vi "IMAQController.panel.vi"(0 "object ref":refnum<vi>, 5 "error in":errorcluster) -> ()   [LabVIEW 2014, in "IMAQController.lvlib"]
doc: "This is the front panel VI for the IMAQController class.\n\nThis program is free software; you can redistribute it and/or modify it under the terms of the GNU General Public License as published by the Free Software Foundation; either version 2 of the license, or (at your option) any later version.\n\nThis program is distributed in the hope that it will be useful, but WITHOUT ANY WARRANTY; without even the implied warranty of MERCHANTABILITY or FITNESS FOR A PARTICULAR PURPOSE. See the GNU General License for more details (http://www.gnu.org).\n\nLast update: 2-DEC-2010"
uses:
  IMAQController.lvlib
  CSlibraries-extern/DimLVEvent/LVDimInterface/LVDimInterface.lvlib
  CSlibraries-extern/DimLVEvent/LVDimInterface/LVDimInterface.dim service type.ctl
  CSCore/CSSystem/CSSystemLib/CSSystemLib.lvlib
  CSCore/BaseProcess/BaseProcess.lvlib
  CSlibraries-extern/DimLVEvent/DimIndicators/DimIndicators.lvlib
  CSPentatrap/_common/PTUtils/PTUtils.lvlib
  CSlibraries-extern/HGF/HGF_VisionTools/HGF_VisionTools.lvlib
  CSCore/CSObj/CSObj.lvlib
  CSlibraries-extern/DimLVEvent/LVDimInterface/LVDimInterface.dic_info_service_queue.vi
  CSCore/CSSystem/CoreLib/CoreLib.lvlib
  CSCore/CSSystem/CoreLib/CoreLib.short 2 byte array.vi
  <vilib>/Utility/error.llb/DialogType.ctl
  CSCore/CSSystem/CoreLib/CoreLib.int 2 byte array.vi
  CSCore/CSSystem/CoreLib/CoreLib.string 2 byte array.vi
  <vilib>/Utility/file.llb/Write To Spreadsheet File (DBL).vi
  <vilib>/Math Plots/3D Math Plots/3D Surface/3D Surface Datatype/3D Surface Datatype.lvclass
  <vilib>/Utility/file.llb/Write To Spreadsheet File (I64).vi
  <vilib>/Math Plots/3D Math Plots/3D Surface/3D Surface XCtrl/3D Surface.xctl
  <vilib>/Utility/config.llb/NI_LVConfig.lvlib
  <vilib>/Utility/config.llb/Read Key (Boolean).vi
  <vilib>/Utility/config.llb/Read Key (String).vi
  <vilib>/Utility/config.llb/Write Key (String).vi
  <vilib>/Math Plots/3D Math Plots/3D Surface/3D Surface Datatype/Public/Plot Helper (Vector).vi
  <vilib>/Math Plots/3D Math Plots/3D Plot/3D Plot Datatype/3D Plot Datatype.lvclass
  <vilib>/Utility/config.llb/Write Key (Boolean).vi
  <vilib>/event_ctls.llb/eventvkey.ctl
  CSlibraries-extern/DimLVEvent/DimIndicators/DimIndicators.anyType.ctl
panel:
  in  "ScanNamesArray":string[](array[string])
  in  "MeasurementNo":i32
  out "AnaWidth":i32
  out "AnaHeight":i32
  out "ScanRunning?":bool
  out "Progress bar":u8(slide) scale=0.0..100.0
  out "Last scan started":string
  out "ScanMin":dbl
  out "ActVerticalProj":dbl[][](array[numeric])
  out "ActHorizontalProj":dbl[][](array[numeric])
  in  "Delay (ms) Buffered":i32=2000
  out "SActStep":i32
  in  "Control Tab":T1(tab)
  in  "ROI Choice":enum32{"Radio Selection 1", "Radio Selection 2"}(radio)=enum."Radio Selection 2"
  in  "lower limit":dbl
  in  "auto repeat scan step":bool
  in  "Stop Scan button":bool
  in  "Pause Scan button":bool
  in  "Start Scan button":bool
  in  "Configure Scan button":bool
  in  "ROI2notROI1Boolen":bool
  in  "TL1x":i32 caption="x"
  in  "TL1y":i32 caption="y"
  in  "BR1x":i32 caption="x"
  in  "BR1y":i32 caption="y"
  in  "TL2x":i32 caption="x"
  in  "TL2y":i32 caption="y"
  in  "BR2x":i32 caption="x"
  in  "BR2y":i32 caption="y"
  in  "Clear ROIs button":bool
  out "ROI 2":dbl format="%.0e"
  out "ROI 1":dbl format="%.0e"
  out "ROI 1 / ROI 2":dbl format="%#.4g"
  in  "Offset":dbl
  in  "auto save":bool
  in  "Delay (ms)":i32=2000
  in  "Acquisition mode":T2(radio)
  in  "Network Transport":enum32{"Radio Selection 1", "Radio Selection 2"}(radio)
  in  "Image Settings":cluster{u8, u8}(slide)={0, 255} scale=0.0..255.0
  in  "Show Grid ?":bool=TRUE
  in  "Grid Color Box":u32(colorbox)=16448250
  in  "Save Path":path=path "D:/HitrapControlSystem/Camera-Pictures"
  in  "Overlay configured?":bool
  in  "Save this button":bool
  in  "Averaging":u8=1
  in  "Show all data":bool=TRUE
  in  "# shown Plots:":u8=3
  out "Intensity Scan":cluster{dbl[], dbl[]}[](graph)
  out "3D Surface":refnum<class "3D Plot Datatype.lvclass">[](xcontrol)
  out "ScanImage":T3(plugin-control)
  out "HilfsplotProj":cluster{i32[], dbl[]}[](graph)
  in  "Save Analysis button":bool
  in  "Analysis Mode":T4(ring)
  in  "Clear Analysis button":bool
  in  "Bug Report/ Feature Request - List":i32(listbox)
  in  "Send Button":bool
  out "Error OR":bool
  out "Error OL":bool
  out "Error UR":bool
  out "Error UL":bool
  out "Camera Choice error out":errorcluster
  out "NewVal":i32[](array[numeric])
  out "Overlay Lines":T5(array[cluster])
  out "SNofSteps":i32
  out "Image Arrived":i32
  out "Scan Image":i32
  out "Proj Up":i32
  out "AnaStep2":string
  out "AnaStep1":string
  out "AnaStep3":string
  out "BugFilePath":path
  out "ActDimensions":i16
  out "ScanValuesArray":dbl[](array[numeric])
  in  "CameraTimeStamps":dbl[](array[numeric])
  out "DIM Array":refnum<queue>[](array[refnum])
  out "Connection status":bool
  in  "Camera Choice":i32[](listbox)
  in  "Select Camera":u16(ring)
  in  "Camera\nConnected?":bool
  in  "Acquisition mode (Buffer)":T2(radio)
  in  "string":string
  in  "TestButton":bool
  out "ActImage RSelectionOn?":bool
  out "ActImage RMouse Down?":bool
  out "ActImage LSelectionOn?":bool
  out "ActImage LMouse Down?":bool
  out "Vertical chart XY":cluster{i32[], dbl[]}[](graph)
  out "Horizontal chart XY":cluster{i32[], dbl[]}[](graph)
  out "Error complete":bool
  out "Horizontal chart":dbl(graph)
  out "Time Stamp":timestamp format="%<%X\n%x>T"
  in  "Clear Log button":bool
  in  "Save Log button":bool
  in  "ActualImageLink(Compression Mode)":T6
  in  "Chart Auswertung-Strings":string
  out "Horiz/Vert Chart error out":errorcluster
  out "Horiz/Vert Chart Loop":i32
  out "Vertical chart":dbl[][](graph)
  out "Waveform Chart":dbl(graph)
  out "Act Image\nInformation":string
  out "Scan Image Pixel Value Loop error out":errorcluster
  out "Scan Pixel Value Loop":i32
  out "Scan Image\nInformation":string
  in  "stop button":bool
  out "Logger String":string
  out "Time Loop":i32
  in  "Analysis Image Settings":cluster{u8, u8}(slide)={0, 255} scale=0.0..255.0
  out "User Event error out":errorcluster
  out "User Event Loop":i32
  out "Send command error out":errorcluster
  out "DIM client error out":errorcluster
  out "Send Command Loop":i32
  out "DIM Client Loop":i32
  out "Analysis Event Loop":i32
  out "Asynch\nAna Data":i32
  out "TimeStamp Analyzer":i16[](array[numeric])
  out "Data Ana Synch?":bool
  out "TimeStamp Data":i16[](array[numeric])
  out "aktueller\nService":i32
  out "Image length":i32
  out "Image height":i32
  out "ActImage":T3(plugin-control)
  out "Analysis Event error out":errorcluster
  out "DIM service length / byte":i32
  out "no link":bool
  out "callBackID":i32
  # "Acquisition control"
  # "Scan control"
  # "Projections control"
  # "Image control"
  # "ROI 1"
  # "ROI 2"
  # "TL"
  # "BR"
  # "Integrated Pixel Values"
  # "Save Path"
  # "(no Analysis!)"
  # "Intensity Plot"
  # "Intensity Plot"
  # "Vertical Projection"
  # "position / mm"
  # "Horizontal Projection"
  # "position / mm"
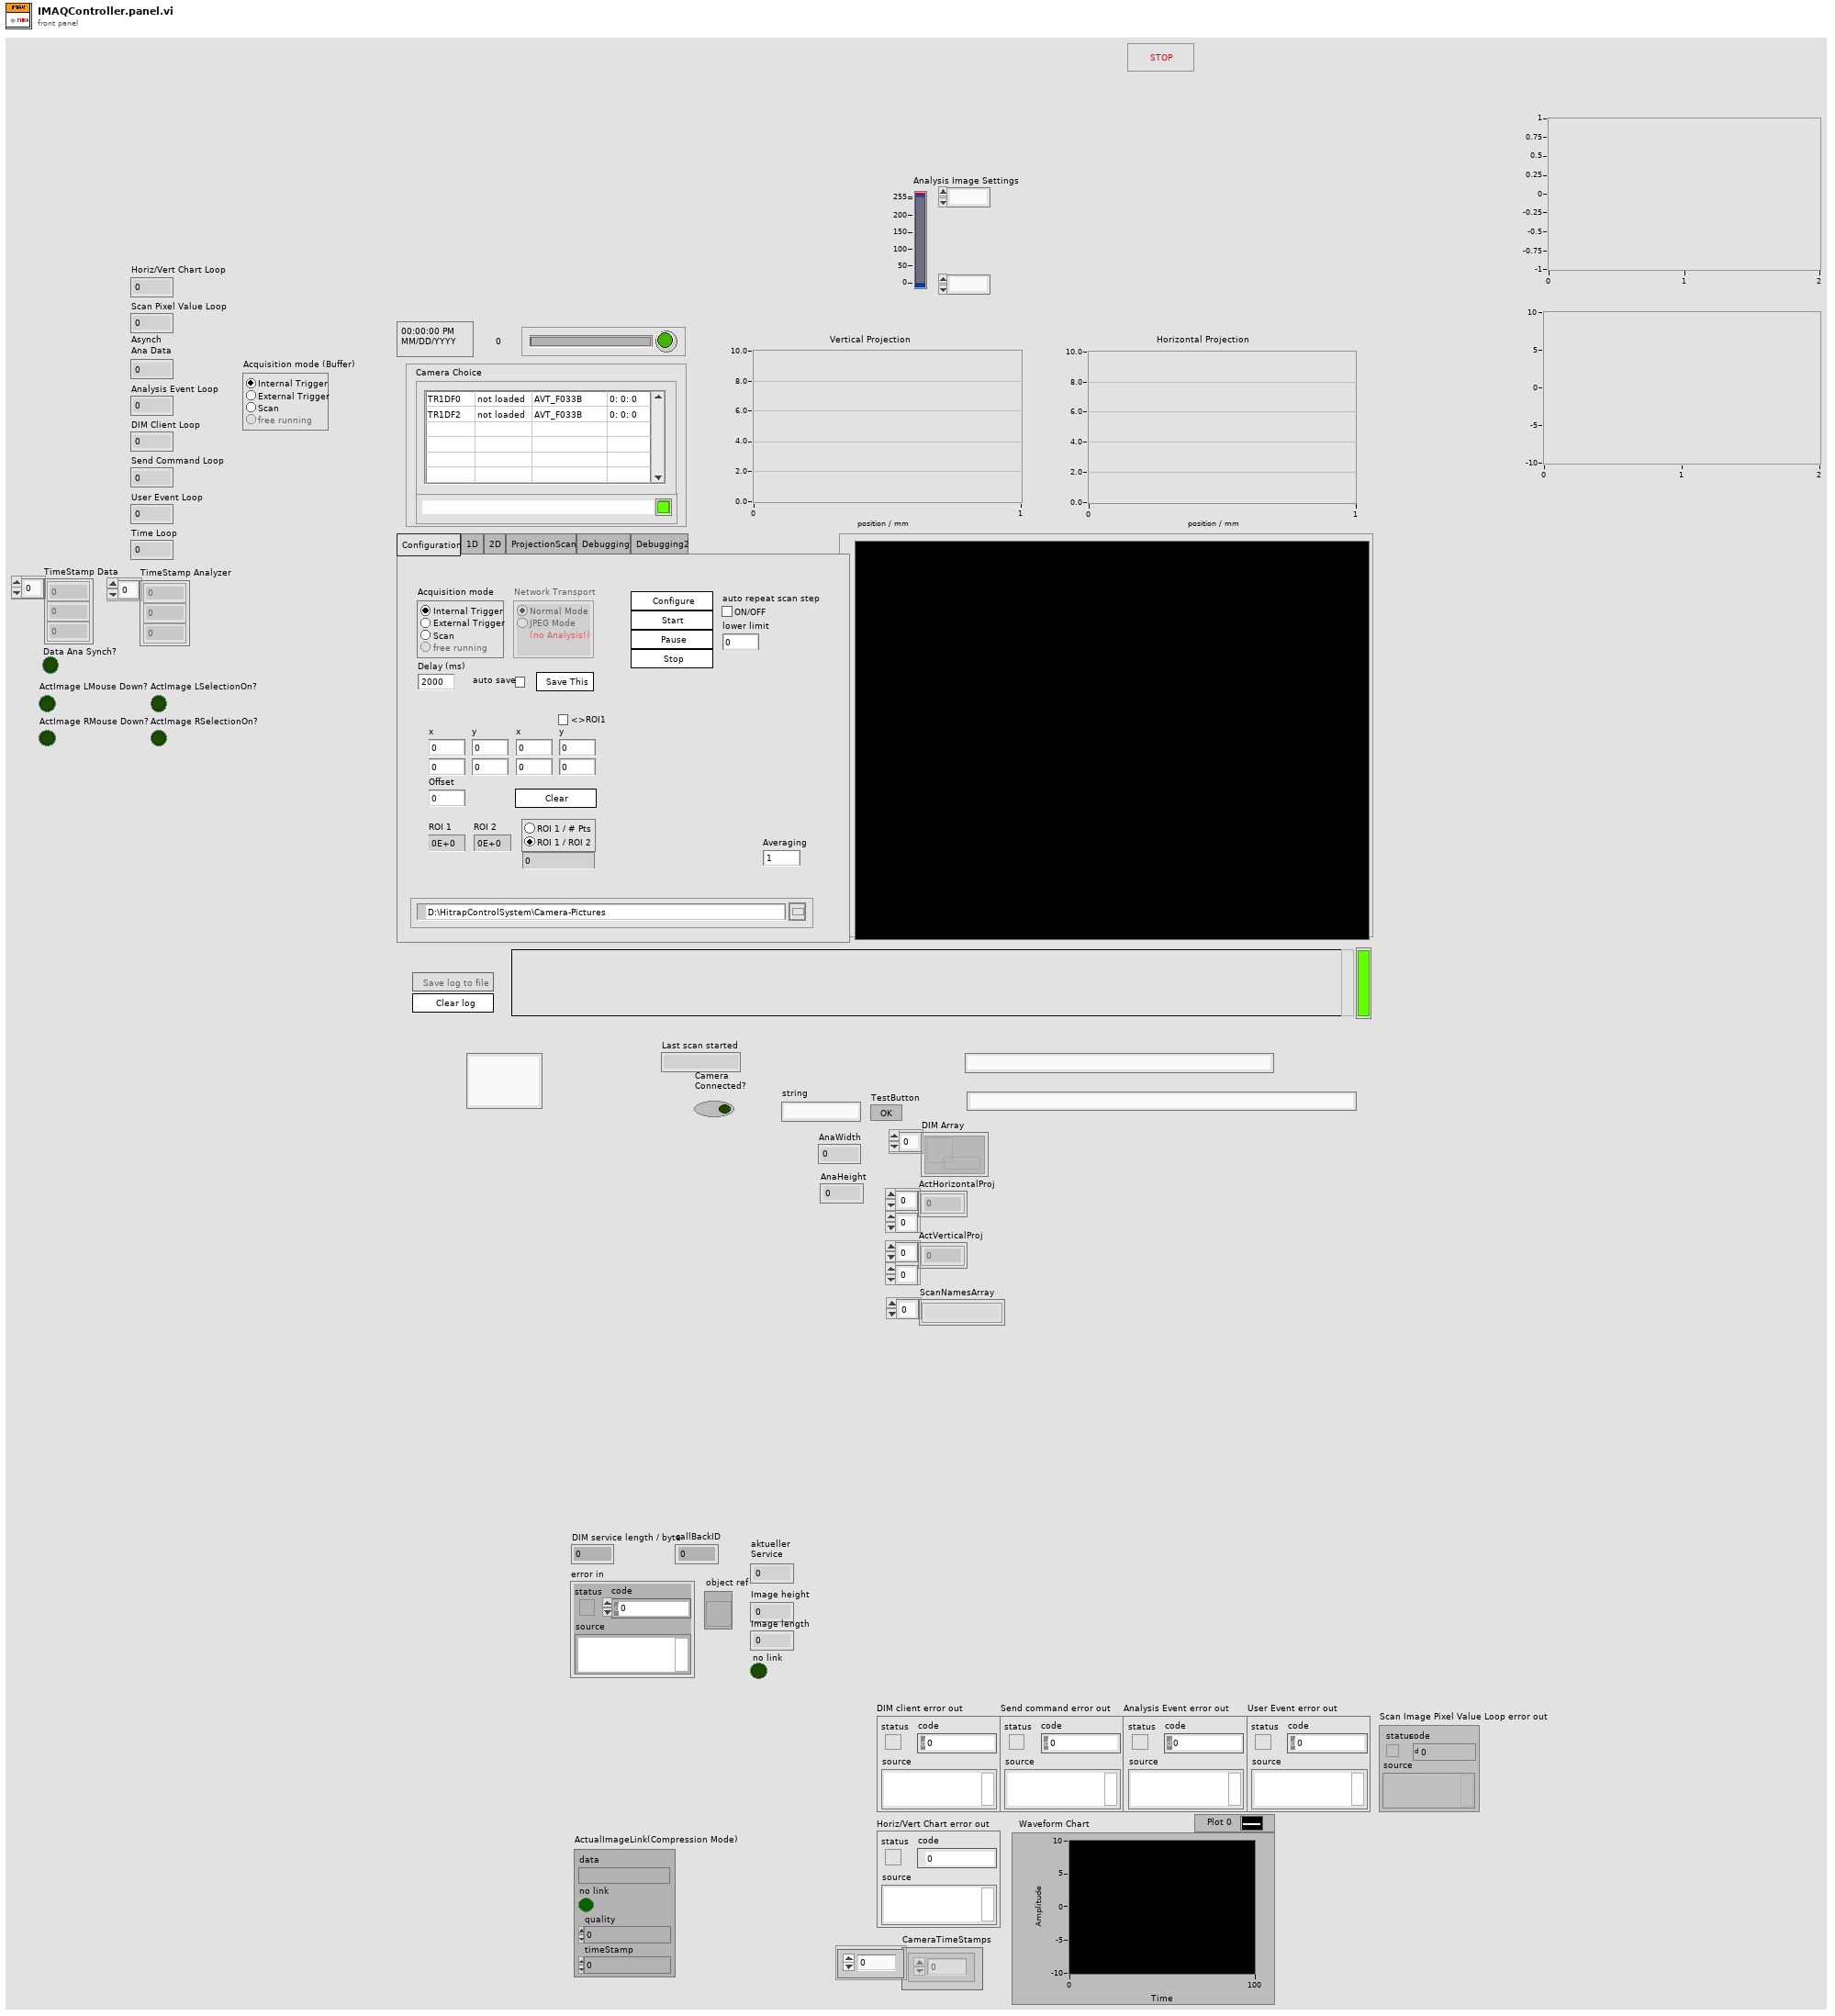
[diagram p1: front panel]
types:
  T1 = enum32{"Configuration", "1D", "2D", "ProjectionScan", "Debugging", "Debugging2"}
  T2 = enum32{"Internal Trigger", "Scan", "free Running", "External Trigger"}
  T3 = typedef "IMAQ Image.ctl" = refnum<image>
  T4 = enum16{"Horizontal Projection", "Vertical Projection"}
  T5 = cluster{cluster{"Horizontal":i32, "Vertical":i32}, cluster{"Horizontal":i32, "Vertical":i32}}[]
  T6 = typedef "DimIndicators.lvlib/DimIndicators.anyType.ctl" = cluster{"data":string, "no link":bool, "quality":i32, "timeStamp":dbl}
  T7 = cluster{"Message":string, "Error?":bool, "current time":timestamp, "MsgNo":i32}
  T8 = cluster{"Data":u8[][], "Height":i32, "Width":i32, "Save path out Horizontal":path, "Save path out Vertical":path}
  T9 = cluster{"Data":u8[][], "Height":i32, "Width":i32, "Save path out Scan":path, "Save path out Horizontal":path, "Save path out Vertical":path, "Scan?":bool, "Scan running?":bool, "ScanValuesArray":dbl[], "ActDimensions":i16, "ScanNamesArray":string[], "Av repeat?":bool}
  T10 = cluster{"Data":u8[][], "Height":i32, "Width":i32, "Save path out Scan":path, "Save path out Horizontal":path, "Save path out Vertical":path, "Scan?":bool, "Scan running?":bool, "ROI Calculation?":bool, "Starting Mouse Position 1":cluster{"X":i32, "Y":i32}, "End Mouse Position 1":cluster{"X":i32, "Y":i32}, "Starting Mouse Position 2":cluster{"X":i32, "Y":i32}, "End Mouse Position 2":cluster{"X":i32, "Y":i32}, "do analysis?":bool, "ScanValuesArray":dbl[], "ActDimensions":i16, "ScanNamesArray":string[], "Av repeat?":bool}
  T11 = typedef "DialogType.ctl" = u16
  T12 = cluster{"Message":string, "Error?":bool, "current time":timestamp}
  T13 = typedef "Image Type" = u32
  T14 = typedef "BaseProcess.lvlib/BaseProcess.i attribute.ctl" = cluster{"EventStatus":string, "EventError":i32, "PresetEvtWatchD":i32, "PresetPdcWatchD":i32, "EventTimeout":i32, "PeriodicInterval":i32, "Interface":string[], "Address":string[], "Special":string[], "PeriodicError":i32, "PeriodicStatus":string, "SuperProc":string, "Descriptors":T15[], "CaseRef":refnum<vi>, "PdcRef":refnum<vi>, "Thread Ref":refnum<vi>, "eventErrorID":i32, "eventStatusID":i32, "periodicErrorID":i32, "periodicStatusID":i32, "pdcCtrID":i32}
  T15 = typedef "BaseProcess.lvlib/BaseProcess.descriptor definition.ctl" = cluster{"selector":string, "descriptor":T16}
  T16 = typedef "BaseProcess.lvlib/BaseProcess.descriptor string definition.ctl" = string
  T17 = typedef "IMAQController.lvlib/IMAQController.i attribute.ctl" = cluster{"ImageTakenID":i32, "actSequencer":string, "actScanner":string, "CameraTriggerID":i32, "activatedCameras":cluster{"Name":string, "Camera Type":string, "Acquisition Mode":u32, "JPEG Mode?":bool, "Acquisition Delay":dbl, "Save Images?":bool, "Center Coordinates":T18, "PixelPermm":cluster{"Horizontal":dbl, "Vertical":dbl}, "Rotation":dbl, "Mirror Mode":u32, "PixelCoordinates":cluster{"1":cluster{"Horizontal":i32, "Vertical":i32}, "2":cluster{"Horizontal":i32, "Vertical":i32}, "3":cluster{"Horizontal":i32, "Vertical":i32}, "4":cluster{"Horizontal":i32, "Vertical":i32}}, "RWCoordinates":cluster{"1":cluster{"Horizontal":dbl, "Vertical":dbl}, "2":cluster{"Horizontal":dbl, "Vertical":dbl}, "3":cluster{"Horizontal":dbl, "Vertical":dbl}, "4":cluster{"Horizontal":dbl, "Vertical":dbl}}, "HorizScaling":dbl, "VertScaling":dbl}[], "Ini C-Array":string[], "actCamera":string, "activeCamera":cluster{"Name":string, "Camera Type":string, "Aqcuisation Mode":enum32{"Internal Trigger", "Scan", "free Running", "External Trigger"}, "JPEG Mode?":bool, "Acquisition Delay":dbl, "Save Images?":bool, "Center Coordinates":T18, "PixelPermm":cluster{"Horizontal":dbl, "Vertical":dbl}, "Rotation":dbl, "Mirror Mode":u32, "PixelCoordinates":cluster{"1":cluster{"Horizontal":i32, "Vertical":i32}, "2":cluster{"Horizontal":i32, "Vertical":i32}, "3":cluster{"Horizontal":i32, "Vertical":i32}, "4":cluster{"Horizontal":i32, "Vertical":i32}}, "RWCoordinates":cluster{"1":cluster{"Horizontal":dbl, "Vertical":dbl}, "2":cluster{"Horizontal":dbl, "Vertical":dbl}, "3":cluster{"Horizontal":dbl, "Vertical":dbl}, "4":cluster{"Horizontal":dbl, "Vertical":dbl}}, "HorizScaling":dbl, "VertScaling":dbl}, "BilderMittelungen":u8, "OldPicture":dbl[][]}
  T18 = typedef "LVPoint32TypeDef.ctl" = cluster{"Horizontal":i32, "Vertical":i32}
  T19 = cluster{"Name":string, "Camera Type":string, "Acquisition Mode":u32, "JPEG Mode?":bool, "Acquisition Delay":dbl, "Save Images?":bool, "Center Coordinates":T18, "PixelPermm":cluster{"Horizontal":dbl, "Vertical":dbl}, "Rotation":dbl, "Mirror Mode":u32, "PixelCoordinates":cluster{"1":cluster{"Horizontal":i32, "Vertical":i32}, "2":cluster{"Horizontal":i32, "Vertical":i32}, "3":cluster{"Horizontal":i32, "Vertical":i32}, "4":cluster{"Horizontal":i32, "Vertical":i32}}, "RWCoordinates":cluster{"1":cluster{"Horizontal":dbl, "Vertical":dbl}, "2":cluster{"Horizontal":dbl, "Vertical":dbl}, "3":cluster{"Horizontal":dbl, "Vertical":dbl}, "4":cluster{"Horizontal":dbl, "Vertical":dbl}}, "HorizScaling":dbl, "VertScaling":dbl}[]
  T20 = typedef "NI_LVConfig.lvlib/Config Data RefNum.ctl" = refnum<k1>
  T21 = enum8{"Enabled", "Disabled", "Disabled and Grayed Out"}
  T22 = typedef "LVDimInterface.lvlib/LVDimInterface.dim service type.ctl" = u16
  T23 = cluster{"Last scan started":string, "ScanValuesArray":dbl[], "ActDimensions":i16, "ScanNamesArray":string[]}
  T24 = cluster{"Name":string, "Color":u32, "Style":u8, "Point Style":u8, "Name Visible":bool, "Allow Drag":bool, "Annotation Mode":u32, "Plot":i32, "Index":i32, "Position":cluster{"X":dbl, "Y":dbl}, "X Scale":u32, "Y Scale":u32, "Show Arrow":bool, "Lock Name":bool, "Plot Area":i32, "Label Offset":cluster{"X":dbl, "Y":dbl}}
  T25 = cluster{"Name":string, "Color":u32, "Style":u8, "Point Style":u8, "Name Visible":bool, "Allow Drag":bool, "Annotation Mode":u32, "Plot":i32, "Index":i32, "Position":cluster{"X":dbl, "Y":dbl}, "X Scale":u32, "Y Scale":u32, "Show Arrow":bool, "Lock Name":bool, "Plot Area":i32, "Label Offset":cluster{"X":dbl, "Y":dbl}}[]
  T26 = typedef "CoreDefs.rawDataType.ctl" = i8[]
  T27 = typedef "LVAnnotationListTypeDef.ctl" = cluster{"Name":string, "Color":u32, "Style":u8, "Point Style":u8, "Name Visible":bool, "Allow Drag":bool, "Annotation Mode":u32, "Plot":i32, "Index":i32, "Position":cluster{"X":dbl, "Y":dbl}, "X Scale":u32, "Y Scale":u32, "Show Arrow":bool, "Lock Name":bool, "Plot Area":i32, "Label Offset":cluster{"X":dbl, "Y":dbl}}[]
  T28 = cluster{"Message":string, "Error?":bool, "current time":timestamp, "Msg#":i32}
  T29 = cluster{"Message":string, "Error?":bool, "current time":timestamp, "MsgNo":i32}[]
  T30 = typedef "eventvkey.ctl" = enum16{"ASCII", "Enter", "Return", "Shift", "Ctrl", "Alt", "Cmd", "Opt", "Caps", "NumLock", "Clear", "Break", "Up", "Down", "Left", "Right", "Insert", "Delete", "Home", "End", "PageUp", "PageDown", "Escape", "Help", "Pause", "ScrollLock", "F1", "F2", "F3", "F4", "F5", "F6", "F7", "F8", "F9", "F10", "F11", "F12", "F13", "F14", "F15", "F16", "F17", "F18", "F19", "F20", "F21", "F22", "F23", "F24", "Play", "VolumeUp", "VolumeDown", "Mute", "Two Byte Char"}
  T31 = enum32{"Gray", "Binary", "Gradient", "Rainbow", "Temperature"}
  T32 = cluster{"Name":string, "Camera Type":string, "Acquisition Mode":u32, "JPEG Mode?":bool, "Acquisition Delay":dbl, "Save Images?":bool, "Center Coordinates":T18, "PixelPermm":cluster{"Horizontal":dbl, "Vertical":dbl}, "Rotation":dbl, "Mirror Mode":u32, "PixelCoordinates":cluster{"1":cluster{"Horizontal":i32, "Vertical":i32}, "2":cluster{"Horizontal":i32, "Vertical":i32}, "3":cluster{"Horizontal":i32, "Vertical":i32}, "4":cluster{"Horizontal":i32, "Vertical":i32}}, "RWCoordinates":cluster{"1":cluster{"Horizontal":dbl, "Vertical":dbl}, "2":cluster{"Horizontal":dbl, "Vertical":dbl}, "3":cluster{"Horizontal":dbl, "Vertical":dbl}, "4":cluster{"Horizontal":dbl, "Vertical":dbl}}, "HorizScaling":dbl, "VertScaling":dbl}
  T33 = cluster{"SystemName":string, "Camera-Name":string[]}[]
  T34 = typedef "LVDateTimeRec.ctl" = cluster{"fractional second":dbl, "second":i32, "minute":i32, "hour":i32, "day of month":i32, "month":i32, "year":i32, "day of week":i32, "day of year":i32, "DST":i32}
  T35 = cluster{"Name":string, "CSObject Name":string, "Camera Type":string, "Hardware Address":string, "Acquisition Mode":u32, "JPEG Mode?":bool, "Acquisition Delay":dbl, "Save Images?":bool, "Center Coordinates":T18, "PixelPermm":cluster{"Horizontal":dbl, "Vertical":dbl}, "Rotation":dbl, "Mirror Mode":u32, "PixelCoordinates":cluster{"1":cluster{"Horizontal":i32, "Vertical":i32}, "2":cluster{"Horizontal":i32, "Vertical":i32}, "3":cluster{"Horizontal":i32, "Vertical":i32}, "4":cluster{"Horizontal":i32, "Vertical":i32}}, "RWCoordinates":cluster{"1":cluster{"Horizontal":dbl, "Vertical":dbl}, "2":cluster{"Horizontal":dbl, "Vertical":dbl}, "3":cluster{"Horizontal":dbl, "Vertical":dbl}, "4":cluster{"Horizontal":dbl, "Vertical":dbl}}, "HorizScaling":dbl, "VertScaling":dbl}[]
  T36 = cluster{"Name":string, "CSObject Name":string, "Camera Type":string, "Hardware Address":string, "Acquisition Mode":u32, "JPEG Mode?":bool, "Acquisition Delay":dbl, "Save Images?":bool, "Center Coordinates":T18, "PixelPermm":cluster{"Horizontal":dbl, "Vertical":dbl}, "Rotation":dbl, "Mirror Mode":u32, "PixelCoordinates":cluster{"1":cluster{"Horizontal":i32, "Vertical":i32}, "2":cluster{"Horizontal":i32, "Vertical":i32}, "3":cluster{"Horizontal":i32, "Vertical":i32}, "4":cluster{"Horizontal":i32, "Vertical":i32}}, "RWCoordinates":cluster{"1":cluster{"Horizontal":dbl, "Vertical":dbl}, "2":cluster{"Horizontal":dbl, "Vertical":dbl}, "3":cluster{"Horizontal":dbl, "Vertical":dbl}, "4":cluster{"Horizontal":dbl, "Vertical":dbl}}, "HorizScaling":dbl, "VertScaling":dbl}
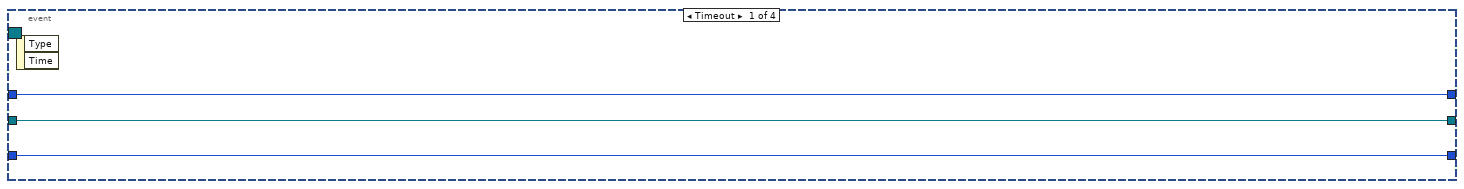
[diagram p2: hidden frame]
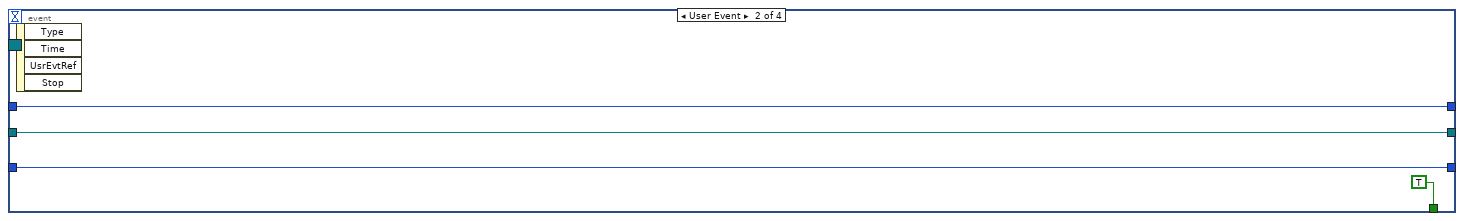
[diagram p3: hidden frame]
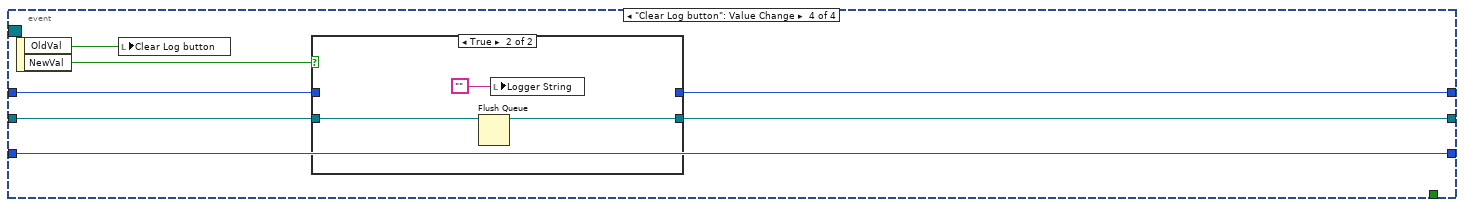
[diagram p4: hidden frame]
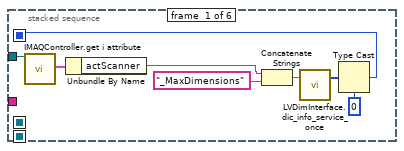
[diagram p6: hidden frame]
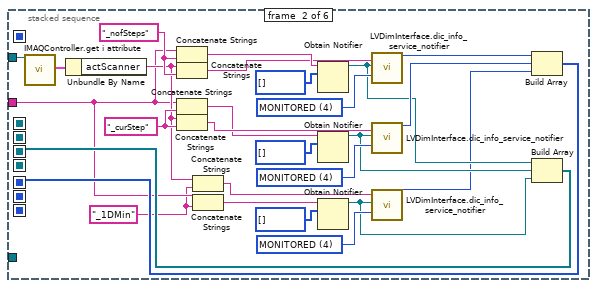
[diagram p7: hidden frame]
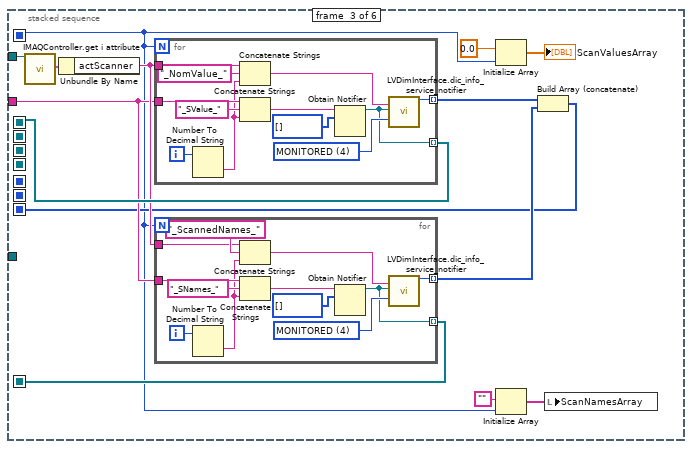
[diagram p8: hidden frame]
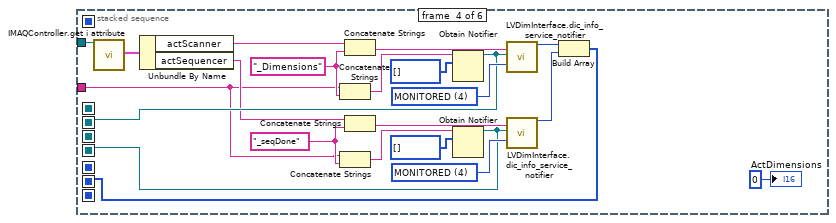
[diagram p9: hidden frame]
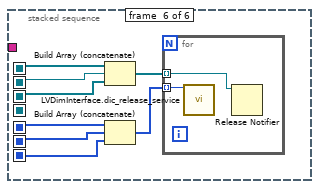
[diagram p18: hidden frame]
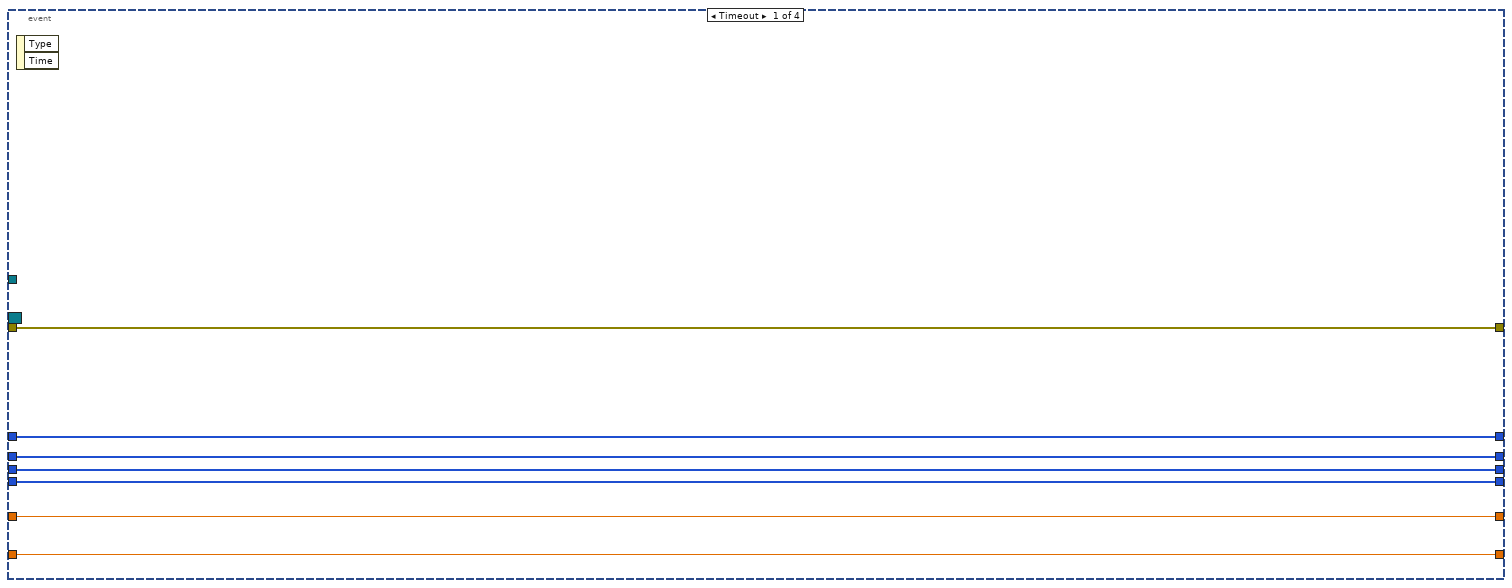
[diagram p19: hidden frame]
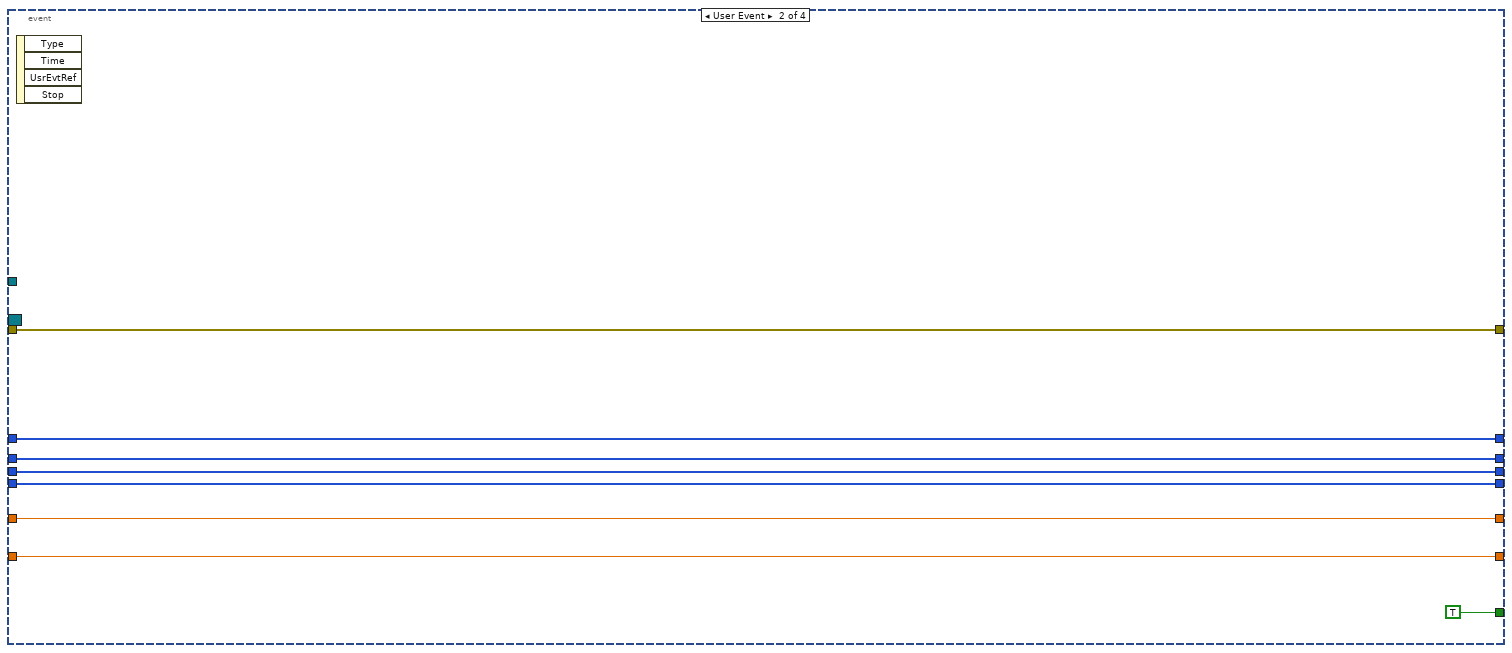
[diagram p20: hidden frame]
diagram:
  w2 = refnum<class "3D Plot Datatype.lvclass">[] []  # 2D Plot Class
  w24 = 0.0  # Previous x-Value
  w25 = dbl[][] []  # ScanGraphZ
  w27 = 0  # Msg#
  w28 = T7 {"Message"="", "Error?"=TRUE, "current time"=timestamp(0 s since 1904-01-01), "MsgNo"=0}  # Logger String
  w31 = 100  # Max Logger Size
  w40 = T8 {"Data"=[], "Height"=0, "Width"=0, "Save path out Horizontal"=path "", "Save path out Vertical"=path ""}  # Analysis Step 3
  w45 = TRUE  # AnaOn?
  w44 = T9 {"Data"=[], "Height"=0, "Width"=0, "Save path out Scan"=path "", "Save path out Horizontal"=path "", "Save path out Vertical"=path "", "Scan?"=TRUE, "Scan running?"=TRUE, "ScanValuesArray"=[], "ActDimensions"=0, "ScanNamesArray"=[], "Av repeat?"=FALSE}  # Analysis Step 1
  w43 = T10 {"Data"=[], "Height"=0, "Width"=0, "Save path out Scan"=path "", "Save path out Horizontal"=path "", "Save path out Vertical"=path "", "Scan?"=TRUE, "Scan running?"=TRUE, "ROI Calculation?"=TRUE, "Starting Mouse Position 1"={"X"=0, "Y"=0}, "End Mouse Position 1"={"X"=0, "Y"=0}, "Starting Mouse Position 2"={"X"=0, "Y"=0}, "End Mouse Position 2"={"X"=0, "Y"=0}, "do analysis?"=TRUE, "ScanValuesArray"=[], "ActDimensions"=0, "ScanNamesArray"=[], "Av repeat?"=FALSE}  # Analysis Step 2
  w47 = TRUE  # DeleteAnaOfLastStep
  w59 = 0  # AnaCounter
  w61 = 0  # MaxProjectionH
  w62 = i32[][] []  # Analysis Data Hor
  w70 = FALSE  # Paused scan?
  w72 = TRUE  # SequenceDone?
  w75 = TRUE  # CameraChange?
  w95 = FALSE  # Is maybe a bit better
  w113 = TRUE  # NewScan?
  w115 = dbl[] []  # ScanGraphY
  w116 = dbl[] []  # ScanGraphX
  w117 = u32 5 items=["Grayscale", "Binary", "Gradient", "Rainbow", "Temperature", "User Defined"] ("Palette:Palette Type")
  w119 = cluster{"X":i32, "Y":i32} {"X"=0, "Y"=0}  # End Mouse Position 2
  w118 = cluster{"X":i32, "Y":i32} {"X"=0, "Y"=0}  # Starting Mouse Position 2
  w120 = cluster{"X":i32, "Y":i32} {"X"=0, "Y"=0}  # End Mouse Position 1
  (unwired) TRUE  # NewImage?
  w127 = cluster{"X":i32, "Y":i32} {"X"=0, "Y"=0}  # Starting Mouse Position 1
  w128 = 0.0  # Vertical YMax
  w129 = 0.0  # Horizontal YMax
  w131 = i32[] []  # 2nd last values
  w133 = 0  # Cancel error
  w135 = FALSE  # active error
  w136 = T11 2 items=["no dialog", "OK message", "continue or stop message", "OK message + warnings", "continue/stop + warnings"] ("type of dialog (OK msg:1)")
  w138 = i32[] []  # last values
  w146 = T12 {"Message"="", "Error?"=TRUE, "current time"=timestamp(0 s since 1904-01-01)}  # Logger Update
  w154 = FALSE  # Stop
  w167 = 0  # MaxProjectionV
  w168 = i32[][] []  # Analysis Data Ver
  w166 = u32 3 items=["Grayscale", "Binary", "Gradient", "Rainbow", "Temperature", "User Defined"] ("Palette:Palette Type")
  w63 = T13 0 items=["Grayscale (U8)", "Grayscale (I16)", "Grayscale (SGL)", "Complex (CSG)", "RGB (U32)", "HSL (U32)", "RGB (U64)", "Grayscale (U16)"] ("Image Type")
  w175 = i16[] []
  w177 = FALSE  # alle daten gelesen?
  w178 = FALSE  # event  occured?
  # "This loop calculates the lifetime of cameras in the \"camera choice\" list\nIt uses right now \"get service once\" which is not the best solution"
  # "This is a workaround for\na very strange error"
  # "macht noch wenig Sinn, da\nFP sofort geschlossen wird, bevor man \ndie Fehler sehen kann"
  n1 = call "CSSystemLib.ref2name.vi"("obj refnum"="object ref") -> ("name"=w32:string)
  n2 = call "IMAQController.InitPanel.vi"("i ref in"="object ref", "error in"="error in") -> ("i ref out"=w56:refnum<vi>, "Camera Config Array"=w76:string[][], "actCameras"=w90:i32[], "error out"=w85:errorcluster)  [unwired: 14 in]
  n3 = property on="Camera Choice" class="MCListbox (strict)"(error in=w85, "Value"=w90) -> (error out=w57:errorcluster)  [unwired: 1 in, 1 out]
  n4 = for {
    tunnel: [w182] -> w77 mode=indexing
    tunnel: w76 -> [w183] mode=indexing
    n5 = Replace Array Subset(array=w183, new element="not loaded" ("new element/subarray"), index=1) -> (w182:string[])
  }
  n6 = Get Date/Time In Seconds() -> (seconds since 1Jan1904=w84:timestamp)
  n7 = call "BaseProcess.get i attribute.vi"("i ref in"=w56, "error in (no error)"=w57) -> ("i ref out"=w58:refnum<vi>, "i attribute"=w54:T14, "error out"=w55:errorcluster)  [unwired: 15 in]
  n8 = To Double Precision Float(number=w84) -> (double precision float=w83:dbl)
  n9 = Unbundle By Name(w54) -> ("Special"=w53:string[])
  n10 = call "IMAQController.SortActivatedCameraArray.vi"("i ref in"=w58, "error in (no error)"=w55) -> ("i ref out"=w82:refnum<vi>, "error out"=w81:errorcluster)  [unwired: 16 in]
  n11 = Index Array(array=w53, index #1=3 ("index")) -> (element #1=w51:string, element #2=w18:string)  [unwired: 1 in]
  n12 = call "IMAQController.get i attribute.vi"("i ref in"=w82, "error in (no error)"=w81) -> ("i ref out"=w97:refnum<vi>, "i attribute"=w171:T17, "error out"=w87:errorcluster)  [unwired: 15 in]
  n13 = for {
    tunnel: w90 -> [w185] mode=indexing
    tunnel: w76 -> [w219]
    shift-right: [w215] -> w88
    shift-left: dbl[] [] ("CameraTimeStamps") -> [w216]
    tunnel: w87 -> [w217]
    tunnel: [w217] -> w16
    shift-right: [w187] -> w86
    shift-left: w77 -> [w199]
    tunnel: w83 -> [w197]
    w207 = ":" ("string")
    w193 = "Camera_" ("string")
    n14 = Index Array(array=w219, index (row)=w185, index (col)=0 ("disabled index (col)")) -> (element=w192:string)
    n15 = Concatenate Strings(w193, w192, "_CameraType" ("string")) -> (w195:string)
    n16 = Concatenate Strings(w193, w192, "_birthday" ("string")) -> (w220:string)
    n17 = call "LVDimInterface.dic_info_service_once.vi"("serviceName"=w195) -> ("data"=w194:i8[])  [unwired: 15 in, 3 out]
    n18 = call "LVDimInterface.dic_info_service_once.vi"("serviceName"=w220) -> ("data"=w223:i8[])  [unwired: 15 in, 3 out]
    n19 = Type Cast(x=w194) -> (*(type *) &x=w190:string)  [unwired: 1 in]
    n20 = Type Cast(type=0.0, x=w223) -> (*(type *) &x=w198:dbl)
    n21 = Subtract(x=w197, y=w198) -> (x-y=w200:dbl)
    n22 = Quotient & Remainder(x=w200, y=3600.0) -> (x-y*floor(x/y)=w210:dbl, floor(x/y)=w208:dbl)
    n23 = Quotient & Remainder(x=w210, y=60.0) -> (x-y*floor(x/y)=w206:dbl, floor(x/y)=w201:dbl)
    n24 = Number To Decimal String(number=w208) -> (decimal integer string=w209:string)  [unwired: 1 in]
    n25 = Number To Decimal String(number=w201, width (-)=i16 2) -> (decimal integer string=w202:string)
    n26 = Number To Decimal String(number=w206, width (-)=i16 2) -> (decimal integer string=w205:string)
    n27 = Build Array (concatenate)(w216, w198) -> (w215:dbl[])
    n28 = Concatenate Strings(w209, w207, w202, w207, w205) -> (w214:string)
    n29 = Replace Array Subset(array=w199, new element=w214, index (row)=w185, index (col)=3 ("disabled index (col)")) -> (w191:string[][])
    n30 = Replace Array Subset(array=w191, new element=w190, index (row)=w185, index (col)=2 ("disabled index (col)")) -> (w188:string[][])
    n31 = Replace Array Subset(array=w188, new element="loaded" ("new element/subarray"), index (row)=w185, index (col)=1 ("disabled index (col)")) -> (w187:string[][])
  }
  n32 = String To Path(string=w51) -> (path=w50:path)
  n33 = String To Path(string=w18) -> (path=w17:path)
  "BugFilePath" <- w17
  n34 = local write "Save Path"(w50) -> ()
  n35 = Unbundle By Name(w171) -> ("actCamera"=w22:string, "activatedCameras"=w111:T19)
  n36 = call <vilib>:"Open Config Data.vi"("error in (no error)"=w16, "configuration file path"=w17) -> ("error out"=w14:errorcluster, "refnum"=w15:T20)  [unwired: 7 in, 1 out]
  n37 = call <vilib>:"Get Section Names.vi"("error in (no error)"=w14, "refnum"=w15) -> ("error out"=w12:errorcluster, "section names"=w13:string[], "refnum out"=w9:T20)  [unwired: 7 in]
  n38 = for {
    tunnel: w13 -> [w234] mode=indexing
    tunnel: w9 -> [w248]
    shift-right: [w233] -> w11
    shift-left: w12 -> [w249]
    tunnel: [w224] -> w8 mode=indexing
    n39 = call-poly <vilib>:"Read Key.vi"("section"=w234, "error in (no error)"=w249, "key"="B?", "refnum"=w248) -> ("error out"=w246:errorcluster, "value"=w232:bool, "refnum out"=w247:T20)  [unwired: 4 in, 1 out]
    n40 = Select(t="B", s=w232, f="F") -> (s? t:f=w229:string)
    n41 = call-poly <vilib>:"Read Key.vi"("section"=w234, "error in (no error)"=w246, "key"="Date", "refnum"=w247) -> ("error out"=w237:errorcluster, "value"=w228:string, "refnum out"=w239:T20)  [unwired: 4 in, 1 out]
    n42 = call-poly <vilib>:"Read Key.vi"("section"=w234, "error in (no error)"=w237, "key"="User", "refnum"=w239) -> ("error out"=w235:errorcluster, "value"=w227:string, "refnum out"=w236:T20)  [unwired: 4 in, 1 out]
    n43 = call-poly <vilib>:"Read Key.vi"("section"=w234, "error in (no error)"=w235, "key"="Topic", "refnum"=w236) -> ("error out"=w244:errorcluster, "value"=w226:string, "refnum out"=w245:T20)  [unwired: 4 in, 1 out]
    n44 = call-poly <vilib>:"Read Key.vi"("section"=w234, "error in (no error)"=w244, "key"="Desc", "refnum"=w245) -> ("error out"=w233:errorcluster, "value"=w225:string)  [unwired: 4 in, 2 out]
    n45 = Build Array(w229, w228, w227, w226, w225) -> (w224:string[])
  }
  n46 = for {
    tunnel: [w251] -> w80 mode=indexing
    tunnel: w111 -> [w253] mode=indexing
    tunnel: [w250] -> w23 mode=indexing
    n47 = Unbundle By Name(w253) -> ("Name"=w250:string)
    n48 = Concatenate Strings("HITRAP " ("string"), w250) -> (w251:string)
  }
  n49 = local write "CameraTimeStamps"(w88) -> ()
  n50 = property on="Camera Choice" class="MCListbox (strict)"("ItemNames"=w86) -> ()  [unwired: 2 in, 2 out]
  n51 = Search 1D Array(1D array=w23, element=w22) -> (index of element=w19:i32)  [unwired: 1 in]
  n52 = call <vilib>:"Close Config Data.vi"("error in (no error)"=w11, "refnum"=w9) -> ("error out"=w10:errorcluster)  [unwired: 8 in, 1 out]
  n53 = Concatenate Strings(w32, "_actualImage" ("string")) -> (w174:string)
  n54 = Concatenate Strings(w32, "_ScanImage" ("string")) -> (w169:string)
  n55 = Concatenate Strings(w32, "_actualImageRAW" ("string")) -> (w126:string)
  n56 = Concatenate Strings(w32, "_actualSaveImage" ("string")) -> (w68:string)
  n57 = call "IMAQ Create"("Image Name"=w174, "Image Type"=w63, "error in (no error)"=w10) -> ("New Image"=w172:T3, "error out"=w163:errorcluster)  [unwired: 2 in]
  n58 = call "IMAQ Create"("Image Name"=w169, "Image Type"=w63, "error in (no error)"=w163) -> ("New Image"=w60:T3, "error out"=w124:errorcluster)  [unwired: 2 in]
  n59 = call "IMAQ Create"("Image Name"=w126, "Image Type"=w63, "error in (no error)"=w124) -> ("New Image"=w69:T3, "error out"=w66:errorcluster)  [unwired: 2 in]
  n60 = call "IMAQ Create"("Image Name"=w68, "Image Type"=w63, "error in (no error)"=w66) -> ("New Image"=w64:T3, "error out"=w65:errorcluster)  [unwired: 2 in]
  n61 = property on="ScanImage"(error in=w65, "Palette Type"=w166) -> (error out=w162:errorcluster)  [unwired: 1 in, 1 out]
  n62 = property on="ActImage"(error in=w162, "Palette Type"=w117) -> (error out=w161:errorcluster)  [unwired: 1 in, 1 out]
  n63 = property on="ScanImage"(error in=w161, "Zoom to Fit Mode"=FALSE) -> (error out=w160:errorcluster)  [unwired: 1 in, 1 out]
  n64 = property on="ActImage"(error in=w160, "Zoom to Fit Mode"=w95) -> (error out=w130:errorcluster)  [unwired: 1 in, 1 out]
  n65 = Initialize Array("", 5 ("dimension size")) -> (w6:string[])
  n66 = property on="Select Camera" class="Ring (strict)"(error in=w130, "Strings []"=w80) -> (error out=w20:errorcluster)  [unwired: 1 in, 1 out]
  n67 = Build Array (concatenate)(w8, w6) -> (w7:string[][])
  n68 = property on="Bug Report/ Feature Request - List" class="MCListbox (strict)"("ItemNames"=w7) -> ()  [unwired: 2 in, 2 out]
  n69 = property on="Select Camera" class="Ring (strict)"(error in=w20, "Value"=w19) -> (error out=w21:errorcluster)  [unwired: 1 in, 1 out]
  n70 = stacked-sequence {
    seq-local: [_ _ _ w289 _ _] -> [_ _ _ _ w300 _]
    seq-local: [w260 _ _ _ _ _] -> [_ w268 _ _ _ _]
    seq-local: [_ w271 _ _ _ _] -> [_ _ _ w298 _ _]
    tunnel: [_ _ _ _ w302 _] -> w100
    tunnel: w21 -> [w266 _ _ _ _ _]
    tunnel: [_ _ _ _ w303 _] -> w101
    tunnel: w22 -> [_ _ _ _ w301 _]
    frame #0 {
      w257 = T2."Internal Trigger" ("Acquisition mode")
      w256 = T21."Disabled and Grayed Out" ("Disabled")
      n71 = property on="Network Transport" class="RadioBtnsControl (strict)"(error in=w266, "DisabledEnum"=w256) -> (error out=w265:errorcluster)  [unwired: 1 in, 1 out]
      n72 = local write "Acquisition mode"(w257) -> ()
      n73 = local write "Network Transport"(enum32{"Radio Selection 1", "Radio Selection 2"}."Radio Selection 1" ("Network Transport")) -> ()
      n74 = property on="Acquisition mode" class="RadioBtnsControl (strict)"(error in=w265, "DisabledEnum"=T21."Enabled" ("Disabled")) -> (error out=w254:errorcluster)  [unwired: 1 in, 1 out]
      n75 = local write "Acquisition mode (Buffer)"(w257) -> ()
      n76 = property on="Start Scan button" class="Bool"(error in=w254, "DisabledEnum"=w256) -> (error out=w264:errorcluster)  [unwired: 1 in, 1 out]
      n77 = property on="Pause Scan button" class="Bool"(error in=w264, "DisabledEnum"=w256) -> (error out=w263:errorcluster)  [unwired: 1 in, 1 out]
      n78 = property on="Stop Scan button" class="Bool"(error in=w263, "DisabledEnum"=w256) -> (error out=w262:errorcluster)  [unwired: 1 in, 1 out]
      n79 = property on="Progress bar" class="Slide (strict)"(error in=w262, "DisabledEnum"=T21."Enabled" ("Disabled")) -> (error out=w261:errorcluster)  [unwired: 1 in, 1 out]
      n80 = property on="Logger String" class="Str"(error in=w261, "Text.Scroll Position"=u32 4294967295) -> (error out=w260:errorcluster)  [unwired: 1 in, 1 out]
    }
    frame #1 {
      w269 = u32 12040119
      w270 = u32 2 ("Active Plot")
      w274 = u32 6776679
      w275 = u32 0
      w276 = u32 1 ("Active Plot")
      w277 = u32 0 ("Active Plot")
      n81 = property on="Horizontal chart XY" class="XYGraph (strict)"(error in=w268, "Active Plot"=w277, "Plot.Plot Color"=w275) -> (error out=w278:errorcluster)  [unwired: 1 in, 1 out]
      n82 = property on="Horizontal chart XY" class="XYGraph (strict)"(error in=w278, "Active Plot"=w276, "Plot.Plot Color"=w274) -> (error out=w279:errorcluster)  [unwired: 1 in, 1 out]
      n83 = property on="Vertical chart XY" class="XYGraph (strict)"(error in=w279, "Active Plot"=w277, "Plot.Plot Color"=w275) -> (error out=w280:errorcluster)  [unwired: 1 in, 1 out]
      n84 = property on="Vertical chart XY" class="XYGraph (strict)"(error in=w280, "Active Plot"=w276, "Plot.Plot Color"=w274) -> (error out=w273:errorcluster)  [unwired: 1 in, 1 out]
      n85 = property on="Horizontal chart XY" class="XYGraph (strict)"(error in=w273, "Active Plot"=w270, "Plot.Plot Color"=w269) -> (error out=w272:errorcluster)  [unwired: 1 in, 1 out]
      n86 = property on="Vertical chart XY" class="XYGraph (strict)"(error in=w272, "Active Plot"=w270, "Plot.Plot Color"=w269) -> (error out=w271:errorcluster)  [unwired: 1 in, 1 out]
      n87 = Wait Until Next ms Multiple(millisecond multiple=u32 200) -> ()  [unwired: 1 out]
    }
    frame #2 {
      n88 = property on="Intensity Scan" class="XYGraph (strict)"("Active Plot"=u32 0, "Plot.Plot Color"=u32 0) -> ()  [unwired: 2 in, 2 out]
      n89 = property on="Intensity Scan" class="XYGraph (strict)"("Active Plot"=u32 1, "Plot.Plot Color"=u32 6776679) -> ()  [unwired: 2 in, 2 out]
      n90 = property on="Intensity Scan" class="XYGraph (strict)"("Active Plot"=u32 2, "Plot.Plot Color"=u32 12040119) -> ()  [unwired: 2 in, 2 out]
    }
    frame #3 {
      w294 = FALSE ("ActImage Mouse Down?")
      w295 = FALSE ("ActImage Mouse Down?")
      w296 = -2.0 ("Cursor.Cursor Position:Cursor Y")
      w297 = u32 0 ("Active Cursor")
      n91 = property on="Horizontal chart XY" class="XYGraph (strict)"(error in=w298, "Active Cursor"=w297, "Cursor.Cursor Y"=w296) -> (error out=w299:errorcluster)  [unwired: 1 in, 1 out]
      n92 = property on="Vertical chart XY" class="XYGraph (strict)"(error in=w299, "Active Cursor"=w297, "Cursor.Cursor Y"=w296) -> (error out=w291:errorcluster)  [unwired: 1 in, 1 out]
      n93 = local write "Camera\nConnected?"(TRUE ("Camera\nConnected?")) -> ()
      n94 = local write "Overlay configured?"(FALSE ("OverlayAlreadyConfigured?")) -> ()
      n95 = call "ColorMap_Rainbow_LH.vi"("Limits (L:0,H:255)"="Image Settings") -> ("Rainbow_LH"=w292:cluster{"Red":u8, "Green":u8, "Blue":u8}[])
      n96 = property on="ActImage"(error in=w291, "User Palette"=w292) -> (error out=w289:errorcluster)  [unwired: 1 in, 1 out]
      "ActImage LMouse Down?" <- w295
      "ActImage LSelectionOn?" <- w295
      "ActImage RSelectionOn?" <- w294
      "ActImage RMouse Down?" <- w294
    }
    frame #4 {
      # "DIM Indicators are not stable enough to\nread them out here..."
      n97 = Concatenate Strings(w301, "_NumberOfImages" ("string")) -> (w304:string)
      n98 = call "LVDimInterface.dic_info_service_once.vi"("serviceName"=w304, "error in (no error)"=w300) -> ("data"=w307:i8[], "error out"=w302:errorcluster)  [unwired: 14 in, 2 out]
      n99 = Type Cast(type=u16 0 ("data"), x=w307) -> (*(type *) &x=w303:u16)
    }
    frame #5 {
      w308 = T21."Disabled and Grayed Out" ("Disabled")
      n100 = property on="Connection status" class="Bool (strict)"("TipStrip"="") -> ()  [unwired: 2 in, 2 out]
      n101 = local write "Delay (ms) Buffered"("Delay (ms)") -> ()
      n102 = property on="Configure Scan button" class="Bool"("DisabledEnum"=T21."Enabled" ("Disabled")) -> ()  [unwired: 2 in, 2 out]
      n103 = property on="auto repeat scan step" class="Bool (strict)"("DisabledEnum"=w308) -> ()  [unwired: 2 in, 2 out]
      n104 = property on="lower limit" class="DigNum (strict)"("DisabledEnum"=w308) -> ()  [unwired: 2 in, 2 out]
      n105 = property on="Progress bar" class="Slide (strict)"("DisabledEnum"=w308) -> ()  [unwired: 2 in, 2 out]
      n106 = property on="ScanRunning?" class="Bool (strict)"("DisabledEnum"=w308) -> ()  [unwired: 2 in, 2 out]
      "ScanRunning?" <- FALSE ("ScanRunning?")
    }
  }
  n107 = Generate Occurrence "Stop Occurrence"() -> (w78:refnum<k4>)
  n108 = Create User Event(user event datatype=w154, error in=w100) -> (user event=w35:refnum<user-event>, error out=w147:errorcluster)
  n109 = Create User Event(user event datatype=w146, error in=w147) -> (user event=w1:refnum<user-event>, error out=w139:errorcluster)
  n110 = Create User Event(user event datatype=w44, error in=w139) -> (user event=w41:refnum<user-event>, error out=w134:errorcluster)
  n111 = Obtain Notifier(notification data type=w133, error in (no error)=w134) -> (notifier out=w132:refnum<notifier>, error out=w38:errorcluster)  [unwired: 2 in, 1 out]
  n112 = Create User Event(user event datatype=w40, error in=w38) -> (user event=w39:refnum<user-event>, error out=w37:errorcluster)
  n113 = Create User Event(user event datatype=w43, error in=w37) -> (user event=w42:refnum<user-event>, error out=w114:errorcluster)
  n114 = Create User Event(user event datatype=w113, error in=w114) -> (user event=w112:refnum<user-event>, error out=w74:errorcluster)
  n115 = Create User Event(user event datatype=w72, error in=w74) -> (user event=w71:refnum<user-event>, error out=w73:errorcluster)
  n116 = Create User Event(user event datatype=w75, error in=w73) -> (user event=w3:refnum<user-event>, error out=w49:errorcluster)
  n117 = Create User Event(user event datatype=w47, error in=w49) -> (user event=w46:refnum<user-event>, error out=w48:errorcluster)
  n118 = call "IMAQController.get i attribute.vi"("i ref in"=w97, "error in (no error)"=w48) -> ("i ref out"=w79:refnum<vi>, "i attribute"=w106:T17, "error out"=w107:errorcluster)  [unwired: 15 in]
  n119 = Unbundle By Name(w106) -> ("actCamera"=w102:string)
  n120 = Concatenate Strings(w102, "_Image" ("string")) -> (w103:string)
  n121 = for {
    N: w101 -> [_]
    shift-right: [w327] -> w108
    shift-left: w107 -> [w316]
    tunnel: [w326] -> w105 mode=indexing
    tunnel: w103 -> [w317]
    tunnel: i8[] [] -> [w314]
    tunnel: [w313] -> w109 mode=indexing
    i -> [w319]
    w325 = T22 4 items=["ONCE_ONLY"=1, "TIMED"=2, "MONITORED"=4] ("serviceType")
    n122 = Increment(x=w319) -> (x+1=w321:i32)
    n123 = Number To Decimal String(number=w321) -> (decimal integer string=w320:string)  [unwired: 1 in]
    n124 = Obtain Queue(element data type=w314, error in (no error)=w316) -> (queue out=w313:refnum<queue>, error out=w315:errorcluster)  [unwired: 3 in, 1 out]
    n125 = Concatenate Strings(w317, "_", w320) -> (w318:string)
    n126 = call-poly "LVDimInterface.dic_info_service.vi"("serviceName"=w318, "queueRef"=w313, "timeout [s]"=0, "serviceType"=w325, "error in (no error)"=w315, "stamped"=FALSE) -> ("callBackID"=w326:i32, "error out"=w327:errorcluster)  [unwired: 12 in]
  }
  "DIM Array" <- w109
  n127 = Concatenate Strings(w32, "_RAWImage2" ("string")) -> (w91:string)
  n128 = call <vilib>:"Simple Error Handler.vi"("type of dialog (OK msg:1)"=w136, "error in (no error)"=w108) -> ("error out"=w96:errorcluster)  [unwired: 3 in, 4 out]
  n129 = call "IMAQ Create"("Image Name"=w91) -> ("New Image"=w94:T3)  [unwired: 4 in, 1 out]
  n130 = register-events(error in=w96, w35, w41) -> (reference out=w145:refnum<event-registration>, error out=w144:errorcluster)  [unwired: 1 in]
  n131 = register-events(error in=w96, w35, w39, w3) -> (reference out=w140:refnum<event-registration>, error out=w141:errorcluster)  [unwired: 1 in]
  n132 = Concatenate Strings(w32, "_LQueue" ("string")) -> (w34:string)
  n133 = register-events(w1, w35) -> (reference out=w36:refnum<event-registration>)  [unwired: 2 in, 1 out]
  n134 = register-events(error in=w96, w35) -> (reference out=w152:refnum<event-registration>, error out=w153:errorcluster)  [unwired: 1 in]
  n135 = register-events(error in=w96, w35, w42, w112, w71, w3) -> (reference out=w150:refnum<event-registration>, error out=w151:errorcluster)  [unwired: 1 in]
  n136 = Obtain Queue(max queue size (-1, unlimited)=w31, name (unnamed)=w34, element data type=w28) -> (queue out=w30:refnum<queue>)  [unwired: 2 in, 2 out]
  n137 = while "DIM Client Loop" {
    tunnel: [w331] -> w179
    tunnel: w172 -> [w353]
    tunnel: [w354] -> w156
    shift-right: [w351] -> _
    shift-left: w178 -> [w352]
    shift-right: [w350] -> _
    shift-left: w177 -> [w349]
    shift-right: [w347] -> _
    shift-left: 0 ("DIM service length / byte") -> [w348]
    shift-right: [w345] -> _
    shift-left: w175 -> [w346]
    shift-right: [w343] -> _
    shift-left: w175 -> [w344]
    shift-right: [w330] -> w157
    shift-left: w96 -> [w355]
    tunnel: w78 -> [w338]
    tunnel: w41 -> [w337]
    tunnel: w132 -> [w336]
    tunnel: w69 -> [w334]
    tunnel: w79 -> [w333]
    tunnel: w1 -> [w329]
    tunnel: w64 -> [w328]
    i -> [w342]
    stop <- w339 continue-if-true
    n138 = local read "DIM Array"() -> (w331:refnum<queue>[])
    n139 = case shown="True" "Camera\nConnected?" {
      tunnel: w355 -> [w357 w379]
      tunnel: [w356 w378] -> w354
      tunnel: w353 -> [w356 w377]
      tunnel: w352 -> [_ w376]
      tunnel: [_ w375] -> w351
      tunnel: [_ w374] -> w350
      tunnel: w349 -> [_ w373]
      tunnel: w348 -> [_ w372]
      tunnel: [_ w371] -> w347
      tunnel: w346 -> [_ w370]
      tunnel: [_ w369] -> w345
      tunnel: w344 -> [_ w368]
      tunnel: [_ w367] -> w343
      tunnel: w337 -> [_ w366]
      tunnel: [w357 w365] -> w330
      tunnel: w331 -> [_ w364]
      tunnel: w336 -> [_ w363]
      tunnel: "Network Transport" -> [_ w362]
      tunnel: w334 -> [_ w361]
      tunnel: w333 -> [_ w360]
      tunnel: w329 -> [_ w359]
      tunnel: w328 -> [_ w358]
      frame False {
      }
      frame True {
        n140 = case shown="\"Radio Selection 1\", Default" w362 {
          tunnel: w379 -> [w407 w720]
          tunnel: [w406 w717] -> w378
          tunnel: w377 -> [w405 w721]
          tunnel: w376 -> [w404 _]
          tunnel: [w403 _] -> w375
          tunnel: [w400 _] -> w374
          tunnel: w373 -> [w399 _]
          tunnel: w364 -> [w398 _]
          tunnel: w372 -> [w397 _]
          tunnel: [w395 _] -> w371
          tunnel: w370 -> [w394 _]
          tunnel: [w393 _] -> w369
          tunnel: w368 -> [w392 _]
          tunnel: [w390 _] -> w367
          tunnel: [w388 w719] -> w365
          tunnel: w366 -> [w380 _]
          tunnel: w364 -> [w387 _]
          tunnel: w363 -> [w385 _]
          tunnel: w361 -> [w384 w716]
          tunnel: w360 -> [w383 _]
          tunnel: w359 -> [w382 _]
          tunnel: w358 -> [w381 _]
          frame "Radio Selection 1", Default {
            n141 = case shown="True" w404 {
              tunnel: w398 -> [w494 w643]
              tunnel: w407 -> [w502 w650]
              tunnel: [w501 w649] -> w389
              tunnel: w392 -> [w500 w648]
              selector: w404 -> [w499 w640]
              tunnel: [w498 w639] -> w403
              tunnel: [w497 w638] -> w402
              tunnel: [w496 w637] -> w401
              tunnel: w399 -> [_ w629]
              tunnel: w397 -> [w492 w636]
              tunnel: [w491 w635] -> w396
              tunnel: [w489 w634] -> w393
              tunnel: w394 -> [w490 w633]
              tunnel: [w488 w632] -> w391
              tunnel: w387 -> [w487 _]
              tunnel: [w485 w629] -> w386
              tunnel: w385 -> [w484 w630]
              frame True {
                w495 = 1  # aktueller Service
                n142 = Array Size(array=w494) -> (size(s)=w493:i32)
                n143 = while {
                  tunnel: w494 -> [w518]
                  tunnel: w499 -> [w522]
                  tunnel: [w521] -> w498
                  tunnel: [w520] -> w497
                  tunnel: [w519] -> w496
                  shift-right: [w528] -> w488
                  shift-left: w500 -> [w527]
                  shift-right: [w529] -> w501
                  shift-left: w502 -> [w530]
                  shift-right: [w515] -> _
                  shift-left: w495 -> [w516]
                  tunnel: w493 -> [w514]
                  shift-right: [w511] -> w491
                  shift-left: w492 -> [w512]
                  tunnel: w490 -> [w510]
                  tunnel: [w509] -> w489
                  tunnel: w487 -> [w508]
                  tunnel: [w505] -> w486
                  tunnel: w484 -> [w503]
                  stop <- w506 stop-if-true
                  # "andere DIM service\n(werden nur nach erstem abgefragt)"
                  n144 = Index Array(array=w518, index=w516) -> (element=w517:refnum<queue>)
                  n145 = Dequeue Element(queue=w517, timeout in ms (-1)=2000, error in (no error)=w530) -> (element=w524:i8[], timed out?=w525:bool, error out=w504:errorcluster)  [unwired: 1 out]
                  n146 = case shown="No Error" w504 {
                    selector: w504 -> [w531 w611]
                    tunnel: [w547 w610] -> w529
                    tunnel: w525 -> [w546 _]
                    tunnel: w524 -> [w545 _]
                    tunnel: [w544 _] -> w523
                    tunnel: w522 -> [w543 w618]
                    tunnel: [w542 w618] -> w521
                    tunnel: [w541 -1 ("callBackID")] -> w520
                    tunnel: [w540 FALSE ("no link")] -> w519
                    tunnel: w516 -> [w539 w615]
                    tunnel: [w538 w615] -> w515
                    tunnel: w512 -> [w537 w616]
                    tunnel: [w536 w616] -> w511
                    tunnel: w510 -> [w535 w617]
                    tunnel: [w534 w617] -> w509
                    tunnel: w508 -> [w533 _]
                    tunnel: [w532 TRUE] -> w505
                    tunnel: w503 -> [_ w609]
                    frame No Error {
                      n147 = case "timed out?" shown="False" w546 {
                        tunnel: w545 -> [w563 _]
                        tunnel: w531 -> [w562 w608]
                        tunnel: [w561 w608] -> w547
                        tunnel: [w560 _] -> w544
                        tunnel: w543 -> [w559 w607]
                        tunnel: [w558 w607] -> w542
                        tunnel: [w557 _] -> w541
                        tunnel: [w556 _] -> w540
                        tunnel: w539 -> [w555 w606]
                        tunnel: [w554 w606] -> w538
                        tunnel: w537 -> [w553 w605]
                        tunnel: [w552 w605] -> w536
                        tunnel: w535 -> [w551 w604]
                        tunnel: [w550 w604] -> w534
                        tunnel: w533 -> [w549 _]
                        tunnel: [w548 TRUE] -> w532
                        frame False {
                          n148 = call "LVDimInterface.dim_unfold_data.vi"("rawData"=w563, "error in (no error)"=w562) -> ("data"=w564:i8[], "callBackID"=w557:i32, "no link"=w556:bool, "error out"=w561:errorcluster)  [unwired: 14 in]
                          n149 = case "no link?" shown="False" w556 {
                            tunnel: w564 -> [w575 _]
                            tunnel: [w582 _] -> w560
                            tunnel: w559 -> [_ w602]
                            tunnel: [w581 w602] -> w558
                            tunnel: w555 -> [w580 w601]
                            tunnel: [w579 w601] -> w554
                            tunnel: w553 -> [w578 w600]
                            tunnel: [w577 w600] -> w552
                            tunnel: w551 -> [w570 w599]
                            tunnel: [w569 w599] -> w550
                            tunnel: w549 -> [w566 _]
                            tunnel: [w565 TRUE] -> w548
                            frame False {
                              n150 = Type Cast(type=i16[] [], x=w575) -> (*(type *) &x=w572:i16[])
                              n151 = Split 1D Array(array=w572, index=3) -> (first subarray=w571:i16[], second subarray=w573:i16[])
                              n152 = Equal?(x=w570, y=w571) -> (x = y?=w567:bool[])
                              n153 = And Array Elements(Boolean array=w567) -> (logical AND=w568:bool)
                              n154 = case shown="False" w568 {
                                tunnel: w573 -> [_ w591]
                                tunnel: [_ w591] -> w582
                                tunnel: [FALSE FALSE] -> w581
                                tunnel: w580 -> [w587 w596]
                                tunnel: [w587 w595] -> w579
                                tunnel: w578 -> [w586 w594]
                                tunnel: [w586 w592] -> w577
                                tunnel: w570 -> [w585 w590]
                                tunnel: [w585 w590] -> w569
                                tunnel: w566 -> [w584 _]
                                tunnel: [TRUE _] -> w565
                                frame False {
                                n155 = for {
                                tunnel: w584 -> [w589] mode=indexing
                                n156 = Flush Queue(queue=w589) -> ()  [unwired: 1 in, 3 out]
                                }
                                }
                                frame True {
                                n157 = Array Size(array=w591) -> (size(s)=w593:i32)
                                n158 = Add(x=w593, y=w594) -> (x+y=w592:i32)
                                n159 = Increment(x=w596) -> (x+1=w595:i32)
                                }
                              }
                            }
                            frame True {
                            }
                          }
                        }
                        frame True {
                        }
                      }
                    }
                    frame Error {
                      n160 = Wait on Notification(notifier=w609, timeout in ms (-1)=500) -> (notification=w612:i32, timed out?=w613:bool)  [unwired: 2 in, 2 out]
                      n161 = case shown="False" w613 {
                        tunnel: w611 -> [w623 w628]
                        tunnel: [w622 w628] -> w610
                        tunnel: w612 -> [w624 _]
                        frame False {
                          n162 = case shown="0" w624 {
                            tunnel: w623 -> [w626 w627]
                            tunnel: [w625 w627] -> w622
                            frame 0 {
                              n163 = call <vilib>:"Clear Errors.vi"("error in (no error)"=w626) -> ("error out"=w625:errorcluster)  [unwired: 5 in, 1 out]
                            }
                            frame Default {
                            }
                          }
                        }
                        frame True {
                        }
                      }
                    }
                  }
                  n164 = Increment(x=w515) -> (x+1=w513:i32)
                  n165 = Greater?(x=w513, y=w514) -> (0:w507:bool)
                  n166 = Insert Into Array(array=w527, new element=w523) -> (w528:i16[])  [unwired: 1 in]
                  n167 = Or(x=w505, y=w507) -> (x .or. y?=w506:bool)
                  "aktueller\nService" <- w516
                }
                n168 = Not(x=w486) -> (.not. x?=w485:bool)
              }
              frame False {
                # "not working\nfor only 1 DIM\nservice !!!!!!!"
                # "erster DIM service\n(auf diesen wird gewartet, bis er aktualisiert wurde)"
                n169 = Index Array(array=w643, index=0) -> (element=w641:refnum<queue>)
                n170 = Dequeue Element(queue=w641, timeout in ms (-1)=2000, error in (no error)=w650) -> (element=w645:i8[], timed out?=w646:bool, error out=w631:errorcluster)  [unwired: 1 out]
                n171 = case shown="No Error" w631 {
                  selector: w631 -> [w651 w702]
                  tunnel: [w663 w701] -> w649
                  tunnel: w646 -> [w662 _]
                  tunnel: w645 -> [w661 _]
                  tunnel: [w660 _] -> w644
                  tunnel: w640 -> [w659 w708]
                  tunnel: [w658 w708] -> w639
                  tunnel: [w657 _] -> w638
                  tunnel: [w656 _] -> w637
                  tunnel: w636 -> [w655 w707]
                  tunnel: [w654 w707] -> w635
                  tunnel: [w653 w706] -> w634
                  tunnel: w633 -> [w652 w706]
                  tunnel: w630 -> [_ w705]
                  frame No Error {
                    n172 = case "timed out?" shown="False" w662 {
                      tunnel: w661 -> [w675 _]
                      tunnel: w651 -> [w674 w699]
                      tunnel: [w673 w699] -> w663
                      tunnel: [w672 _] -> w660
                      tunnel: w659 -> [w671 w698]
                      tunnel: [w670 w698] -> w658
                      tunnel: [w668 _] -> w657
                      tunnel: [w669 _] -> w656
                      tunnel: w655 -> [w667 w697]
                      tunnel: [w666 w697] -> w654
                      tunnel: [w665 w696] -> w653
                      tunnel: w652 -> [w664 w696]
                      frame False {
                        n173 = call "LVDimInterface.dim_unfold_data.vi"("rawData"=w675, "error in (no error)"=w674) -> ("data"=w676:i8[], "callBackID"=w668:i32, "no link"=w669:bool, "error out"=w673:errorcluster)  [unwired: 14 in]
                        n174 = case "no link?" shown="False" w669 {
                          tunnel: w676 -> [w692 _]
                          tunnel: [w689 _] -> w672
                          tunnel: w671 -> [_ w695]
                          tunnel: [TRUE w695] -> w670
                          tunnel: w667 -> [w685 w694]
                          tunnel: [w683 w694] -> w666
                          tunnel: [w679 w693] -> w665
                          tunnel: w664 -> [_ w693]
                          frame False {
                            n175 = Type Cast(type=i16[] [], x=w692) -> (*(type *) &x=w691:i16[])
                            n176 = Array Size(array=w691) -> (size(s)=w684:i32)
                            n177 = Split 1D Array(array=w691, index=5) -> (first subarray=w680:i16[], second subarray=w689:i16[])
                            n178 = Add(x=w684, y=w685) -> (x+y=w683:i32)
                            n179 = Split 1D Array(array=w680, index=3) -> (first subarray=w679:i16[], second subarray=w681:i16[])
                            n180 = Index Array(array=w681, index #1=0 ("index")) -> (element #1=→"Image height":i16, element #2=→"Image length":i16)  [unwired: 1 in]
                          }
                          frame True {
                          }
                        }
                      }
                      frame True {
                      }
                    }
                  }
                  frame Error {
                    n181 = Wait on Notification(notifier=w705, timeout in ms (-1)=500) -> (notification=w700:i32, timed out?=w703:bool)  [unwired: 2 in, 2 out]
                    n182 = case shown="False" w703 {
                      tunnel: w702 -> [w710 w715]
                      tunnel: [w709 w715] -> w701
                      tunnel: w700 -> [w711 _]
                      frame False {
                        n183 = case shown="0" w711 {
                          tunnel: w710 -> [w713 w714]
                          tunnel: [w712 w714] -> w709
                          frame 0 {
                            n184 = call <vilib>:"Clear Errors.vi"("error in (no error)"=w713) -> ("error out"=w712:errorcluster)  [unwired: 5 in, 1 out]
                          }
                          frame Default {
                          }
                        }
                      }
                      frame True {
                      }
                    }
                  }
                }
                n185 = Insert Into Array(array=w648, new element=w644) -> (w632:i16[])  [unwired: 1 in]
              }
            }
            "callBackID" <- w402
            "no link" <- w401
            "TimeStamp Data" <- w393
            n186 = case shown="True" w386 {
              selector: w386 -> [w415 _]
              tunnel: [w416 w422] -> w406
              tunnel: w405 -> [w416 w431]
              tunnel: [w415 FALSE] -> w400
              tunnel: w396 -> [w414 w429]
              tunnel: [w414 _] -> w395
              tunnel: w391 -> [w413 w428]
              tunnel: [w413 w427] -> w390
              tunnel: w389 -> [w409 w426]
              tunnel: [w408 w425] -> w388
              tunnel: w380 -> [_ w424]
              tunnel: w384 -> [_ w423]
              tunnel: w383 -> [_ w421]
              tunnel: w382 -> [_ w420]
              tunnel: w381 -> [_ w419]
              frame False {
                # "The reason for this is that if you change the\ncamera the GUI will delete the Queue and\nmaybe he still tries to read out the old one\nleading to this error"
                n187 = Unbundle By Name(w409) -> ("code"=w412:i32)
                n188 = Equal?(x=w412, y=1122) -> (x = y?=w410:bool)
                n189 = case shown="True" w410 {
                  tunnel: [w417 errorcluster {"status"=FALSE, "code"=0, "source"=""} ("error out")] -> w408
                  tunnel: w409 -> [w417 _]
                  frame False {
                  }
                  frame True {
                  }
                }
              }
              frame True {
                n190 = stacked-sequence {
                  seq-local: [_ w462 _] -> [_ _ w479]
                  seq-local: [_ w451 _] -> [_ _ w476]
                  seq-local: [w441 _ _] -> [_ w450 _]
                  seq-local: [w437 _ _] -> [_ w447 _]
                  seq-local: [w438 _ _] -> [_ w446 _]
                  tunnel: [_ w464 _] -> w422
                  tunnel: w431 -> [_ w461 _]
                  tunnel: w429 -> [_ _ w483]
                  tunnel: w428 -> [_ w465 _]
                  tunnel: [_ _ i16[] [] ("Array")] -> w427
                  tunnel: w426 -> [_ w467 _]
                  tunnel: [_ _ w473] -> w425
                  tunnel: w424 -> [_ w444 _]
                  tunnel: w423 -> [_ w460 _]
                  tunnel: w421 -> [_ w466 _]
                  tunnel: w420 -> [_ _ w478]
                  tunnel: w419 -> [_ w448 _]
                  frame #0 {
                    w433 = T23 {"Last scan started"="", "ScanValuesArray"=[], "ActDimensions"=0, "ScanNamesArray"=[]}  # Scan Variables
                    n191 = local read "ScanRunning?"() -> (w438:bool)
                    n192 = local read "Last scan started"() -> (w436:string)
                    n193 = local read "ScanValuesArray"() -> (w435:dbl[])
                    n194 = local read "ActDimensions"() -> (w434:i16)
                    n195 = call <vilib>:"Check if File or Folder Exists.vi"("path"="Save Path") -> ("file or folder exists?"=w439:bool)  [unwired: 8 in, 2 out]
                    n196 = Bundle(cluster=w433, "Last scan started"=w436, "ScanValuesArray"=w435, "ActDimensions"=w434, "ScanNamesArray"="ScanNamesArray") -> (w437:T23)
                    n197 = case shown="False" w439 {
                      tunnel: "Save Path" -> [_ w443]
                      tunnel: [w442 w443] -> w441
                      frame False {
                        n198 = call <vilib>:"Dflt Data Dir.vi"() -> ("App:Default Data Directory"=w442:path)
                      }
                      frame True {
                      }
                    }
                  }
                  frame #1 {
                    n199 = local read "Image length"() -> (w453:i32)
                    n200 = local read "Image height"() -> (w454:i32)
                    n201 = local read "Overlay Lines"() -> (w459:T5)
                    n202 = control-ref of="ActImage"() -> (w457:refnum<vi>)
                    n203 = local read "Show Grid ?"() -> (w456:bool)
                    n204 = call "IMAQController.ImageProcessing.vi"("i ref in"=w466, "Image ref in"=w457, "ActImage"=w461, "RawImage"=w460, "DIM data"=w465, "ImageHeight"=w454, "ImageWidth"=w453, "error in (no error)"=w467, "Ana Step 1 Event"=w444, "Save?"="auto save", "Grid Color"="Grid Color Box", "Overlay Lines In"=w459, "Save path in"=w450, "Overlay already configured?"="Overlay configured?", "Save Overlay?"=FALSE, "ShowGrid?"=w456, "Scan Variables"=w447, "SaveImage"=w448, "Scan Running?"=w446, "Averaging"="Averaging") -> ("Overlay Lines Out"=→"Overlay Lines":T5, "ActImage Out"=w464:T3, "Error?"=w451:bool, "error out"=w462:errorcluster)  [unwired: 2 in, 2 out]
                  }
                  frame #2 {
                    w471 = T12 {"Message"="", "Error?"=TRUE, "current time"=timestamp(0 s since 1904-01-01)}  # Logger String
                    n205 = local read "Image Arrived"() -> (w475:i32)
                    n206 = Not(x=w476) -> (.not. x?=w477:bool)
                    n207 = local write "Overlay configured?"(w477) -> ()
                    n208 = Multiply(x=2, y=w483) -> (x*y=→"DIM service length / byte":i32)
                    n209 = Increment(x=w475) -> (x+1=→"Image Arrived":i32)
                    n210 = Get Date/Time In Seconds() -> (seconds since 1Jan1904=w468:timestamp)
                    n211 = Bundle By Name(cluster=w471, "Message"="New image arrived", "Error?"=FALSE, "current time"=w468) -> (w472:T12)
                    n212 = Generate User Event(user event=w478, event data cluster=w472, error in=w479) -> (error out=w473:errorcluster)  [unwired: 1 in, 1 out]
                  }
                }
              }
            }
          }
          frame "Radio Selection 2" {
            n213 = event shown="[1] \"ActualImageLink(Compression Mode)\": Value Change" {
              selector: _ -> [_ _ _]
              dyn-events: _ -> [_ _ _]
              timeout: 100 -> [_ _ _]
              tunnel: w721 -> [w722 w729 w732]
              tunnel: w720 -> [w723 w728 w735]
              tunnel: [w723 w725 w733] -> w719
              tunnel: [w722 w727 w732] -> w717
              tunnel: w716 -> [_ w724 _]
              event Timeout {
                n214 = event-data() -> ()  [unwired: 1 in, 2 out]
              }
              event Value Change {
                n215 = event-data() -> ("NewVal"=w731:T6)  [unwired: 1 in, 4 out]
                n216 = Unbundle By Name(w731) -> ("data"=w730:string)
                n217 = Unflatten From String(type=w729, binary string=w730, error in (no error)=w728) -> (value=w727:T3, error out=w726:errorcluster)  [unwired: 2 in, 1 out]
                n218 = call "IMAQ Copy"("error in (no error)"=w726, "Image Dst"=w724, "Image Src"=w727) -> ("error out"=w725:errorcluster)  [unwired: 3 in, 1 out]
                n219 = local write "ActImage"(w727) -> ()
              }
              event "Error UL": Mouse Down {
                n220 = event-data() -> ()  [unwired: 1 in, 7 out]
                n221 = call <vilib>:"Clear Errors.vi"("error in (no error)"=w735) -> ("error out"=w734:errorcluster)  [unwired: 5 in, 1 out]
                n222 = invoke on="Error UL" class="Bool (strict)" method="Reinit To Default"(error in=w734) -> (error out=w733:errorcluster)  [unwired: 2 in, 2 out]
              }
            }
          }
        }
      }
    }
    n223 = local write "DIM client error out"(w330) -> ()
    n224 = case shown="Error" w330 {
      frame No Error {
      }
      frame Error {
        n225 = Wait (ms)(milliseconds to wait=u32 2000 ("millisecond multiple")) -> ()  [unwired: 1 out]
      }
    }
    n226 = Wait on Occurrence(1:FALSE ("ignore previous (T)"), 2:w338, 3:10 ("ms timeout (-1)")) -> (0:w339:bool)
    "DIM Client Loop" <- w342
  }
  n227 = while "CameraTimeStamp Loop" {
    tunnel: w78 -> [w742]
    stop <- w743 continue-if-true
    n228 = property on="Camera Choice" class="MCListbox (strict)"() -> ("ItemNames"=w740:string[][])  [unwired: 2 in, 2 out]
    n229 = local read "Camera Choice"() -> (w741:i32[])
    n230 = Get Date/Time In Seconds() -> (seconds since 1Jan1904=w738:timestamp)
    n231 = To Double Precision Float(number=w738) -> (double precision float=w737:dbl)
    n232 = for {
      tunnel: w741 -> [w749] mode=indexing
      tunnel: w737 -> [w754]
      shift-right: [w750] -> w739
      shift-left: w740 -> [w753]
      i -> [w746]
      w760 = ":" ("string")
      n233 = local read "CameraTimeStamps"() -> (w748:dbl[])
      n234 = Index Array(array=w748, index=w746) -> (element=w747:dbl)
      n235 = Subtract(x=w754, y=w747) -> (x-y=w767:dbl)
      n236 = Quotient & Remainder(x=w767, y=3600.0) -> (x-y*floor(x/y)=w757:dbl, floor(x/y)=w759:dbl)
      n237 = Quotient & Remainder(x=w757, y=60.0) -> (x-y*floor(x/y)=w761:dbl, floor(x/y)=w766:dbl)
      n238 = Number To Decimal String(number=w759) -> (decimal integer string=w758:string)  [unwired: 1 in]
      n239 = Number To Decimal String(number=w766, width (-)=i16 2) -> (decimal integer string=w765:string)
      n240 = Number To Decimal String(number=w761, width (-)=i16 2) -> (decimal integer string=w762:string)
      n241 = Concatenate Strings(w758, w760, w765, w760, w762) -> (w751:string)
      n242 = Replace Array Subset(array=w753, new element=w751, index (row)=w749, index (col)=3 ("disabled index (col)")) -> (w750:string[][])
    }
    n243 = property on="Camera Choice" class="MCListbox (strict)"("ItemNames"=w739) -> ()  [unwired: 2 in, 2 out]
    n244 = Wait on Occurrence(1:FALSE ("ignore previous (T)"), 2:w742, 3:10000 ("ms timeout (-1)")) -> (0:w743:bool)
  }
  n245 = stacked-sequence "ScanValue-DIM Loop + Add Scan DimServices" {
    seq-local: [_ _ w807 _ _ _] -> [_ _ _ _ _ w941]
    seq-local: [_ _ w814 _ _ _] -> [_ _ _ _ w867 w947]
    seq-local: [_ _ _ w848 _ _] -> [_ _ _ _ w866 w946]
    seq-local: [_ _ _ w844 _ _] -> [_ _ _ _ _ w942]
    seq-local: [w769 _ _ _ _ _] -> [_ _ w805 _ _ _]
    seq-local: [_ w786 _ _ _ _] -> [_ _ _ _ w865 w945]
    seq-local: [_ w785 _ _ _ _] -> [_ _ _ _ _ w943]
    seq-local: [_ _ _ w847 _ _] -> [_ _ _ _ w864 _]
    seq-local: [_ _ w806 _ _ _] -> [_ _ _ _ w862 _]
    tunnel: w32 -> [_ w779 w810 w841 _ _]
    tunnel: w79 -> [w774 w799 w816 w861 _ _]
    tunnel: w78 -> [_ _ _ _ w868 _]
    tunnel: w71 -> [_ _ _ _ w863 _]
    frame #0 {
      n246 = call "IMAQController.get i attribute.vi"("i ref in"=w774) -> ("i attribute"=w775:T17)  [unwired: 16 in, 2 out]
      n247 = Unbundle By Name(w775) -> ("actScanner"=w768:string)
      n248 = Concatenate Strings(w768, "_MaxDimensions" ("string")) -> (w771:string)
      n249 = call "LVDimInterface.dic_info_service_once.vi"("serviceName"=w771) -> ("data"=w772:i8[])  [unwired: 15 in, 3 out]
      n250 = Type Cast(type=0, x=w772) -> (*(type *) &x=w769:i32)
    }
    frame #1 {
      w778 = "_1DMin"
      w783 = T22 4 items=["ONCE_ONLY"=1, "TIMED"=2, "MONITORED"=4] ("serviceType")
      w793 = T22 4 items=["ONCE_ONLY"=1, "TIMED"=2, "MONITORED"=4] ("serviceType")
      w798 = "_nofSteps" ("string")
      w797 = "_curStep" ("string")
      w801 = T22 4 items=["ONCE_ONLY"=1, "TIMED"=2, "MONITORED"=4] ("serviceType")
      n251 = call "IMAQController.get i attribute.vi"("i ref in"=w799) -> ("i attribute"=w800:T17)  [unwired: 16 in, 2 out]
      n252 = Unbundle By Name(w800) -> ("actScanner"=w780:string)
      n253 = Concatenate Strings(w779, w798) -> (w796:string)
      n254 = Concatenate Strings(w780, w798) -> (w795:string)
      n255 = Concatenate Strings(w779, w797) -> (w791:string)
      n256 = Concatenate Strings(w780, w797) -> (w792:string)
      n257 = Concatenate Strings(w780, w778) -> (w782:string)
      n258 = Concatenate Strings(w779, w778) -> (w781:string)
      n259 = Obtain Notifier(name (unnamed)=w796, notification data type=i8[] []) -> (notifier out=w788:refnum<notifier>)  [unwired: 2 in, 2 out]
      n260 = Obtain Notifier(name (unnamed)=w791, notification data type=i8[] []) -> (notifier out=w787:refnum<notifier>)  [unwired: 2 in, 2 out]
      n261 = Obtain Notifier(name (unnamed)=w781, notification data type=i8[] []) -> (notifier out=w777:refnum<notifier>)  [unwired: 2 in, 2 out]
      n262 = call "LVDimInterface.dic_info_service_notifier.vi"("serviceName"=w795, "notifierRef"=w788, "serviceType"=w801) -> ("callBackID"=w790:i32)  [unwired: 15 in, 1 out]
      n263 = call "LVDimInterface.dic_info_service_notifier.vi"("serviceName"=w792, "notifierRef"=w787, "serviceType"=w793) -> ("callBackID"=w789:i32)  [unwired: 15 in, 1 out]
      n264 = call "LVDimInterface.dic_info_service_notifier.vi"("serviceName"=w782, "notifierRef"=w777, "serviceType"=w783) -> ("callBackID"=w776:i32)  [unwired: 15 in, 1 out]
      n265 = Build Array(w790, w789, w776) -> (w785:i32[])
      n266 = Build Array(w788, w787, w777) -> (w786:refnum<notifier>[])
    }
    frame #2 {
      n267 = call "IMAQController.get i attribute.vi"("i ref in"=w816) -> ("i attribute"=w815:T17)  [unwired: 16 in, 2 out]
      n268 = Unbundle By Name(w815) -> ("actScanner"=w811:string)
      n269 = for {
        N: w805 -> [_]
        tunnel: w810 -> [w840]
        tunnel: w811 -> [w833]
        tunnel: [w830] -> w809 mode=indexing
        tunnel: [w829] -> w814 mode=indexing
        i -> [w838]
        w835 = T22 4 items=["ONCE_ONLY"=1, "TIMED"=2, "MONITORED"=4] ("serviceType")
        n270 = Number To Decimal String(number=w838) -> (decimal integer string=w832:string)  [unwired: 1 in]
        n271 = Concatenate Strings(w833, "_NomValue_", w832) -> (w831:string)
        n272 = Concatenate Strings(w840, "_SValue_" ("string"), w832) -> (w837:string)
        n273 = Obtain Notifier(name (unnamed)=w837, notification data type=i8[] []) -> (notifier out=w829:refnum<notifier>)  [unwired: 2 in, 2 out]
        n274 = call "LVDimInterface.dic_info_service_notifier.vi"("serviceName"=w831, "notifierRef"=w829, "serviceType"=w835) -> ("callBackID"=w830:i32)  [unwired: 15 in, 1 out]
      }
      n275 = for {
        N: w805 -> [_]
        tunnel: w810 -> [w828]
        tunnel: w811 -> [w821]
        tunnel: [w818] -> w808 mode=indexing
        tunnel: [w817] -> w806 mode=indexing
        i -> [w826]
        w823 = T22 4 items=["ONCE_ONLY"=1, "TIMED"=2, "MONITORED"=4] ("serviceType")
        n276 = Number To Decimal String(number=w826) -> (decimal integer string=w820:string)  [unwired: 1 in]
        n277 = Concatenate Strings(w821, "_ScannedNames_", w820) -> (w819:string)
        n278 = Concatenate Strings(w828, "_SNames_" ("string"), w820) -> (w825:string)
        n279 = Obtain Notifier(name (unnamed)=w825, notification data type=i8[] []) -> (notifier out=w817:refnum<notifier>)  [unwired: 2 in, 2 out]
        n280 = call "LVDimInterface.dic_info_service_notifier.vi"("serviceName"=w819, "notifierRef"=w817, "serviceType"=w823) -> ("callBackID"=w818:i32)  [unwired: 15 in, 1 out]
      }
      n281 = Initialize Array(0.0, w805) -> (→"ScanValuesArray":dbl[])
      n282 = Initialize Array("", w805) -> (w804:string[])
      n283 = Build Array (concatenate)(w809, w808) -> (w807:i32[])
      n284 = local write "ScanNamesArray"(w804) -> ()
    }
    frame #3 {
      w842 = "_seqDone" ("string")
      w851 = T22 4 items=["ONCE_ONLY"=1, "TIMED"=2, "MONITORED"=4] ("serviceType")
      w856 = "_Dimensions" ("string")
      w858 = T22 4 items=["ONCE_ONLY"=1, "TIMED"=2, "MONITORED"=4] ("serviceType")
      n285 = call "IMAQController.get i attribute.vi"("i ref in"=w861) -> ("i attribute"=w860:T17)  [unwired: 16 in, 2 out]
      n286 = Unbundle By Name(w860) -> ("actScanner"=w853:string, "actSequencer"=w843:string)
      n287 = Concatenate Strings(w841, w856) -> (w855:string)
      n288 = Concatenate Strings(w841, w842) -> (w849:string)
      n289 = Concatenate Strings(w853, w856) -> (w857:string)
      n290 = Concatenate Strings(w843, w842) -> (w850:string)
      n291 = Obtain Notifier(name (unnamed)=w855, notification data type=i8[] []) -> (notifier out=w848:refnum<notifier>)  [unwired: 2 in, 2 out]
      n292 = Obtain Notifier(name (unnamed)=w849, notification data type=i8[] []) -> (notifier out=w847:refnum<notifier>)  [unwired: 2 in, 2 out]
      n293 = call "LVDimInterface.dic_info_service_notifier.vi"("serviceName"=w857, "notifierRef"=w848, "serviceType"=w858) -> ("callBackID"=w846:i32)  [unwired: 15 in, 1 out]
      n294 = call "LVDimInterface.dic_info_service_notifier.vi"("serviceName"=w850, "notifierRef"=w847, "serviceType"=w851) -> ("callBackID"=w845:i32)  [unwired: 15 in, 1 out]
      n295 = Build Array(w846, w845) -> (w844:i32[])
      "ActDimensions" <- i16 0 ("ActDimensions")
    }
    frame #4 {
      n296 = while {
        tunnel: w868 -> [w903]
        tunnel: w867 -> [w902]
        tunnel: w866 -> [w898]
        tunnel: w865 -> [w893]
        tunnel: w864 -> [w883]
        tunnel: w863 -> [w882]
        tunnel: w862 -> [w869]
        stop <- w904 continue-if-true
        w887 = 0
        n297 = for {
          tunnel: w902 -> [w933] mode=indexing
          i -> [w929]
          n298 = Get Notifier Status(notifier=w933) -> (current notification=w935:i8[])  [unwired: 1 in, 4 out]
          n299 = call "LVDimInterface.dim_unfold_data.vi"("rawData"=w935) -> ("data"=w934:i8[], "no link"=w932:bool)  [unwired: 15 in, 2 out]
          n300 = Type Cast(type=0.0, x=w934) -> (*(type *) &x=w930:dbl)
          n301 = case shown="False" w932 {
            tunnel: w930 -> [w937 _]
            tunnel: w929 -> [w936 _]
            frame False {
              n302 = local read "ScanValuesArray"() -> (w939:dbl[])
              n303 = Replace Array Subset(array=w939, new element=w937, index=w936) -> (w938:dbl[])
              n304 = local write "ScanValuesArray"(w938) -> ()
            }
            frame True {
            }
          }
        }
        n305 = Wait on Notification(notifier=w883, timeout in ms (-1)=50) -> (notification=w884:i8[], timed out?=w870:bool)  [unwired: 2 in, 2 out]
        n306 = for {
          tunnel: w869 -> [w911] mode=indexing
          i -> [w908]
          n307 = Get Notifier Status(notifier=w911) -> (current notification=w913:i8[])  [unwired: 1 in, 4 out]
          n308 = call "LVDimInterface.dim_unfold_data.vi"("rawData"=w913) -> ("data"=w912:i8[], "no link"=w910:bool)  [unwired: 15 in, 2 out]
          n309 = Type Cast(type="", x=w912) -> (*(type *) &x=w909:string)
          n310 = case shown="False" w910 {
            tunnel: w909 -> [w917 _]
            tunnel: w908 -> [w916 _]
            frame False {
              n311 = local read "ScanNamesArray"() -> (w915:string[])
              n312 = Replace Array Subset(array=w915, new element=w917, index=w916) -> (w914:string[])
              n313 = local write "ScanNamesArray"(w914) -> ()
            }
            frame True {
            }
          }
        }
        n314 = call "LVDimInterface.dim_unfold_data.vi"("rawData"=w884) -> ("data"=w873:i8[], "no link"=w871:bool)  [unwired: 15 in, 2 out]
        n315 = Or(x=w871, y=w870) -> (x .or. y?=w872:bool)
        n316 = case shown="False" w872 {
          tunnel: w873 -> [w920 _]
          tunnel: w882 -> [w922 _]
          frame False {
            n317 = Type Cast(type=i16 0, x=w920) -> (*(type *) &x=w919:i16)
            n318 = Greater Than 0?(x=w919) -> (x > 0?=w923:bool)
            n319 = case shown="True" w923 {
              tunnel: w922 -> [_ w925]
              frame False {
              }
              frame True {
                n320 = Generate User Event(user event=w925, event data cluster=TRUE ("event data")) -> ()  [unwired: 2 in, 2 out]
              }
            }
          }
          frame True {
          }
        }
        n321 = Index Array(array=w893) -> (element #1=w892:refnum<notifier>, element #2=w879:refnum<notifier>, element #3=w875:refnum<notifier>)  [unwired: 3 in]
        n322 = Get Notifier Status(notifier=w898) -> (current notification=w901:i8[])  [unwired: 1 in, 4 out]
        n323 = Get Notifier Status(notifier=w892) -> (current notification=w895:i8[])  [unwired: 1 in, 4 out]
        n324 = Get Notifier Status(notifier=w879) -> (current notification=w888:i8[])  [unwired: 1 in, 4 out]
        n325 = Get Notifier Status(notifier=w875) -> (current notification=w880:i8[])  [unwired: 1 in, 4 out]
        n326 = call "LVDimInterface.dim_unfold_data.vi"("rawData"=w901) -> ("data"=w900:i8[], "no link"=w897:bool)  [unwired: 15 in, 2 out]
        n327 = call "LVDimInterface.dim_unfold_data.vi"("rawData"=w895) -> ("data"=w894:i8[], "no link"=w891:bool)  [unwired: 15 in, 2 out]
        n328 = call "LVDimInterface.dim_unfold_data.vi"("rawData"=w888) -> ("data"=w889:i8[], "no link"=w885:bool)  [unwired: 15 in, 2 out]
        n329 = call "LVDimInterface.dim_unfold_data.vi"("rawData"=w880) -> ("data"=w881:i8[], "no link"=w878:bool)  [unwired: 15 in, 2 out]
        n330 = Type Cast(type=i16 0, x=w900) -> (*(type *) &x=w896:i16)
        n331 = Type Cast(type=w887, x=w894) -> (*(type *) &x=w890:i32)
        n332 = Type Cast(type=w887, x=w889) -> (*(type *) &x=w886:i32)
        n333 = Type Cast(type=0.0, x=w881) -> (*(type *) &x=w876:dbl)
        n334 = case shown="False" w897 {
          tunnel: w896 -> [w928 _]
          frame False {
            n335 = local write "ActDimensions"(w928) -> ()
          }
          frame True {
          }
        }
        n336 = case shown="False" w891 {
          tunnel: w890 -> [w927 _]
          frame False {
            "SNofSteps" <- w927
          }
          frame True {
          }
        }
        n337 = case shown="False" w885 {
          tunnel: w886 -> [w926 _]
          frame False {
            "SActStep" <- w926
          }
          frame True {
          }
        }
        n338 = case shown="False" w878 {
          tunnel: w876 -> [w918 _]
          frame False {
            "ScanMin" <- w918
          }
          frame True {
          }
        }
        n339 = Wait on Occurrence(1:FALSE ("ignore previous (T)"), 2:w903, 3:50 ("ms timeout (-1)")) -> (0:w904:bool)
      }
    }
    frame #5 {
      n340 = Build Array (concatenate)(w947, w946, w945) -> (w944:refnum<notifier>[])
      n341 = Build Array (concatenate)(w943, w942, w941) -> (w940:i32[])
      n342 = for {
        tunnel: w940 -> [w949] mode=indexing
        tunnel: w944 -> [w948] mode=indexing
        n343 = call "LVDimInterface.dic_release_service.vi"("callBackID"=w949) -> ()  [unwired: 18 in, 1 out]
        n344 = Release Notifier(notifier=w948) -> ()  [unwired: 2 in, 3 out]
      }
    }
  }
  n345 = while "Time Loop" {
    tunnel: w78 -> [w952]
    i -> [w951]
    stop <- w953 continue-if-true
    n346 = Get Date/Time In Seconds() -> (seconds since 1Jan1904=→"Time Stamp":timestamp)
    n347 = Wait on Occurrence(1:FALSE ("ignore previous (T)"), 2:w952, 3:1000 ("ms timeout (-1)")) -> (0:w953:bool)
    "Time Loop" <- w951
  }
  n348 = while "Analysis Event Loop" {
    tunnel: w60 -> [w994]
    shift-right: [w991] -> _
    shift-left: w168 -> [w993]
    shift-right: [w990] -> _
    shift-left: w167 -> [w992]
    tunnel: [w989] -> w165
    shift-right: [w979] -> w159
    shift-left: w151 -> [w984]
    tunnel: w150 -> [w987]
    shift-right: [w981] -> _
    shift-left: w116 -> [w983]
    shift-right: [w980] -> _
    shift-left: w115 -> [w982]
    tunnel: w79 -> [w978]
    shift-right: [w976] -> _
    shift-left: w62 -> [w977]
    shift-right: [w974] -> _
    shift-left: w61 -> [w975]
    shift-right: [w973] -> _
    shift-left: _ -> [w971]
    shift-right: [w972] -> _
    shift-left: _ -> [w970]
    shift-right: [w968] -> _
    shift-left: w59 -> [w969]
    tunnel: w46 -> [w967]
    tunnel: w45 -> [w966]
    tunnel: w39 -> [w965]
    shift-right: [w964] -> _
    shift-left: _ -> [w963]
    shift-right: [w962] -> _
    shift-left: _ -> [w961]
    shift-right: [w959] -> _
    shift-left: w25 -> [w960]
    shift-right: [w957] -> _
    shift-left: w24 -> [w958]
    tunnel: w2 -> [w956]
    i -> [w988]
    stop <- w986 stop-if-true
    n349 = case shown="No Error" w984 {
      selector: w984 -> [w1021 w2210]
      tunnel: w994 -> [w1032 w2207]
      tunnel: w993 -> [w1031 w2208]
      tunnel: w992 -> [w1030 w2206]
      tunnel: [w1029 w2208] -> w991
      tunnel: [w1028 w2206] -> w990
      tunnel: [w1027 w2207] -> w989
      tunnel: w987 -> [w1026 w2213]
      tunnel: [w1025 w2212] -> w986
      tunnel: w966 -> [w1024 _]
      tunnel: -1 -> [w1023 w2211]
      tunnel: [w1022 w2209] -> w979
      tunnel: w983 -> [w1020 w2205]
      tunnel: w982 -> [w1019 w2204]
      tunnel: [w1018 w2205] -> w981
      tunnel: [w1017 w2204] -> w980
      tunnel: w978 -> [w1016 _]
      tunnel: w977 -> [w1014 w2203]
      tunnel: [w1015 w2203] -> w976
      tunnel: w975 -> [w1013 w2200]
      tunnel: [w1012 w2200] -> w974
      tunnel: [w1011 w2202] -> w973
      tunnel: [w1010 w2201] -> w972
      tunnel: w971 -> [w1009 w2202]
      tunnel: w970 -> [w1008 w2201]
      tunnel: w969 -> [w1007 w2199]
      tunnel: [w1006 w2199] -> w968
      tunnel: w967 -> [w1005 _]
      tunnel: w965 -> [w1004 _]
      tunnel: [w1003 _] -> w964
      tunnel: w963 -> [w1002 _]
      tunnel: [w1001 _] -> w962
      tunnel: w961 -> [w1000 _]
      tunnel: w960 -> [w999 w2198]
      tunnel: [w998 w2198] -> w959
      tunnel: w958 -> [w997 w2197]
      tunnel: [w996 w2197] -> w957
      tunnel: w956 -> [w995 _]
      frame No Error {
        n350 = event shown="[4] <Analysis Step 2>: User Event" {
          selector: w1026 -> [_ _ _ _ _ _ _ _]
          dyn-events: _ -> [_ _ _ _ _ _ _ _]
          timeout: w1023 -> [_ _ _ _ _ _ _ _]
          tunnel: w1032 -> [w1045 w1062 w1072 w1119 w1243 w2077 w2163 w2192]
          tunnel: w1031 -> [w1047 w1060 w1086 w1122 w1247 w2095 w2159 w2194]
          tunnel: w1030 -> [w1046 w1061 w1084 w1121 w1250 w2087 w2155 w2191]
          tunnel: w1021 -> [w1044 w1063 _ w1126 _ w2097 w2164 w2196]
          tunnel: [w1047 w1060 w1078 w1122 w1232 w2093 w2158 w2194] -> w1029
          tunnel: [w1046 w1061 w1075 w1121 w1231 w2084 w2154 w2191] -> w1028
          tunnel: [w1045 w1062 w1072 w1118 w1234 w2076 w2163 w2192] -> w1027
          tunnel: [w1044 w1063 _ w1126 _ w2096 w2164 w2196] -> w1022
          tunnel: [_ TRUE _ _ _ _ _ _] -> w1025
          tunnel: w1024 -> [_ _ _ w1117 w1242 _ _ _]
          tunnel: w1020 -> [w1043 w1058 w1088 w1125 w1238 w2091 w2161 w2195]
          tunnel: w1019 -> [w1042 w1057 w1087 w1124 w1237 w2090 w2160 w2193]
          tunnel: [w1043 w1058 w1077 w1125 w1228 w2089 w2157 w2195] -> w1018
          tunnel: [w1042 w1057 w1076 w1124 w1227 w2088 w2156 w2193] -> w1017
          tunnel: w1016 -> [_ _ _ w1114 w1252 _ _ _]
          tunnel: [w1041 w1056 w1079 w1123 w1233 w2092 w2152 w2188] -> w1015
          tunnel: w1014 -> [w1041 w1056 w1085 w1123 w1245 w2094 w2153 w2188]
          tunnel: w1013 -> [w1040 w1055 w1083 w1120 w1249 w2086 w2151 w2187]
          tunnel: [w1040 w1055 w1074 w1120 w1230 w2083 w2150 w2187] -> w1012
          tunnel: [w1038 w1053 w1081 w1115 w1236 w2104 w2148 w2185] -> w1011
          tunnel: [w1037 w1052 w1080 w1110 w1235 w2102 w2146 w2184] -> w1010
          tunnel: w1009 -> [w1038 w1053 w1090 w1115 w1226 w2105 w2149 w2185]
          tunnel: w1008 -> [w1037 w1052 w1089 w1110 w1225 w2103 w2147 w2184]
          tunnel: w1007 -> [w1039 w1054 w1082 w1113 w1241 w2085 _ w2186]
          tunnel: [w1039 w1054 w1073 w1113 w1229 w2082 _ w2186] -> w1006
          tunnel: w1005 -> [_ _ _ _ _ _ _ _]
          tunnel: w1004 -> [_ _ _ _ w1222 _ _ _]
          tunnel: [w1035 w1050 w1068 w1111 w1221 w2098 w2142 w2181] -> w1003
          tunnel: w1002 -> [w1035 w1050 w1070 w1111 _ w2100 w2144 w2181]
          tunnel: [w1036 w1051 w1069 w1112 w1220 w2099 w2143 w2182] -> w1001
          tunnel: w1000 -> [w1036 w1051 w1071 w1112 _ w2101 w2145 w2182]
          tunnel: w999 -> [w1034 w1049 w1067 w1109 w1215 w2081 w2140 w2180]
          tunnel: [w1034 w1049 w1066 w1109 w1214 w2079 w2141 w2180] -> w998
          tunnel: w997 -> [w1033 w1048 w1064 w1108 w1212 w2080 w2138 w2179]
          tunnel: [w1033 w1048 w1065 w1108 w1211 w2078 w2139 w2179] -> w996
          tunnel: w995 -> [_ _ _ _ w1210 w2075 _ _]
          event Timeout {
            n351 = event-data() -> ()  [unwired: 1 in, 1 out]
          }
          event User Event {
            n352 = event-data() -> ()  [unwired: 1 in, 1 out]
          }
          event "Clear Analysis button": Value Change {
            n353 = event-data() -> ("NewVal"=w1091:bool)  [unwired: 1 in]
            n354 = local write "Clear Analysis button"(FALSE ("Clear Analysis button")) -> ()
            n355 = case shown="True" w1091 {
              tunnel: w1090 -> [w1105 _]
              tunnel: w1089 -> [w1104 _]
              tunnel: w1088 -> [w1101 w1107]
              tunnel: w1087 -> [w1100 w1106]
              tunnel: w1086 -> [w1102 _]
              tunnel: w1085 -> [w1103 _]
              tunnel: w1084 -> [w1099 _]
              tunnel: w1083 -> [w1098 _]
              tunnel: w1082 -> [w1097 _]
              tunnel: [w1105 _] -> w1081
              tunnel: [w1104 _] -> w1080
              tunnel: [w1103 _] -> w1079
              tunnel: [w1102 _] -> w1078
              tunnel: [w1101 w1107] -> w1077
              tunnel: [w1100 w1106] -> w1076
              tunnel: [w1099 _] -> w1075
              tunnel: [w1098 _] -> w1074
              tunnel: [w1097 _] -> w1073
              tunnel: w1071 -> [w1096 _]
              tunnel: w1070 -> [w1095 _]
              tunnel: [w1096 _] -> w1069
              tunnel: [w1095 _] -> w1068
              tunnel: w1067 -> [w1094 _]
              tunnel: [w1094 _] -> w1066
              tunnel: [w1093 _] -> w1065
              tunnel: w1064 -> [w1093 _]
              frame False {
              }
              frame True {
              }
            }
          }
          event "Analysis Mode": Value Change {
            n356 = event-data() -> ("NewVal"=w1116:T4)  [unwired: 1 in]
            n357 = case shown="True" w1117 {
              tunnel: w1119 -> [w1127 w1135]
              tunnel: [w1127 w1140] -> w1118
              tunnel: w1116 -> [_ w1139]
              tunnel: w1115 -> [_ w1138]
              tunnel: w1110 -> [_ w1128]
              tunnel: w1114 -> [_ w1136]
              tunnel: w1113 -> [_ w1133]
              tunnel: w1111 -> [_ w1130]
              tunnel: w1112 -> [_ w1129]
              frame False {
              }
              frame True {
                w1131 = 449  # ScanImage Width in Pixel
                w1132 = 379  # ScanImage Height in Pixel
                n358 = local read "Acquisition mode (Buffer)"() -> (w1134:T2)
                n359 = case shown="\"Horizontal Projection\", Default" w1139 {
                  tunnel: w1138 -> [_ w1194]
                  tunnel: [w1160 w1194] -> w1137
                  tunnel: w1128 -> [w1160 _]
                  tunnel: w1136 -> [w1153 w1187]
                  tunnel: w1134 -> [w1149 w1180]
                  tunnel: w1133 -> [w1148 w1179]
                  tunnel: w1132 -> [w1144 _]
                  tunnel: w1131 -> [_ w1178]
                  tunnel: w1130 -> [w1142 _]
                  tunnel: w1129 -> [_ w1175]
                  frame "Horizontal Projection", Default {
                    n360 = call "IMAQController.get i attribute.vi"("i ref in"=w1153) -> ("i attribute"=w1159:T17)  [unwired: 16 in, 2 out]
                    n361 = case shown="\"Scan\"" w1149 {
                      tunnel: [w1162 w1173] -> w1147
                      tunnel: w1148 -> [w1167 _]
                      tunnel: ["Measurement Number" ("X Scale.Name Label.Text") w1171] -> w1145
                      tunnel: [w1163 w1172] -> w1146
                      tunnel: w1144 -> [w1161 _]
                      frame Default {
                        n362 = Increment(x=w1167) -> (x+1=w1162:i32)
                        n363 = Greater?(x=w1162, y=w1161) -> (0:w1166:bool)
                        n364 = Subtract(x=w1162, y=w1161) -> (x-y=w1165:i32)
                        n365 = Select(t=w1165, s=w1166, f=0) -> (s? t:f=w1163:i32)
                      }
                      frame "Scan" {
                        w1170 = 0
                        n366 = local read "ScanValuesArray"() -> (w1174:dbl[])
                        n367 = local read "ScanNamesArray"() -> (w1169:string[])
                        n368 = local read "ScanMin"() -> (w1172:dbl)
                        n369 = Index Array(array=w1174, index=w1170) -> (element=w1173:dbl)
                        n370 = Index Array(array=w1169, index=w1170) -> (element=w1171:string)
                      }
                    }
                    n371 = Unbundle By Name(w1159) -> ("activeCamera.Center Coordinates.Horizontal"=w1154:i32, "activeCamera.PixelPermm.Horizontal"=w1156:dbl)
                    n372 = local read "AnaWidth"() -> (w1141:i32)
                    n373 = Subtract(x=w1141, y=w1154) -> (x-y=w1158:i32)
                    n374 = Reciprocal(x=w1156) -> (1/x=w1155:dbl)
                    n375 = Negate(x=w1154) -> (-x=w1157:i32)
                    n376 = Multiply(x=w1142, y=w1147) -> (x*y=w1143:dbl)
                    n377 = Multiply(x=w1158, y=w1155) -> (x*y=w1150:dbl)
                    n378 = Multiply(x=w1155, y=w1157) -> (x*y=w1151:dbl)
                    n379 = property on="HilfsplotProj" class="XYGraph (strict)"("XScale.Maximum"=w1150, "XScale.Minimum"=w1151, "XScale.NameLbl.Text"="horizontal position / mm" ("X Scale.Name Label.Text"), "YScale.Maximum"=w1143, "YScale.Minimum"=w1146, "YScale.NameLbl.Text"=w1145) -> ()  [unwired: 2 in, 2 out]
                  }
                  frame "Vertical Projection" {
                    n380 = call "IMAQController.get i attribute.vi"("i ref in"=w1187) -> ("i attribute"=w1193:T17)  [unwired: 16 in, 2 out]
                    n381 = Unbundle By Name(w1193) -> ("activeCamera.Center Coordinates.Vertical"=w1188:i32, "activeCamera.PixelPermm.Vertical"=w1190:dbl)
                    n382 = case shown="\"Scan\"" w1180 {
                      tunnel: [w1196 w1207] -> w1183
                      tunnel: w1179 -> [w1201 _]
                      tunnel: ["Measurement Number" ("X Scale.Name Label.Text") w1205] -> w1181
                      tunnel: [w1197 w1206] -> w1182
                      tunnel: w1178 -> [w1195 _]
                      frame Default {
                        n383 = Increment(x=w1201) -> (x+1=w1196:i32)
                        n384 = Greater?(x=w1196, y=w1195) -> (0:w1200:bool)
                        n385 = Subtract(x=w1196, y=w1195) -> (x-y=w1199:i32)
                        n386 = Select(t=w1199, s=w1200, f=0) -> (s? t:f=w1197:i32)
                      }
                      frame "Scan" {
                        w1204 = 0
                        n387 = local read "ScanValuesArray"() -> (w1208:dbl[])
                        n388 = local read "ScanNamesArray"() -> (w1203:string[])
                        n389 = local read "ScanMin"() -> (w1206:dbl)
                        n390 = Index Array(array=w1208, index=w1204) -> (element=w1207:dbl)
                        n391 = Index Array(array=w1203, index=w1204) -> (element=w1205:string)
                      }
                    }
                    n392 = local read "AnaHeight"() -> (w1176:i32)
                    n393 = Subtract(x=w1176, y=w1188) -> (x-y=w1192:i32)
                    n394 = Reciprocal(x=w1190) -> (1/x=w1189:dbl)
                    n395 = Negate(x=w1188) -> (-x=w1191:i32)
                    n396 = Multiply(x=w1175, y=w1183) -> (x*y=w1177:dbl)
                    n397 = Multiply(x=w1192, y=w1189) -> (x*y=w1184:dbl)
                    n398 = Multiply(x=w1189, y=w1191) -> (x*y=w1185:dbl)
                    n399 = property on="HilfsplotProj" class="XYGraph (strict)"("YScale.Maximum"=w1184, "YScale.Minimum"=w1185, "YScale.NameLbl.Text"="vertical position / mm" ("X Scale.Name Label.Text"), "XScale.Maximum"=w1177, "XScale.Minimum"=w1182, "XScale.NameLbl.Text"=w1181) -> ()  [unwired: 2 in, 2 out]
                  }
                }
                n400 = call "IMAQ ArrayToImage"("Image Pixels (U8)"=w1137, "Image"=w1135) -> ("Image Out"=w1140:T3)  [unwired: 8 in, 1 out]
                n401 = local write "ScanImage"(w1140) -> ()
              }
            }
          }
          event User Event {
            n402 = event-data() -> ("Data"=w1251:u8[][], "Height"=w1240:i32, "Width"=w1239:i32, "Save path out Scan"=w1248:path, "Save path out Horizontal"=w1224:path, "Save path out Vertical"=w1223:path, "Scan?"=w1253:bool, "Scan running?"=w1246:bool, "ROI Calculation?"=w1213:bool, "Starting Mouse Position 1"=w1257:cluster{"X":i32, "Y":i32}, "End Mouse Position 1"=w1256:cluster{"X":i32, "Y":i32}, "Starting Mouse Position 2"=w1255:cluster{"X":i32, "Y":i32}, "End Mouse Position 2"=w1254:cluster{"X":i32, "Y":i32}, "do analysis?"=w1219:bool, "ScanValuesArray"=w1218:dbl[], "ActDimensions"=w1217:i16, "ScanNamesArray"=w1216:string[], "Av repeat?"=w1209:bool)  [unwired: 1 in]
            n403 = stacked-sequence {
              seq-local: [_ _ _ w1443 _ _ _ _ _ _] -> [_ _ _ _ _ w1695 _ _ _ _]
              seq-local: [_ _ _ _ w1574 _ _ _ _ _] -> [_ _ _ _ _ w1694 _ _ _ _]
              seq-local: [_ _ w1429 _ _ _ _ _ _ _] -> [_ _ _ w1441 w1573 w1688 _ _ _ _]
              seq-local: [_ _ w1428 _ _ _ _ _ _ _] -> [_ _ _ w1442 w1572 w1689 _ _ _ _]
              seq-local: [_ _ _ w1430 _ _ _ _ _ _] -> [_ _ _ _ _ w1687 _ _ _ _]
              seq-local: [_ _ _ _ w1562 _ _ _ _ _] -> [_ _ _ _ _ w1686 _ _ _ _]
              seq-local: [w1282 _ _ _ _ _ _ _ _ _] -> [_ w1376 _ _ _ _ w1811 _ _ _]
              seq-local: [_ w1371 _ _ _ _ _ _ _ _] -> [_ _ _ w1437 w1568 w1681 w1812 w1941 w2013 w2065]
              seq-local: [w1281 _ _ _ _ _ _ _ _ _] -> [_ _ _ _ _ _ w1805 w1939 _ _]
              seq-local: [_ _ _ _ _ _ w1801 _ _ _] -> [_ _ _ _ _ _ _ w1944 w2007 _]
              seq-local: [_ _ _ _ _ _ w1800 _ _ _] -> [_ _ _ _ _ _ _ w1943 w2008 _]
              seq-local: [_ _ _ _ _ _ w1799 _ _ _] -> [_ _ _ _ _ _ _ w1942 w2009 _]
              tunnel: w1243 -> [_ _ _ _ _ w1693 _ _ _ _]
              tunnel: [_ _ _ w1444 _ _ _ _ _ _] -> w1232
              tunnel: [_ _ _ w1440 _ _ _ _ _ _] -> w1231
              tunnel: [_ _ _ _ _ w1696 _ _ _ _] -> w1234
              tunnel: w1249 -> [_ _ _ _ w1569 _ _ _ _ _]
              tunnel: [_ _ _ _ w1571 _ _ _ _ _] -> w1230
              tunnel: [_ _ _ _ w1575 _ _ _ _ _] -> w1233
              tunnel: [_ _ _ w1443 _ _ _ _ _ _] -> w1236
              tunnel: [_ _ _ _ w1574 _ _ _ _ _] -> w1235
              tunnel: "Analysis Mode" -> [_ _ _ _ _ w1697 _ _ _ _]
              tunnel: w1252 -> [_ w1374 _ _ _ w1692 _ _ _ _]
              tunnel: w1241 -> [_ _ _ _ _ w1691 _ _ _ _]
              tunnel: [_ _ _ _ _ w1690 _ _ _ _] -> w1229
              tunnel: w1253 -> [_ w1375 _ w1439 w1570 w1685 w1813 w1938 w2010 _]
              tunnel: w1257 -> [w1286 _ _ _ _ _ _ _ _ _]
              tunnel: w1256 -> [w1285 _ _ _ _ _ _ _ _ _]
              tunnel: w1255 -> [w1284 _ _ _ _ _ _ _ _ _]
              tunnel: w1254 -> [w1283 _ _ _ _ _ _ _ _ _]
              tunnel: w1251 -> [w1280 _ _ w1438 w1566 _ _ _ _ w2064]
              tunnel: w1250 -> [_ _ _ w1436 _ _ _ _ _ _]
              tunnel: w1248 -> [_ _ _ w1435 w1565 _ _ w1937 _ _]
              tunnel: w1247 -> [_ _ _ w1434 _ _ _ _ _ _]
              tunnel: w1246 -> [_ _ _ w1433 w1567 _ _ _ _ _]
              tunnel: w1245 -> [_ _ _ _ w1564 _ _ _ _ _]
              tunnel: w1242 -> [_ _ _ _ _ w1684 _ _ _ _]
              tunnel: w1240 -> [_ w1373 _ _ _ w1683 _ _ _ w2063]
              tunnel: w1239 -> [_ w1372 _ _ _ w1682 _ _ _ w2062]
              tunnel: w1238 -> [_ _ _ _ _ _ w1810 _ _ _]
              tunnel: w1237 -> [_ _ _ _ _ _ w1809 _ _ _]
              tunnel: [_ _ _ _ _ _ w1801 _ _ _] -> w1228
              tunnel: [_ _ _ _ _ _ w1800 _ _ _] -> w1227
              tunnel: w1226 -> [_ _ _ w1432 _ _ _ _ _ _]
              tunnel: w1225 -> [_ _ _ w1431 w1563 _ _ _ _ _]
              tunnel: w1224 -> [_ _ _ _ _ _ _ _ _ w2061]
              tunnel: w1223 -> [_ _ _ _ _ _ _ _ _ w2059]
              tunnel: w1222 -> [_ _ _ _ _ _ _ _ _ w2060]
              tunnel: [_ _ _ _ w1562 _ _ _ _ _] -> w1221
              tunnel: [_ _ _ w1430 _ _ _ _ _ _] -> w1220
              tunnel: w1219 -> [_ w1369 _ _ _ _ _ _ _ _]
              tunnel: w1218 -> [_ _ _ _ _ w1680 w1808 _ _ _]
              tunnel: w1217 -> [_ _ _ _ _ _ w1807 w1935 w2012 _]
              tunnel: w1216 -> [_ _ _ _ _ w1679 w1806 w1936 w2011 _]
              tunnel: w1215 -> [_ _ _ _ _ _ w1804 _ _ _]
              tunnel: [_ _ _ _ _ _ w1799 _ _ _] -> w1214
              tunnel: w1213 -> [w1258 _ _ _ _ _ _ _ _ _]
              tunnel: w1212 -> [_ _ _ _ _ _ w1803 _ _ _]
              tunnel: [_ _ _ _ _ _ w1802 _ _ _] -> w1211
              tunnel: w1210 -> [_ _ _ _ _ _ _ _ w2006 _]
              tunnel: w1209 -> [_ w1370 _ _ _ _ _ _ _ _]
              frame #0 {
                # "noetig, wenn Maus von \nUR nach OL bewegt wird"
                # "Calculate ROIs (necessary also to check for lower limit)"
                n404 = Unbundle By Name(w1286) -> ("X"=w1267:i32, "Y"=w1266:i32)
                n405 = Unbundle By Name(w1285) -> ("X"=w1265:i32, "Y"=w1264:i32)
                n406 = Unbundle By Name(w1284) -> ("X"=w1263:i32, "Y"=w1262:i32)
                n407 = Unbundle By Name(w1283) -> ("X"=w1261:i32, "Y"=w1260:i32)
                n408 = Compound Arithmetic op=ADD(w1267, w1266, w1265, w1264, w1263, w1262, w1261, w1260) -> (w1259:i32)
                n409 = Less Or Equal?(x=w1267, y=w1265) -> (x <= y?=w1268:bool)
                n410 = Less Or Equal?(x=w1266, y=w1264) -> (x <= y?=w1271:bool)
                n411 = Less Or Equal?(x=w1263, y=w1261) -> (x <= y?=w1275:bool)
                n412 = Less Or Equal?(x=w1262, y=w1260) -> (x <= y?=w1274:bool)
                n413 = Not Equal To 0?(x=w1259) -> (x != 0?=w1281:bool)
                n414 = case shown="True" w1268 {
                  tunnel: w1267 -> [w1366 w1368]
                  tunnel: w1265 -> [w1365 w1367]
                  tunnel: [w1365 w1368] -> w1269
                  tunnel: [w1366 w1367] -> w1270
                  frame False {
                  }
                  frame True {
                  }
                }
                n415 = case shown="True" w1271 {
                  tunnel: w1266 -> [w1362 w1364]
                  tunnel: w1264 -> [w1361 w1363]
                  tunnel: [w1361 w1364] -> w1272
                  tunnel: [w1362 w1363] -> w1273
                  frame False {
                  }
                  frame True {
                  }
                }
                n416 = case shown="True" w1275 {
                  tunnel: w1263 -> [w1358 w1360]
                  tunnel: w1261 -> [w1357 w1359]
                  tunnel: [w1357 w1360] -> w1276
                  tunnel: [w1358 w1359] -> w1277
                  frame False {
                  }
                  frame True {
                  }
                }
                n417 = case shown="True" w1274 {
                  tunnel: w1262 -> [w1354 w1356]
                  tunnel: w1260 -> [w1353 w1355]
                  tunnel: [w1353 w1356] -> w1278
                  tunnel: [w1354 w1355] -> w1279
                  frame False {
                  }
                  frame True {
                  }
                }
                n418 = local write "TL2x"(w1276) -> ()
                n419 = local write "TL2y"(w1278) -> ()
                n420 = local write "BR2x"(w1277) -> ()
                n421 = local write "BR2y"(w1279) -> ()
                n422 = local write "TL1x"(w1269) -> ()
                n423 = local write "TL1y"(w1272) -> ()
                n424 = local write "BR1x"(w1270) -> ()
                n425 = local write "BR1y"(w1273) -> ()
                n426 = case shown="True" w1258 {
                  tunnel: [_ w1310] -> w1282
                  tunnel: w1280 -> [_ w1309]
                  tunnel: w1279 -> [_ w1308]
                  tunnel: w1278 -> [_ w1307]
                  tunnel: w1277 -> [_ w1306]
                  tunnel: w1276 -> [_ w1305]
                  tunnel: w1273 -> [_ w1304]
                  tunnel: w1272 -> [_ w1303]
                  tunnel: w1270 -> [_ w1302]
                  tunnel: w1269 -> [_ w1301]
                  frame False {
                  }
                  frame True {
                    n427 = Subtract(x=w1304, y=w1303) -> (x-y=w1299:i32)
                    n428 = Subtract(x=w1302, y=w1301) -> (x-y=w1298:i32)
                    n429 = Subtract(x=w1308, y=w1307) -> (x-y=w1297:i32)
                    n430 = Subtract(x=w1306, y=w1305) -> (x-y=w1296:i32)
                    n431 = Array Subset(array=w1309, index (row)=w1303, length (row)=w1299, index (col)=w1301, length (col)=w1298) -> (w1293:u8[][])
                    n432 = Array Subset(array=w1309, index (row)=w1307, length (row)=w1297, index (col)=w1305, length (col)=w1296) -> (w1295:u8[][])
                    n433 = Array Size(array=w1293) -> (size(s)=w1300:i32[])
                    n434 = Multiply Array Elements(1:w1300) -> (0:w1287:i32)
                    n435 = Reshape Array(w1293, w1287) -> (w1294:u8[])
                    n436 = case shown="Default" w1287 {
                      selector: w1287 -> [_ w1349]
                      tunnel: w1294 -> [_ w1348]
                      tunnel: "Offset" -> [_ w1350]
                      tunnel: [0.0 w1352] -> w1291
                      frame 0 {
                      }
                      frame Default {
                        n437 = To Long Integer(number=w1348) -> (32bit integer=w1347:i32[])
                        n438 = Add Array Elements(numeric array=w1347) -> (sum=w1346:i32)
                        n439 = Multiply(x=w1349, y=w1350) -> (x*y=w1351:dbl)
                        n440 = Subtract(x=w1346, y=w1351) -> (x-y=w1352:dbl)
                      }
                    }
                    "ROI 1" <- w1291
                    n441 = case shown="False" "ROI2notROI1Boolen" {
                      tunnel: w1295 -> [w1325 _]
                      tunnel: "Offset" -> [w1324 w1341]
                      tunnel: [w1323 w1337] -> w1290
                      tunnel: w1291 -> [_ w1336]
                      tunnel: w1309 -> [_ w1335]
                      frame False {
                        n442 = Array Size(array=w1325) -> (size(s)=w1322:i32[])
                        n443 = Multiply Array Elements(1:w1322) -> (0:w1321:i32)
                        n444 = Reshape Array(w1325, w1321) -> (w1326:u8[])
                        n445 = case shown="Default" w1321 {
                          selector: w1321 -> [_ w1331]
                          tunnel: w1326 -> [_ w1330]
                          tunnel: w1324 -> [_ w1332]
                          tunnel: [0.0 w1334] -> w1323
                          frame 0 {
                          }
                          frame Default {
                            n446 = To Long Integer(number=w1330) -> (32bit integer=w1329:i32[])
                            n447 = Add Array Elements(numeric array=w1329) -> (sum=w1328:i32)
                            n448 = Multiply(x=w1331, y=w1332) -> (x*y=w1333:dbl)
                            n449 = Subtract(x=w1328, y=w1333) -> (x-y=w1334:dbl)
                          }
                        }
                      }
                      frame True {
                        n450 = To Long Integer(number=w1335) -> (32bit integer=w1344:i32[][])
                        n451 = Array Size(array=w1335) -> (size(s)=w1343:i32[])
                        n452 = Add Array Elements(numeric array=w1344) -> (sum=w1340:i32)
                        n453 = Multiply Array Elements(1:w1343) -> (0:w1342:i32)
                        n454 = Multiply(x=w1341, y=w1342) -> (x*y=w1339:dbl)
                        n455 = Subtract(x=w1340, y=w1339) -> (x-y=w1338:dbl)
                        n456 = Subtract(x=w1338, y=w1336) -> (x-y=w1337:dbl)
                      }
                    }
                    "ROI 2" <- w1290
                    n457 = case shown="\"Radio Selection 1\"" "ROI Choice" {
                      tunnel: [w1312 w1316] -> w1310
                      tunnel: w1291 -> [w1313 w1315]
                      tunnel: w1290 -> [_ w1314]
                      tunnel: w1287 -> [w1311 _]
                      frame "Radio Selection 1" {
                        n458 = Divide(x=w1313, y=w1311) -> (x/y=w1312:dbl)
                      }
                      frame "Radio Selection 2", Default {
                        n459 = case shown="0" w1314 {
                          tunnel: w1315 -> [_ w1320]
                          tunnel: w1314 -> [_ w1319]
                          tunnel: [0.0 w1318] -> w1316
                          frame 0 {
                          }
                          frame Default {
                            n460 = Divide(x=w1320, y=w1319) -> (x/y=w1318:dbl)
                          }
                        }
                      }
                    }
                    "ROI 1 / ROI 2" <- w1310
                  }
                }
              }
              frame #1 {
                # "Check if Analysis necessary or scan step has to be repeated"
                n461 = case shown="True" w1369 {
                  tunnel: w1376 -> [_ w1398]
                  tunnel: w1375 -> [_ w1381]
                  tunnel: w1374 -> [_ w1397]
                  tunnel: [_ w1385] -> w1371
                  tunnel: w1370 -> [_ w1380]
                  frame False {
                  }
                  frame True {
                    # "repeat because of averaging"
                    # "Eigentlich muss zuerst auf \"Repeat durch Averaging\" \nund dann auf \"Repeat durch lower limit\" getestet \nwerden, deshalb wurde der Repeat Boolean rausgezogen"
                    # "The value will be set to 0 again with a\nspecial command in ProcCases!\n\n1 means ImageTaken and publised\n2 means ImageTaken but not published\nbecause waiting for other images to\ncalculate average or repeat because\nactvalue lower than lower limit"
                    n462 = Not(x=w1380) -> (.not. x?=w1379:bool)
                    n463 = call "IMAQController.get i attribute.vi"("i ref in"=w1397) -> ("i ref out"=w1396:refnum<vi>, "i attribute"=w1393:T17)  [unwired: 16 in, 1 out]
                    n464 = Unbundle By Name(w1393) -> ("ImageTakenID"=w1395:i32, "BilderMittelungen"=w1394:u8)
                    n465 = local read "auto repeat scan step"() -> (w1389:bool)
                    n466 = local read "lower limit"() -> (w1388:dbl)
                    n467 = Less Or Equal?(x=w1398, y=w1388) -> (x <= y?=w1390:bool)
                    n468 = And(x=w1389, y=w1390) -> (x .and. y?=w1391:bool)
                    n469 = And(x=w1381, y=w1391) -> (x .and. y?=w1384:bool)
                    n470 = Not(x=w1380) -> (.not. x?=w1383:bool)
                    n471 = And(x=w1384, y=w1383) -> (x .and. y?=w1382:bool)
                    n472 = case "Repeat because of lower limit" shown="False" w1382 {
                      tunnel: [w1408 i16 2 ("x")] -> w1392
                      tunnel: w1394 -> [_ w1412]
                      tunnel: w1396 -> [_ w1411]
                      tunnel: [w1406 _] -> w1386
                      tunnel: [w1404 u32 16711680] -> w1387
                      tunnel: w1380 -> [w1402 _]
                      frame False {
                        w1406 = TRUE  # Do analysis
                        n473 = Select(t=i16 2 ("x"), s=w1402, f=i16 1 ("x")) -> (s? t:f=w1408:i16)
                        n474 = Select(t=u32 16753426, s=w1402, f=u32 0) -> (s? t:f=w1404:u32)
                      }
                      frame True {
                        n475 = case shown="Default" w1412 {
                          selector: w1412 -> [_ w1415]
                          tunnel: w1411 -> [_ w1420]
                          frame 0 {
                          }
                          frame Default {
                            n476 = call "IMAQController.get data to modify.vi"("i ref in"=w1420) -> ("i ref out"=w1419:refnum<vi>, "i attribute"=w1416:T17, "timed out"=w1417:bool, "error out"=w1418:errorcluster)  [unwired: 15 in]
                            n477 = Decrement(x=w1415) -> (x-1=w1414:u8)
                            n478 = case shown="False" w1417 {
                              tunnel: w1419 -> [w1426 _]
                              tunnel: w1418 -> [w1425 w1427]
                              tunnel: w1416 -> [w1424 _]
                              tunnel: w1414 -> [w1422 _]
                              tunnel: [w1421 w1427] -> _
                              frame False {
                                n479 = Bundle By Name(cluster=w1424, "BilderMittelungen"=w1422) -> (w1423:T17)
                                n480 = call "IMAQController.set modified data.vi"("i ref in"=w1426, "i attribute"=w1423, "error in (no error)"=w1425) -> ("error out"=w1421:errorcluster)  [unwired: 15 in, 1 out]
                              }
                              frame True {
                              }
                            }
                          }
                        }
                      }
                    }
                    n481 = And(x=w1379, y=w1386) -> (x .and. y?=w1385:bool)
                    n482 = local read "MeasurementNo"() -> (w1378:i32)
                    n483 = property on="ROI 1 / ROI 2" class="DigNum (strict)"("NumText.TextColor"=w1387) -> ()  [unwired: 2 in, 2 out]
                    n484 = property on="MeasurementNo" class="DigNum (strict)"("NumText.TextColor"=w1387) -> ()  [unwired: 2 in, 2 out]
                    n485 = Increment(x=w1378) -> (x+1=w1377:i32)
                    n486 = local write "MeasurementNo"(w1377) -> ()
                    n487 = case shown="True" w1381 {
                      tunnel: w1395 -> [_ w1401]
                      tunnel: w1392 -> [_ w1400]
                      frame False {
                      }
                      frame True {
                        n488 = Type Cast(x=w1400) -> (*(type *) &x=w1399:string)  [unwired: 1 in]
                        n489 = call "LVDimInterface.dis_update_service.vi"("my_serviceID"=w1401, "data"=w1399) -> ()  [unwired: 15 in, 3 out]
                      }
                    }
                  }
                }
                "AnaHeight" <- w1373
                "AnaWidth" <- w1372
              }
              frame #2 {
                w1428 = 379  # ScanImage Height in Pixel
                w1429 = 449  # ScanImage Width in Pixel
              }
              frame #3 {
                n490 = case shown="True" w1437 {
                  tunnel: [w1446 w1495] -> w1444
                  tunnel: [w1447 w1467] -> w1443
                  tunnel: w1442 -> [_ w1463]
                  tunnel: w1441 -> [_ w1458]
                  tunnel: [_ w1456] -> w1430
                  tunnel: [w1445 w1454] -> w1440
                  tunnel: w1439 -> [_ w1453]
                  tunnel: w1438 -> [_ w1452]
                  tunnel: w1436 -> [w1445 w1451]
                  tunnel: w1435 -> [_ w1450]
                  tunnel: w1434 -> [w1446 w1449]
                  tunnel: w1433 -> [_ w1448]
                  tunnel: w1432 -> [w1447 _]
                  tunnel: w1431 -> [_ _]
                  frame False {
                  }
                  frame True {
                    w1475 = i32[][] [] ("Analysis Data")
                    w1491 = 255  # MaxPixel
                    # "hier wird ausgabe\nvertikal gestaucht"
                    # "Plot fraction needed\nfor data"
                    # "das hier \nspeichern!"
                    # "neues Scanbild"
                    # "Vertical HeatPlot"
                    n491 = Array Size(array=w1452) -> (size(s)=w1494:i32[])
                    n492 = Index Array(array=w1494, index #1=0 ("index")) -> (element #1=w1474:i32, element #2=w1492:i32)  [unwired: 1 in]
                    n493 = for {
                      N: w1474 -> [_]
                      tunnel: w1452 -> [w1555]
                      tunnel: [w1553] -> w1455 mode=indexing
                      tunnel: w1492 -> [w1552]
                      i -> [w1551]
                      n494 = for {
                        N: w1552 -> [_]
                        tunnel: w1555 -> [w1561]
                        tunnel: w1551 -> [w1556]
                        shift-right: [w1558] -> w1553
                        shift-left: 0 -> [w1559]
                        i -> [w1557]
                        n495 = Index Array(array=w1561, index (row)=w1556, index (col)=w1557) -> (element=w1560:u8)
                        n496 = Add(x=w1559, y=w1560) -> (x+y=w1558:i32)
                      }
                    }
                    n497 = case shown="True" w1453 {
                      tunnel: w1455 -> [_ w1500]
                      tunnel: w1448 -> [_ w1498]
                      tunnel: w1450 -> [_ w1497]
                      frame False {
                      }
                      frame True {
                        n498 = local read "auto save"() -> (w1496:bool)
                        n499 = And(x=w1496, y=w1498) -> (x .and. y?=w1499:bool)
                        n500 = case shown="True" w1499 {
                          tunnel: w1500 -> [_ w1505]
                          tunnel: w1497 -> [_ w1501]
                          frame False {
                          }
                          frame True {
                            n501 = Build Path(base path=w1501, name or relative path="VerticalProjection.txt") -> (appended path=w1503:path)
                            n502 = Build Array(w1505) -> (w1504:i32[][])
                            n503 = call-poly <vilib>:"Write To Spreadsheet File.vi"("transpose? (no:F)"=FALSE, "append to file? (new file:F)"=TRUE, "2D data"=w1504, "file path (dialog if empty)"=w1503) -> ()  [unwired: 4 in, 1 out]
                          }
                        }
                      }
                    }
                    n504 = Array Max & Min(array=w1455) -> (max value=w1471:i32)  [unwired: 3 out]
                    n505 = Greater?(x=w1471, y=w1451) -> (0:w1489:bool)
                    n506 = Array Size(array=w1455) -> (size(s)=w1464:i32)
                    n507 = case "neuen Maximalwert bestimmen" shown="True" w1489 {
                      tunnel: w1451 -> [w1544 w1547]
                      tunnel: w1471 -> [_ w1549]
                      tunnel: [w1544 w1549] -> w1454
                      tunnel: w1449 -> [w1543 w1550]
                      tunnel: [w1543 w1545] -> w1473
                      frame False {
                      }
                      frame True {
                        n508 = Divide(x=w1550, y=w1549) -> (x/y=w1548:dbl[][])
                        n509 = Multiply(x=w1548, y=w1547) -> (x*y=w1546:dbl[][])
                        n510 = To Long Integer(number=w1546) -> (32bit integer=w1545:i32[][])
                      }
                    }
                    n511 = for {
                      N: w1463 -> [w1512]
                      tunnel: w1455 -> [w1514]
                      tunnel: w1464 -> [w1508]
                      tunnel: [w1511] -> w1462 mode=indexing
                      i -> [w1510]
                      n512 = Multiply(x=w1508, y=w1510) -> (x*y=w1509:i32)
                      n513 = Divide(x=w1509, y=w1512) -> (x/y=w1513:dbl)
                      n514 = Interpolate 1D Array(1:w1513, 2:w1514) -> (0:w1511:dbl)
                    }
                    n515 = Divide(x=w1462, y=w1454) -> (x/y=w1490:dbl[])
                    n516 = Array Size(array=w1473) -> (size(s)=w1481:i32[])
                    n517 = Multiply(x=w1491, y=w1490) -> (x*y=w1472:dbl[])
                    n518 = Index Array(array=w1481, index=1) -> (element=w1479:i32)
                    n519 = Insert Into Array(array=w1473, index (col)=w1479, new element=w1472) -> (w1465:i32[][])  [unwired: 1 in]
                    n520 = Array Size(array=w1465) -> (size(s)=w1488:i32[])
                    n521 = Index Array(array=w1488, index=1) -> (element=w1484:i32)
                    n522 = Subtract(x=w1458, y=w1484) -> (x-y=w1485:i32)
                    n523 = Less Than 0?(x=w1485) -> (x < 0?=w1486:bool)
                    n524 = case "wenn voll, alte\nWerte loeschen" shown="True" w1486 {
                      tunnel: w1465 -> [w1537 w1542]
                      tunnel: [w1537 w1541] -> w1495
                      tunnel: w1485 -> [_ w1538]
                      frame False {
                      }
                      frame True {
                        n525 = Absolute Value(x=w1538) -> (abs(x)=w1539:i32)
                        n526 = Delete From Array(array=w1542, length=w1539, index (col)=0 ("index (row)")) -> (array with subset deleted=w1541:i32[][])  [unwired: 1 in, 1 out]
                      }
                    }
                    n527 = Quotient & Remainder(x=w1458, y=w1484) -> (floor(x/y)=w1483:i32)  [unwired: 1 out]
                    n528 = Array Size(array=w1495) -> (size(s)=w1478:i32[])
                    n529 = case shown="Default" w1483 {
                      selector: w1483 -> [_ w1523]
                      tunnel: [1 w1523] -> w1482
                      frame 0 {
                      }
                      frame Default {
                      }
                    }
                    n530 = Index Array(array=w1478, index=1) -> (element=w1476:i32)
                    n531 = for {
                      N: w1476 -> [_]
                      tunnel: w1495 -> [w1530]
                      tunnel: w1482 -> [w1532]
                      shift-right: [w1531] -> w1466
                      shift-left: w1475 -> [w1528]
                      tunnel: w1475 -> [w1524]
                      i -> [w1529]
                      n532 = Index Array(array=w1530, index (col)=w1529) -> (element=w1527:i32[])  [unwired: 1 in]
                      n533 = for {
                        N: w1532 -> [_]
                        shift-right: [w1533] -> w1526
                        shift-left: w1524 -> [w1536]
                        tunnel: w1527 -> [w1535]
                        n534 = Insert Into Array(array=w1536, index (col)=0 ("disabled index (col)"), new element=w1535) -> (w1533:i32[][])  [unwired: 1 in]
                      }
                      n535 = Insert Into Array(array=w1528, index (col)=0 ("disabled index (col)"), new element=w1526) -> (w1531:i32[][])  [unwired: 1 in]
                    }
                    n536 = Array Size(array=w1466) -> (size(s)=w1470:i32[])
                    n537 = Index Array(array=w1470) -> (element #1=w1468:i32, element #2=w1469:i32)  [unwired: 2 in]
                    n538 = Subtract(x=w1458, y=w1469) -> (x-y=w1459:i32)
                    n539 = for "#Pixel to add to fill plot" {
                      N: w1459 -> [_]
                      tunnel: w1468 -> [w1518]
                      shift-right: [w1520] -> w1467
                      shift-left: w1466 -> [w1521]
                      shift-right: [w1516] -> _
                      shift-left: w1469 -> [w1515]
                      n540 = Initialize Array(0.0 ("element"), w1518) -> (w1517:dbl[])
                      n541 = Increment(x=w1515) -> (x+1=w1516:i32)
                      n542 = Insert Into Array(array=w1521, index (col)=w1515, new element=w1517) -> (w1520:i32[][])  [unwired: 1 in]
                    }
                    n543 = Divide(x=w1459, y=w1458) -> (x/y=w1460:dbl)
                    n544 = Subtract(x=1, y=w1460) -> (x-y=w1457:dbl)
                    n545 = Reciprocal(x=w1457) -> (1/x=w1456:dbl)
                  }
                }
              }
              frame #4 {
                n546 = case shown="True" w1568 {
                  tunnel: [w1577 w1604] -> w1575
                  tunnel: [w1578 w1599] -> w1574
                  tunnel: w1573 -> [_ w1595]
                  tunnel: w1572 -> [_ w1589]
                  tunnel: [_ w1587] -> w1562
                  tunnel: [w1576 w1579] -> w1571
                  tunnel: w1570 -> [_ w1585]
                  tunnel: w1569 -> [w1576 w1584]
                  tunnel: w1567 -> [_ w1583]
                  tunnel: w1566 -> [_ w1582]
                  tunnel: w1565 -> [_ w1581]
                  tunnel: w1564 -> [w1577 w1580]
                  tunnel: w1563 -> [w1578 _]
                  frame False {
                  }
                  frame True {
                    # "Plot fraction needed\nfor data"
                    # "hier wird ausgabe\nhorizontal gestaucht"
                    # "das hier\n speichern"
                    # "neues Scanbild"
                    # "Horizontal HeatPlot"
                    n547 = Array Size(array=w1582) -> (size(s)=w1620:i32[])
                    n548 = Index Array(array=w1620, index #1=0 ("index")) -> (element #1=w1606:i32, element #2=w1607:i32)  [unwired: 1 in]
                    n549 = for {
                      N: w1607 -> [_]
                      tunnel: w1582 -> [w1672]
                      tunnel: [w1670] -> w1586 mode=indexing
                      tunnel: w1606 -> [w1669]
                      i -> [w1668]
                      n550 = for {
                        N: w1669 -> [_]
                        tunnel: w1672 -> [w1678]
                        tunnel: w1668 -> [w1673]
                        shift-right: [w1675] -> w1670
                        shift-left: 0 -> [w1676]
                        i -> [w1674]
                        n551 = Index Array(array=w1678, index (row)=w1674, index (col)=w1673) -> (element=w1677:u8)
                        n552 = Add(x=w1676, y=w1677) -> (x+y=w1675:i32)
                      }
                    }
                    n553 = case shown="True" w1585 {
                      tunnel: w1586 -> [_ w1625]
                      tunnel: w1581 -> [_ w1623]
                      tunnel: w1583 -> [_ w1622]
                      frame False {
                      }
                      frame True {
                        n554 = local read "auto save"() -> (w1621:bool)
                        n555 = And(x=w1621, y=w1622) -> (x .and. y?=w1624:bool)
                        n556 = case shown="True" w1624 {
                          tunnel: w1625 -> [_ w1627]
                          tunnel: w1623 -> [_ w1626]
                          frame False {
                          }
                          frame True {
                            n557 = Build Path(base path=w1626, name or relative path="HorizontalProjection.txt") -> (appended path=w1629:path)
                            n558 = Build Array(w1627) -> (w1630:i32[][])
                            n559 = call-poly <vilib>:"Write To Spreadsheet File.vi"("transpose? (no:F)"=FALSE, "append to file? (new file:F)"=TRUE, "2D data"=w1630, "file path (dialog if empty)"=w1629) -> ()  [unwired: 4 in, 1 out]
                          }
                        }
                      }
                    }
                    n560 = Array Max & Min(array=w1586) -> (max value=w1603:i32)  [unwired: 3 out]
                    n561 = Greater?(x=w1603, y=w1584) -> (0:w1615:bool)
                    n562 = Array Size(array=w1586) -> (size(s)=w1594:i32)
                    n563 = case "neuen Maximalwert bestimmen" shown="True" w1615 {
                      tunnel: w1584 -> [w1661 w1664]
                      tunnel: w1603 -> [_ w1666]
                      tunnel: [w1661 w1666] -> w1579
                      tunnel: w1580 -> [w1660 w1667]
                      tunnel: [w1660 w1662] -> w1608
                      frame False {
                      }
                      frame True {
                        n564 = Divide(x=w1667, y=w1666) -> (x/y=w1665:dbl[][])
                        n565 = Multiply(x=w1665, y=w1664) -> (x*y=w1663:dbl[][])
                        n566 = To Long Integer(number=w1663) -> (32bit integer=w1662:i32[][])
                      }
                    }
                    n567 = for {
                      N: w1595 -> [w1637]
                      tunnel: w1586 -> [w1639]
                      tunnel: w1594 -> [w1633]
                      tunnel: [w1636] -> w1593 mode=indexing
                      i -> [w1635]
                      n568 = Multiply(x=w1633, y=w1635) -> (x*y=w1634:i32)
                      n569 = Divide(x=w1634, y=w1637) -> (x/y=w1638:dbl)
                      n570 = Interpolate 1D Array(1:w1638, 2:w1639) -> (0:w1636:dbl)
                    }
                    n571 = Divide(x=w1593, y=w1579) -> (x/y=w1616:dbl[])
                    n572 = Multiply(x=255, y=w1616) -> (x*y=w1618:dbl[])
                    n573 = Insert Into Array(array=w1608, new element=w1618) -> (w1596:i32[][])  [unwired: 2 in]
                    n574 = Array Size(array=w1596) -> (size(s)=w1614:i32[])
                    n575 = Index Array(array=w1614, index=0) -> (element=w1610:i32)
                    n576 = Subtract(x=w1589, y=w1610) -> (x-y=w1611:i32)
                    n577 = Less Than 0?(x=w1611) -> (x < 0?=w1612:bool)
                    n578 = case "wenn voll, alte\n Werte loeschen" shown="True" w1612 {
                      tunnel: w1596 -> [w1654 w1659]
                      tunnel: [w1654 w1658] -> w1604
                      tunnel: w1611 -> [_ w1657]
                      frame False {
                      }
                      frame True {
                        n579 = Absolute Value(x=w1657) -> (abs(x)=w1656:i32)
                        n580 = Delete From Array(array=w1659, length=w1656, index (row)=0) -> (array with subset deleted=w1658:i32[][])  [unwired: 1 in, 1 out]
                      }
                    }
                    n581 = Quotient & Remainder(x=w1589, y=w1610) -> (floor(x/y)=w1609:i32)  [unwired: 1 out]
                    n582 = case shown="Default" w1609 {
                      selector: w1609 -> [_ w1653]
                      tunnel: [1 w1653] -> w1597
                      frame 0 {
                      }
                      frame Default {
                      }
                    }
                    n583 = for {
                      tunnel: w1604 -> [w1649] mode=indexing
                      tunnel: w1597 -> [w1650]
                      shift-right: [w1648] -> w1598
                      shift-left: i32[][] [] ("Analysis Data") -> [w1646]
                      n584 = for {
                        N: w1650 -> [_]
                        tunnel: w1649 -> [w1651]
                        tunnel: [w1651] -> w1647 mode=indexing
                      }
                      n585 = Insert Into Array(array=w1646, new element=w1647) -> (w1648:i32[][])  [unwired: 2 in]
                    }
                    n586 = Array Size(array=w1598) -> (size(s)=w1602:i32[])
                    n587 = Index Array(array=w1602) -> (element #1=w1601:i32, element #2=w1600:i32)  [unwired: 2 in]
                    n588 = Subtract(x=w1589, y=w1601) -> (x-y=w1590:i32)
                    n589 = for {
                      N: w1590 -> [_]
                      tunnel: w1600 -> [w1642]
                      shift-right: [w1644] -> w1599
                      shift-left: w1598 -> [w1645]
                      n590 = Initialize Array(0.0 ("element"), w1642) -> (w1641:dbl[])
                      n591 = Insert Into Array(array=w1645, index (row)=0, new element=w1641) -> (w1644:i32[][])  [unwired: 1 in]
                    }
                    n592 = Divide(x=w1590, y=w1589) -> (x/y=w1591:dbl)
                    n593 = Subtract(x=1, y=w1591) -> (x-y=w1588:dbl)
                    n594 = Reciprocal(x=w1588) -> (1/x=w1587:dbl)
                  }
                }
              }
              frame #5 {
                n595 = case shown="True" w1681 {
                  tunnel: w1697 -> [_ w1718]
                  tunnel: [w1699 w1716] -> w1696
                  tunnel: w1695 -> [_ w1715]
                  tunnel: w1694 -> [_ w1703]
                  tunnel: w1693 -> [w1699 w1714]
                  tunnel: w1692 -> [_ w1713]
                  tunnel: w1691 -> [w1698 w1712]
                  tunnel: [w1698 w1711] -> w1690
                  tunnel: w1689 -> [_ w1710]
                  tunnel: w1688 -> [_ w1709]
                  tunnel: w1687 -> [_ w1708]
                  tunnel: w1686 -> [_ w1702]
                  tunnel: w1685 -> [_ w1707]
                  tunnel: w1684 -> [_ w1706]
                  tunnel: w1683 -> [_ w1705]
                  tunnel: w1682 -> [_ w1704]
                  tunnel: w1680 -> [_ w1701]
                  tunnel: w1679 -> [_ w1700]
                  frame False {
                  }
                  frame True {
                    n596 = case shown="\"Horizontal Projection\", Default" w1718 {
                      tunnel: w1715 -> [w1741 _]
                      tunnel: [w1741 w1778] -> w1717
                      tunnel: w1703 -> [_ w1778]
                      tunnel: w1704 -> [_ w1773]
                      tunnel: w1705 -> [w1736 _]
                      tunnel: w1713 -> [w1740 w1777]
                      tunnel: w1707 -> [w1731 w1769]
                      tunnel: w1712 -> [w1730 w1767]
                      tunnel: [w1729 w1766] -> w1711
                      tunnel: w1710 -> [_ w1765]
                      tunnel: w1709 -> [w1728 _]
                      tunnel: w1708 -> [w1727 _]
                      tunnel: w1702 -> [_ w1764]
                      tunnel: w1701 -> [w1720 w1757]
                      tunnel: w1700 -> [w1719 w1756]
                      frame "Vertical Projection" {
                        n597 = case shown="True" w1731 {
                          tunnel: [w1743 w1755] -> w1732
                          tunnel: w1730 -> [w1748 _]
                          tunnel: ["Measurement Number" ("X Scale.Name Label.Text") w1751] -> w1722
                          tunnel: [w1744 w1754] -> w1721
                          tunnel: [w1743 _] -> w1729
                          tunnel: w1728 -> [w1742 _]
                          tunnel: w1720 -> [_ w1753]
                          tunnel: w1719 -> [_ w1752]
                          frame False {
                            n598 = Increment(x=w1748) -> (x+1=w1743:i32)
                            n599 = Greater?(x=w1743, y=w1742) -> (0:w1747:bool)
                            n600 = Subtract(x=w1743, y=w1742) -> (x-y=w1746:i32)
                            n601 = Select(t=w1746, s=w1747, f=0) -> (s? t:f=w1744:i32)
                          }
                          frame True {
                            w1750 = 0
                            n602 = local read "ScanMin"() -> (w1754:dbl)
                            n603 = Index Array(array=w1753, index=w1750) -> (element=w1755:dbl)
                            n604 = Index Array(array=w1752, index=w1750) -> (element=w1751:string)
                          }
                        }
                        n605 = call "IMAQController.get i attribute.vi"("i ref in"=w1740) -> ("i attribute"=w1739:T17)  [unwired: 16 in, 2 out]
                        n606 = Unbundle By Name(w1739) -> ("activeCamera.Center Coordinates.Vertical"=w1733:i32, "activeCamera.PixelPermm.Vertical"=w1735:dbl)
                        n607 = Subtract(x=w1736, y=w1733) -> (x-y=w1738:i32)
                        n608 = Reciprocal(x=w1735) -> (1/x=w1734:dbl)
                        n609 = Negate(x=w1733) -> (-x=w1737:i32)
                        n610 = Multiply(x=w1738, y=w1734) -> (x*y=w1726:dbl)
                        n611 = Multiply(x=w1734, y=w1737) -> (x*y=w1725:dbl)
                        n612 = Multiply(x=w1727, y=w1732) -> (x*y=w1723:dbl)
                        n613 = property on="HilfsplotProj" class="XYGraph (strict)"("YScale.Maximum"=w1726, "YScale.Minimum"=w1725, "YScale.NameLbl.Text"="vertical position / mm" ("X Scale.Name Label.Text"), "XScale.Maximum"=w1723, "XScale.Minimum"=w1721, "XScale.NameLbl.Text"=w1722) -> ()  [unwired: 2 in, 2 out]
                      }
                      frame "Horizontal Projection", Default {
                        n614 = call "IMAQController.get i attribute.vi"("i ref in"=w1777) -> ("i attribute"=w1776:T17)  [unwired: 16 in, 2 out]
                        n615 = Unbundle By Name(w1776) -> ("activeCamera.Center Coordinates.Horizontal"=w1770:i32, "activeCamera.PixelPermm.Horizontal"=w1772:dbl)
                        n616 = case shown="False" w1769 {
                          tunnel: [w1781 w1792] -> w1768
                          tunnel: w1767 -> [w1785 _]
                          tunnel: ["Measurement Number" ("X Scale.Name Label.Text") w1789] -> w1758
                          tunnel: [w1784 w1791] -> w1759
                          tunnel: [w1781 _] -> w1766
                          tunnel: w1765 -> [w1780 _]
                          tunnel: w1757 -> [_ w1790]
                          tunnel: w1756 -> [_ w1787]
                          frame False {
                            n617 = Increment(x=w1785) -> (x+1=w1781:i32)
                            n618 = Greater?(x=w1781, y=w1780) -> (0:w1783:bool)
                            n619 = Subtract(x=w1781, y=w1780) -> (x-y=w1782:i32)
                            n620 = Select(t=w1782, s=w1783, f=0) -> (s? t:f=w1784:i32)
                          }
                          frame True {
                            w1788 = 0
                            n621 = local read "ScanMin"() -> (w1791:dbl)
                            n622 = Index Array(array=w1787, index=w1788) -> (element=w1789:string)
                            n623 = Index Array(array=w1790, index=w1788) -> (element=w1792:dbl)
                          }
                        }
                        n624 = Subtract(x=w1773, y=w1770) -> (x-y=w1775:i32)
                        n625 = Reciprocal(x=w1772) -> (1/x=w1771:dbl)
                        n626 = Negate(x=w1770) -> (-x=w1774:i32)
                        n627 = Multiply(x=w1775, y=w1771) -> (x*y=w1763:dbl)
                        n628 = Multiply(x=w1771, y=w1774) -> (x*y=w1762:dbl)
                        n629 = Multiply(x=w1768, y=w1764) -> (x*y=w1760:dbl)
                        n630 = property on="HilfsplotProj" class="XYGraph (strict)"("XScale.Maximum"=w1763, "XScale.Minimum"=w1762, "XScale.NameLbl.Text"="horizontal position / mm" ("X Scale.Name Label.Text"), "YScale.Maximum"=w1760, "YScale.Minimum"=w1759, "YScale.NameLbl.Text"=w1758) -> ()  [unwired: 2 in, 2 out]
                      }
                    }
                    n631 = case shown="True" w1706 {
                      tunnel: [w1793 w1796] -> w1716
                      tunnel: w1714 -> [w1793 w1798]
                      tunnel: w1717 -> [_ w1797]
                      frame False {
                      }
                      frame True {
                        n632 = call "IMAQ ArrayToImage"("Image Pixels (U8)"=w1797, "Image"=w1798) -> ("Image Out"=w1796:T3)  [unwired: 8 in, 1 out]
                        n633 = local read "Scan Image"() -> (w1794:i32)
                        n634 = Increment(x=w1794) -> (x+1=→"Scan Image":i32)
                        n635 = local write "ScanImage"(w1796) -> ()
                      }
                    }
                  }
                }
              }
              frame #6 {
                n636 = case shown="True" w1805 {
                  tunnel: w1813 -> [_ w1831]
                  tunnel: w1812 -> [_ w1830]
                  tunnel: w1811 -> [_ w1829]
                  tunnel: w1810 -> [w1817 w1828]
                  tunnel: w1809 -> [w1816 w1827]
                  tunnel: [w1817 w1826] -> w1801
                  tunnel: [w1816 w1825] -> w1800
                  tunnel: w1808 -> [_ w1824]
                  tunnel: w1807 -> [_ w1823]
                  tunnel: w1806 -> [_ w1822]
                  tunnel: w1804 -> [w1815 w1821]
                  tunnel: [w1815 w1820] -> w1799
                  tunnel: w1803 -> [w1814 w1819]
                  tunnel: [w1814 w1818] -> w1802
                  frame False {
                  }
                  frame True {
                    n637 = case shown="True" w1830 {
                      tunnel: w1828 -> [w1835 w1845]
                      tunnel: w1827 -> [w1834 w1848]
                      tunnel: [w1835 w1847] -> w1826
                      tunnel: [w1834 w1846] -> w1825
                      tunnel: w1829 -> [_ w1844]
                      tunnel: w1831 -> [_ w1843]
                      tunnel: w1824 -> [_ w1842]
                      tunnel: w1823 -> [_ w1841]
                      tunnel: w1822 -> [_ w1840]
                      tunnel: w1821 -> [w1833 w1839]
                      tunnel: [w1833 w1838] -> w1820
                      tunnel: w1819 -> [w1832 w1837]
                      tunnel: [w1832 w1836] -> w1818
                      frame False {
                      }
                      frame True {
                        n638 = case shown="True" w1843 {
                          tunnel: w1848 -> [w1851 w1863]
                          tunnel: [w1852 w1860] -> w1847
                          tunnel: [w1851 w1855] -> w1846
                          tunnel: w1844 -> [_ w1865]
                          tunnel: w1845 -> [w1852 w1859]
                          tunnel: w1842 -> [_ w1870]
                          tunnel: w1841 -> [_ w1854]
                          tunnel: w1840 -> [_ w1869]
                          tunnel: w1839 -> [w1850 w1862]
                          tunnel: [w1850 w1861] -> w1838
                          tunnel: w1837 -> [w1849 w1857]
                          tunnel: [w1849 w1856] -> w1836
                          frame False {
                            # "Up to now: Ohne scan auch kein Intensity Plot"
                          }
                          frame True {
                            # "ScanArrays updaten"
                            n639 = Decrement(x=w1854) -> (x-1=w1853:i16)
                            n640 = Index Array(array=w1869, index=w1853) -> (element=w1868:string)
                            n641 = Index Array(array=w1870, index #1=0) -> (element #1=w1856:dbl, element #2=w1866:dbl)  [unwired: 1 in]
                            n642 = property on="Intensity Scan" class="XYGraph (strict)"("XScale.NameLbl.Text"=w1868) -> ()  [unwired: 2 in, 2 out]
                            n643 = Array Size(array=w1859) -> (size(s)=w1858:i32)
                            n644 = Equal To 0?(x=w1858) -> (x = 0?=w1867:bool)
                            n645 = Less?(x=w1856, y=w1857) -> (x < y?=w1864:bool)
                            n646 = case "Init X,Y,Z-Arrays?" shown="False" w1867 {
                              tunnel: w1856 -> [w1873 w1934]
                              tunnel: w1866 -> [w1872 w1933]
                              tunnel: [w1879 w1932] -> w1855
                              tunnel: [w1874 w1931] -> w1860
                              tunnel: w1865 -> [w1877 w1930]
                              tunnel: [w1875 w1928] -> w1861
                              tunnel: w1864 -> [w1881 _]
                              tunnel: w1859 -> [w1880 _]
                              tunnel: w1863 -> [w1878 _]
                              tunnel: w1862 -> [w1876 _]
                              frame False {
                                n647 = case "New y-Value?" shown="True" w1881 {
                                tunnel: w1880 -> [w1885 w1923]
                                tunnel: [w1884 w1921] -> w1879
                                tunnel: w1878 -> [w1886 w1922]
                                tunnel: w1877 -> [w1890 w1917]
                                tunnel: w1876 -> [w1892 w1925]
                                tunnel: [w1895 w1918] -> w1875
                                tunnel: [w1883 w1923] -> w1874
                                tunnel: w1873 -> [w1882 _]
                                tunnel: w1872 -> [_ w1920]
                                frame False {
                                n648 = Array Size(array=w1886) -> (size(s)=w1894:i32)
                                n649 = Decrement(x=w1894) -> (x-1=w1889:i32)
                                n650 = Index Array(array=w1892, index (row)=w1889) -> (element=w1891:dbl[])  [unwired: 1 in]
                                n651 = Search 1D Array(1D array=w1891, element=nan) -> (index of element=w1888:i32)  [unwired: 1 in]
                                n652 = Less Than 0?(x=w1888) -> (x < 0?=w1887:bool)
                                n653 = case "New x-Value?" shown="False" w1887 {
                                tunnel: [w1902 w1909] -> w1895
                                tunnel: w1892 -> [w1901 w1904]
                                tunnel: w1890 -> [w1900 w1908]
                                tunnel: w1889 -> [w1899 _]
                                tunnel: w1888 -> [w1898 _]
                                tunnel: w1886 -> [w1897 w1913]
                                tunnel: w1885 -> [w1896 w1912]
                                tunnel: [w1897 w1913] -> w1884
                                tunnel: [w1896 w1911] -> w1883
                                tunnel: w1882 -> [_ w1910]
                                frame False {
                                n654 = Replace Array Subset(array=w1901, new element=w1900, index (row)=w1899, index (col)=w1898) -> (w1902:dbl[][])
                                }
                                frame True {
                                n655 = Array Size(array=w1904) -> (size(s)=w1905:i32[])
                                n656 = Index Array(array=w1905, index=1) -> (element=w1903:i32)
                                n657 = Build Array(w1908) -> (w1907:dbl[])
                                n658 = Build Array (concatenate)(w1912, w1910) -> (w1911:dbl[])
                                n659 = Insert Into Array(array=w1904, index (col)=w1903, new element=w1907) -> (w1909:dbl[][])  [unwired: 1 in]
                                }
                                }
                                }
                                frame True {
                                n660 = Build Array (concatenate)(w1922, w1920) -> (w1921:dbl[])
                                n661 = Array Size(array=w1925) -> (size(s)=w1927:i32[])
                                n662 = Index Array(array=w1927) -> (element #1=w1914:i32, element #2=w1915:i32)  [unwired: 2 in]
                                n663 = Initialize Array(nan ("element"), w1915) -> (w1924:dbl[])
                                n664 = Build Array (concatenate)(w1925, w1924) -> (w1919:dbl[][])
                                n665 = Replace Array Subset(array=w1919, new element=w1917, index (row)=w1914, index (col)=0 ("disabled index (col)")) -> (w1918:dbl[][])
                                }
                                }
                              }
                              frame True {
                                n666 = Build Array(w1930) -> (w1929:dbl[])
                                n667 = Build Array(w1934) -> (w1931:dbl[])
                                n668 = Build Array(w1933) -> (w1932:dbl[])
                                n669 = Build Array(w1929) -> (w1928:dbl[][])
                              }
                            }
                          }
                        }
                      }
                    }
                  }
                }
              }
              frame #7 {
                n670 = And(x=w1941, y=w1939) -> (x .and. y?=w1940:bool)
                n671 = case shown="True" w1940 {
                  tunnel: w1944 -> [_ w1951]
                  tunnel: w1943 -> [_ w1950]
                  tunnel: w1942 -> [_ w1949]
                  tunnel: w1938 -> [_ w1948]
                  tunnel: w1937 -> [_ w1947]
                  tunnel: w1936 -> [_ w1946]
                  tunnel: w1935 -> [_ w1945]
                  frame False {
                  }
                  frame True {
                    n672 = case shown="True" w1948 {
                      tunnel: w1951 -> [_ w1961]
                      tunnel: w1950 -> [_ w1962]
                      tunnel: w1949 -> [_ w1963]
                      tunnel: w1947 -> [_ w1967]
                      tunnel: w1946 -> [_ w1960]
                      tunnel: w1945 -> [_ w1955]
                      frame False {
                      }
                      frame True {
                        # "File muss in jedem\nSchritt überschrieben \nwerden"
                        # "1D-Intensity Plot"
                        n673 = Subtract(x=w1955, y=2 ("index")) -> (x-y=w1953:i32)
                        n674 = Index Array(array=w1960, index #1=w1953) -> (element #1=w1957:string, element #2=w1956:string)  [unwired: 1 in]
                        n675 = Concatenate Strings(w1956, "vs " ("string"), w1957) -> (w1959:string)
                        n676 = case shown="False" "Show all data" {
                          tunnel: [w1975 w1999] -> w1969
                          tunnel: w1961 -> [w1976 w1998]
                          tunnel: w1963 -> [w1977 w1997]
                          tunnel: "# shown Plots:" -> [w1972 _]
                          tunnel: w1962 -> [w1974 w1996]
                          frame False {
                            n677 = Array Size(array=w1974) -> (size(s)=w1973:i32)
                            n678 = Max & Min(x=w1972, y=w1973) -> (min(x,y)=w1971:i32)  [unwired: 1 out]
                            n679 = for {
                              N: w1971 -> [w1979]
                              tunnel: [w1994] -> w1975 mode=indexing
                              tunnel: w1976 -> [w1993]
                              tunnel: w1977 -> [w1992]
                              tunnel: w1973 -> [w1990]
                              i -> [w1978]
                              w1982 = 1 ("y")
                              n680 = Decrement(x=w1990) -> (x-1=w1981:i32)
                              n681 = Equal?(x=w1979, y=w1982) -> (x = y?=w1985:bool)
                              n682 = Decrement(x=w1979) -> (x-1=w1983:i32)
                              n683 = Select(t=w1982, s=w1985, f=w1983) -> (s? t:f=w1984:i32)
                              n684 = Divide(x=w1978, y=w1984) -> (x/y=w1988:dbl)
                              n685 = Subtract(x=w1981, y=w1978) -> (x-y=w1986:i32)
                              n686 = Multiply(x=w1988, y=200.0 ("x")) -> (x*y=w1980:dbl)
                              n687 = call <vilib>:"RGB to Color.vi"("B"=w1980, "G"=w1980, "R"=w1980) -> ("Color"=w1987:u32)
                              n688 = Index Array(array=w1992, index (row)=w1986) -> (element=w1991:dbl[])  [unwired: 1 in]
                              n689 = property on="Intensity Scan" class="XYGraph (strict)"("Active Plot"=w1978, "Plot.Plot Color"=w1987) -> ()  [unwired: 2 in, 2 out]
                              n690 = Bundle("ScanGraphX"=w1993, "ScanGraphZ"=w1991) -> (w1994:cluster{"ScanGraphX":dbl[], "ScanGraphZ":dbl[]})  [unwired: 1 in]
                            }
                          }
                          frame True {
                            n691 = Array Size(array=w1996) -> (size(s)=w1995:i32)
                            n692 = for {
                              N: w1995 -> [_]
                              tunnel: [w2005] -> w1999 mode=indexing
                              tunnel: w1998 -> [w2004]
                              tunnel: w1997 -> [w2003]
                              i -> [w2001]
                              n693 = Index Array(array=w2003, index (row)=w2001) -> (element=w2002:dbl[])  [unwired: 1 in]
                              n694 = property on="Intensity Scan" class="XYGraph (strict)"("Active Plot"=w2001, "Plot.Plot Color"=u32 0) -> ()  [unwired: 2 in, 2 out]
                              n695 = Bundle("ScanGraphX"=w2004, "ScanGraphZ"=w2002) -> (w2005:cluster{"ScanGraphX":dbl[], "ScanGraphZ":dbl[]})  [unwired: 1 in]
                            }
                          }
                        }
                        "Intensity Scan" <- w1969
                        n696 = Build Path(base path=w1967, name or relative path="Intensity.txt" ("string")) -> (appended path=w1964:path)
                        n697 = call "IMAQController.Write To Spreadsheet File (DBL).vi"("file path (dialog if empty)"=w1964, "Column Header"=w1962, "2D data"=w1963, "General Header"=w1959, "Row Header"=w1961, "append to file? (new file:F)"=FALSE, "transpose? (no:F)"=TRUE) -> ()  [unwired: 12 in, 1 out]
                      }
                    }
                  }
                }
              }
              frame #8 {
                n698 = case shown="True" w2013 {
                  tunnel: w2012 -> [_ w2018]
                  tunnel: w2011 -> [_ w2020]
                  tunnel: w2010 -> [_ w2019]
                  tunnel: w2009 -> [_ w2017]
                  tunnel: w2008 -> [_ w2016]
                  tunnel: w2007 -> [_ w2015]
                  tunnel: w2006 -> [_ w2014]
                  frame False {
                  }
                  frame True {
                    n699 = Greater?(x=w2018, y=i16 1) -> (0:w2022:bool)
                    n700 = case shown="True" w2022 {
                      tunnel: w2020 -> [_ w2029]
                      tunnel: w2019 -> [_ w2028]
                      tunnel: w2018 -> [_ w2027]
                      tunnel: w2017 -> [_ w2026]
                      tunnel: w2016 -> [_ w2025]
                      tunnel: w2015 -> [_ w2024]
                      tunnel: w2014 -> [_ w2023]
                      frame False {
                      }
                      frame True {
                        n701 = case shown="True" w2028 {
                          tunnel: w2029 -> [_ w2039]
                          tunnel: w2027 -> [_ w2038]
                          tunnel: w2026 -> [_ w2035]
                          tunnel: w2025 -> [_ w2036]
                          tunnel: w2024 -> [_ w2037]
                          tunnel: w2023 -> [_ w2030]
                          frame False {
                          }
                          frame True {
                            n702 = Array Size(array=w2035) -> (size(s)=w2034:i32[])
                            n703 = Index Array(array=w2034) -> (element=w2033:i32)  [unwired: 1 in]
                            n704 = Greater?(x=w2033, y=1 ("index")) -> (0:w2031:bool)
                            n705 = case "enough data available" shown="True" w2031 {
                              tunnel: w2039 -> [_ w2049]
                              tunnel: w2038 -> [_ w2048]
                              tunnel: w2035 -> [_ w2047]
                              tunnel: w2037 -> [_ w2046]
                              tunnel: w2036 -> [_ w2045]
                              tunnel: w2030 -> [_ w2040]
                              frame False {
                              }
                              frame True {
                                w2041 = u16 7 ("Axis:Name Label:Name Label Size")
                                w2042 = TRUE ("Axis:Range:Range Auto Scale")
                                n706 = Subtract(x=w2048, y=2 ("index")) -> (x-y=w2050:i32)
                                n707 = Index Array(array=w2049, index #1=w2050) -> (element #1=w2044:string, element #2=w2043:string)  [unwired: 1 in]
                                n708 = property on="3D Surface" class="3D Surface (strict)"("Axis:Active Axis"=enum16{"X-axis", "Y-axis", "Z-axis"}."X-axis", "Axis:Name Label Text"=w2044, "Axis:Range Auto Scale"=w2042, "Axis:Name Label Size"=w2041) -> (error out=w2057:errorcluster)  [unwired: 2 in, 1 out]
                                n709 = call-poly <vilib>:"Plot Helper.vi"("z matrix"=w2047, "y vector"=w2046, "x vector"=w2045, "3D Plot lvclass Array in"=w2040) -> ("3D Plot lvclass Array out"=→"3D Surface":refnum<class "3D Plot Datatype.lvclass">[])  [unwired: 2 in, 5 out]
                                n710 = property on="3D Surface" class="3D Surface (strict)"(error in=w2057, "Axis:Active Axis"=enum16{"X-axis", "Y-axis", "Z-axis"}."Y-axis", "Axis:Name Label Text"=w2043, "Axis:Range Auto Scale"=w2042, "Axis:Name Label Size"=w2041) -> (error out=w2054:errorcluster)  [unwired: 1 in, 1 out]
                                n711 = property on="3D Surface" class="3D Surface (strict)"(error in=w2054, "Axis:Active Axis"=enum16{"X-axis", "Y-axis", "Z-axis"}."Z-axis", "Axis:Name Label Text"="ROI 2 / ROI 1" ("Axis:Name Label:Name Label Text"), "Axis:Range Auto Scale"=w2042, "Axis:Name Label Size"=w2041) -> ()  [unwired: 1 in, 2 out]
                              }
                            }
                          }
                        }
                      }
                    }
                  }
                }
              }
              frame #9 {
                n712 = case shown="True" w2065 {
                  tunnel: w2064 -> [_ w2072]
                  tunnel: w2063 -> [_ w2071]
                  tunnel: w2062 -> [_ w2070]
                  tunnel: w2061 -> [_ w2069]
                  tunnel: w2059 -> [_ w2066]
                  tunnel: w2060 -> [_ w2068]
                  frame False {
                  }
                  frame True {
                    w2073 = T8 {"Data"=[], "Height"=0, "Width"=0, "Save path out Horizontal"=path "", "Save path out Vertical"=path ""}  # Analysis Step 3
                    n713 = Bundle By Name(cluster=w2073, "Data"=w2072, "Height"=w2071, "Width"=w2070, "Save path out Horizontal"=w2069, "Save path out Vertical"=w2066) -> (w2074:T8)
                    n714 = Generate User Event(user event=w2068, event data cluster=w2074) -> ()  [unwired: 2 in, 2 out]
                    n715 = Strip Path(path=w2066) -> (name=→"AnaStep2":string)  [unwired: 1 out]
                  }
                }
              }
            }
          }
          event User Event {
            n716 = event-data() -> ("CameraChange?"=w2106:bool)  [unwired: 1 in]
            n717 = case shown="True" w2106 {
              tunnel: w2105 -> [w2121 _]
              tunnel: [w2121 _] -> w2104
              tunnel: w2103 -> [w2120 _]
              tunnel: [w2120 _] -> w2102
              tunnel: w2101 -> [w2119 _]
              tunnel: w2100 -> [w2118 _]
              tunnel: [w2119 _] -> w2099
              tunnel: [w2118 _] -> w2098
              tunnel: w2097 -> [w2117 w2137]
              tunnel: [w2117 w2137] -> w2096
              tunnel: w2095 -> [w2116 _]
              tunnel: w2094 -> [w2115 _]
              tunnel: [w2116 _] -> w2093
              tunnel: [w2115 _] -> w2092
              tunnel: w2091 -> [w2114 _]
              tunnel: w2090 -> [w2113 _]
              tunnel: [w2114 _] -> w2089
              tunnel: [w2113 _] -> w2088
              tunnel: w2087 -> [w2112 _]
              tunnel: w2086 -> [w2111 _]
              tunnel: w2085 -> [w2110 _]
              tunnel: [w2112 _] -> w2084
              tunnel: [w2111 _] -> w2083
              tunnel: [w2110 _] -> w2082
              tunnel: w2081 -> [w2109 _]
              tunnel: w2080 -> [w2108 _]
              tunnel: [w2109 _] -> w2079
              tunnel: [w2108 _] -> w2078
              tunnel: w2077 -> [w2107 w2126]
              tunnel: [w2107 w2126] -> w2076
              tunnel: w2075 -> [_ w2122]
              frame False {
              }
              frame True {
                w2125 = sgl[] [] ("y vector")
                n718 = call-poly <vilib>:"Plot Helper.vi"("z matrix"=sgl[][] [], "y vector"=w2125, "x vector"=w2125, "3D Plot lvclass Array in"=w2122) -> ("3D Plot lvclass Array out"=w2123:refnum<class "3D Plot Datatype.lvclass">[])  [unwired: 2 in, 5 out]
                n719 = property on="3D Surface" class="3D Surface (strict)"("Axis:Active Axis"=enum16{"X-axis", "Y-axis", "Z-axis"}."X-axis", "Axis:Name Label Text"="X Axis" ("Axis:Name Label:Name Label Text")) -> (error out=w2134:errorcluster)  [unwired: 2 in, 1 out]
                n720 = local write "3D Surface"(w2123) -> ()
                n721 = local write "Intensity Scan"(cluster{dbl[], dbl[]}[] [] ("Intensity Scan")) -> ()
                n722 = property on="3D Surface" class="3D Surface (strict)"(error in=w2134, "Axis:Active Axis"=enum16{"X-axis", "Y-axis", "Z-axis"}."Y-axis", "Axis:Name Label Text"="Y Axis" ("Axis:Name Label:Name Label Text")) -> ()  [unwired: 1 in, 2 out]
                n723 = local write "ROI 1 / ROI 2"(0.0 ("ROI 1 / ROI 2")) -> ()
                n724 = property on="Intensity Scan" class="XYGraph (strict)"("XScale.NameLbl.Text"="Scanname" ("X Scale.Name Label.Text")) -> ()  [unwired: 2 in, 2 out]
                n725 = call "IMAQ ArrayToImage"("Image Pixels (U8)"=u8[][] [], "Image"=w2126) -> ("Image Out"=w2128:T3)  [unwired: 8 in, 1 out]
                n726 = local write "ScanImage"(w2128) -> ()
              }
            }
          }
          event User Event {
            n727 = event-data() -> ("NewScan?"=w2162:bool)  [unwired: 1 in]
            n728 = case shown="False" w2162 {
              tunnel: w2161 -> [w2175 _]
              tunnel: w2160 -> [w2174 _]
              tunnel: w2159 -> [w2176 _]
              tunnel: [w2176 w2177] -> w2158
              tunnel: [w2175 _] -> w2157
              tunnel: [w2174 _] -> w2156
              tunnel: w2155 -> [w2173 _]
              tunnel: [w2173 _] -> w2154
              tunnel: w2153 -> [w2172 _]
              tunnel: [w2172 w2177] -> w2152
              tunnel: w2151 -> [w2171 _]
              tunnel: [w2171 _] -> w2150
              tunnel: w2149 -> [w2170 _]
              tunnel: w2147 -> [w2169 _]
              tunnel: [w2170 _] -> w2148
              tunnel: [w2169 _] -> w2146
              tunnel: w2145 -> [w2168 _]
              tunnel: w2144 -> [w2167 _]
              tunnel: [w2168 _] -> w2143
              tunnel: [w2167 _] -> w2142
              tunnel: [w2166 _] -> w2141
              tunnel: w2140 -> [w2166 _]
              tunnel: [w2165 _] -> w2139
              tunnel: w2138 -> [w2165 _]
              frame False {
              }
              frame True {
                w2177 = i32[][] []  # Analysis Data
                n729 = local write "Progress bar"(u8 0 ("Progress bar")) -> ()
              }
            }
          }
          event User Event {
            w2189 = T21."Disabled and Grayed Out" ("Disabled")
            w2190 = T21."Enabled" ("Disabled")
            n730 = event-data() -> ()  [unwired: 1 in, 4 out]
            n731 = property on="Configure Scan button" class="Bool"("DisabledEnum"=w2190) -> ()  [unwired: 2 in, 2 out]
            n732 = property on="Start Scan button" class="Bool"("DisabledEnum"=w2190) -> ()  [unwired: 2 in, 2 out]
            n733 = property on="Pause Scan button" class="Bool"("DisabledEnum"=w2189) -> ()  [unwired: 2 in, 2 out]
            n734 = property on="Stop Scan button" class="Bool"("DisabledEnum"=w2189) -> ()  [unwired: 2 in, 2 out]
            n735 = local write "ScanRunning?"(FALSE ("ScanRunning?")) -> ()
          }
        }
      }
      frame Error {
        n736 = event shown="[1] <Stop>: User Event" {
          selector: w2213 -> [_ _ _]
          dyn-events: _ -> [_ _ _]
          timeout: w2211 -> [_ _ _]
          tunnel: [_ TRUE _] -> w2212
          tunnel: w2210 -> [w2214 w2215 w2219]
          tunnel: [w2214 w2215 w2217] -> w2209
          event Timeout {
            n737 = event-data() -> ()  [unwired: 1 in, 2 out]
          }
          event User Event {
            n738 = event-data() -> ()  [unwired: 1 in, 4 out]
          }
          event "Error OR": Mouse Down {
            n739 = event-data() -> ()  [unwired: 1 in, 7 out]
            n740 = call <vilib>:"Clear Errors.vi"("error in (no error)"=w2219) -> ("error out"=w2218:errorcluster)  [unwired: 5 in, 1 out]
            n741 = invoke on="Error OR" class="Bool (strict)" method="Reinit To Default"(error in=w2218) -> (error out=w2217:errorcluster)  [unwired: 2 in, 2 out]
          }
        }
      }
    }
    n742 = local write "Analysis Event error out"(w979) -> ()
    "Analysis Event Loop" <- w988
  }
  n743 = while "Send Command Loop" {
    tunnel: w79 -> [w2229]
    shift-right: [w2220] -> w143
    shift-left: w96 -> [w2223]
    tunnel: w78 -> [w2225]
    tunnel: w132 -> [w2222]
    i -> [w2228]
    stop <- w2226 continue-if-true
    n744 = case shown="No Error" w2223 {
      selector: w2223 -> [w2234 w2254]
      tunnel: w2229 -> [w2236 _]
      tunnel: [w2235 w2253] -> w2220
      tunnel: w2222 -> [_ w2252]
      tunnel: [w2233 T2."free Running" ("Acquisition mode")] -> w2221
      frame No Error {
        n745 = local read "Acquisition mode (Buffer)"() -> (w2233:T2)
        n746 = local read "Camera\nConnected?"() -> (w2232:bool)
        n747 = case shown="True" w2232 {
          tunnel: w2236 -> [_ w2241]
          tunnel: [w2237 w2240] -> w2235
          tunnel: w2234 -> [w2237 w2239]
          tunnel: w2233 -> [_ w2238]
          frame False {
          }
          frame True {
            n748 = case shown="\"Internal Trigger\", \"External Trigger\"" w2238 {
              tunnel: w2241 -> [w2246 _]
              tunnel: w2239 -> [w2245 w2250]
              tunnel: [w2248 w2250] -> w2240
              frame "Internal Trigger", "External Trigger" {
                n749 = call "IMAQController.get i attribute.vi"("i ref in"=w2246, "error in (no error)"=w2245) -> ("i ref out"=w2247:refnum<vi>, "i attribute"=w2243:T17, "error out"=w2244:errorcluster)  [unwired: 15 in]
                n750 = Unbundle By Name(w2243) -> ("actCamera"=w2242:string)
                n751 = call "BaseProcess.call process 2.vi"("i ref in"=w2247, "Object"=w2242, "Selector"="snap_and_publish", "error in (no error)"=w2244) -> ("error out"=w2248:errorcluster)  [unwired: 14 in, 1 out]
              }
              frame Default {
              }
            }
          }
        }
      }
      frame Error {
        n752 = Wait on Notification(notifier=w2252, timeout in ms (-1)=500) -> (notification=w2257:i32, timed out?=w2256:bool)  [unwired: 2 in, 2 out]
        n753 = case shown="False" w2256 {
          tunnel: w2254 -> [w2259 w2264]
          tunnel: [w2258 w2264] -> w2253
          tunnel: w2257 -> [w2260 _]
          frame False {
            n754 = case shown="1" w2260 {
              tunnel: w2259 -> [w2262 w2263]
              tunnel: [w2261 w2263] -> w2258
              frame 1 {
                n755 = call <vilib>:"Clear Errors.vi"("error in (no error)"=w2262) -> ("error out"=w2261:errorcluster)  [unwired: 5 in, 1 out]
              }
              frame Default {
              }
            }
          }
          frame True {
          }
        }
      }
    }
    n756 = case shown="Default" w2221 {
      tunnel: [w2230 10 ("Acquisition delay (ms)")] -> w2224
      frame Default {
        n757 = local read "Delay (ms) Buffered"() -> (w2230:i32)
      }
      frame "free Running" {
      }
    }
    n758 = local write "Send command error out"(w2220) -> ()
    n759 = Wait on Occurrence(1:FALSE ("ignore previous (T)"), 2:w2225, 3:w2224) -> (0:w2226:bool)
    "Send Command Loop" <- w2228
  }
  n760 = while "Scan Pixel Value Loop" {
    tunnel: w145 -> [w2281]
    shift-right: [w2277] -> w123
    shift-left: w144 -> [w2280]
    shift-right: [w2276] -> _
    shift-left: w127 -> [w2275]
    tunnel: w69 -> [w2272]
    tunnel: [w2272] -> w121
    shift-right: [w2273] -> _
    shift-left: w120 -> [w2274]
    shift-right: [w2269] -> _
    shift-left: w118 -> [w2271]
    shift-right: [w2268] -> _
    shift-left: w119 -> [w2270]
    tunnel: w79 -> [w2267]
    tunnel: w94 -> [w2266]
    tunnel: [w2266] -> w93
    tunnel: w42 -> [w2265]
    i -> [w2282]
    stop <- w2278 stop-if-true
    # "der hier gibt fast staendig\nfehlermeldungen aus,\ndeshalb schickt er nichts\nan den logger!!"
    n761 = event shown="[7] <Analysis Step 1>: User Event" {
      selector: w2281 -> [_ _ _ _ _ _ _ _ _ _ _ _ _ _]
      dyn-events: _ -> [_ _ _ _ _ _ _ _ _ _ _ _ _ _]
      timeout: -1 -> [_ _ _ _ _ _ _ _ _ _ _ _ _ _]
      tunnel: w2280 -> [w2287 w2306 w2320 w2347 w2352 w2378 _ w2630 w2733 w2753 w2816 w2881 w2912 w2917]
      tunnel: [_ _ _ _ _ _ _ _ _ _ _ _ _ TRUE] -> w2278
      tunnel: [w2287 w2293 w2319 w2347 w2352 w2377 w2515 w2631 w2751 w2777 w2840 w2880 w2912 w2917] -> w2277
      tunnel: [w2286 w2291 w2316 w2346 w2351 w2362 w2519 w2613 w2750 w2760 w2823 w2882 w2911 w2916] -> w2276
      tunnel: w2275 -> [w2286 w2291 w2314 w2346 w2351 w2376 w2570 w2614 _ w2760 w2823 w2882 w2911 w2916]
      tunnel: w2272 -> [_ _ _ _ _ w2375 w2529 w2629 w2736 _ _ _ _ _]
      tunnel: w2274 -> [w2285 w2290 w2318 w2345 w2350 w2374 w2569 w2627 _ w2759 w2822 w2885 w2910 w2915]
      tunnel: [w2285 w2290 w2318 w2345 w2350 w2373 w2518 w2627 w2750 w2759 w2822 w2885 w2910 w2915] -> w2273
      tunnel: w2271 -> [w2284 w2289 w2313 w2343 w2349 w2363 w2568 w2626 _ w2758 w2821 w2884 w2909 w2914]
      tunnel: w2270 -> [w2283 w2288 w2312 w2342 w2348 w2365 w2567 w2625 _ w2757 w2820 w2883 w2908 w2913]
      tunnel: [w2284 w2289 w2315 w2343 w2349 w2361 w2517 w2626 w2750 w2758 w2821 w2884 w2909 w2914] -> w2269
      tunnel: [w2283 w2288 w2312 w2342 w2348 w2364 w2516 w2625 w2750 w2757 w2820 w2883 w2908 w2913] -> w2268
      tunnel: w2267 -> [_ _ _ _ _ w2360 _ _ w2734 w2754 w2817 w2878 _ _]
      tunnel: w2266 -> [_ _ _ _ _ w2359 w2530 w2618 _ _ _ _ _ _]
      tunnel: w2265 -> [_ _ _ _ _ w2358 w2520 w2628 _ _ _ _ _ _]
      event Timeout {
        n762 = event-data() -> ()  [unwired: 1 in, 2 out]
      }
      event "ScanImage": Mouse Move {
        w2297 = " , " ("string")
        # "At the beginning no image is\navailable, which would result\nin an error here"
        n763 = event-data() -> ()  [unwired: 1 in, 4 out]
        n764 = property on="ScanImage"(error in=w2306) -> (error out=w2301:errorcluster, "Last Mouse Position"=w2305)  [unwired: 1 in, 1 out]
        n765 = local read "ScanImage"() -> (w2292:T3)
        n766 = Unbundle(w2305) -> (w2300, w2299)
        n767 = call "IMAQ GetPixelValue"("Image"=w2292, "X Coordinate"=w2300, "Y Coordinate"=w2299, "error in (no error)"=w2301) -> ("Pixel Value (U8)"=w2298:u8, "error out"=w2294:errorcluster)  [unwired: 2 in, 3 out]
        n768 = Unbundle(w2294) -> ("code"=w2295:i32)  [unwired: 2 out]
        n769 = case shown="-1074396120" w2295 {
          tunnel: w2294 -> [_ w2308]
          tunnel: [errorcluster {"status"=FALSE, "code"=0, "source"=""} ("error out") w2308] -> w2293
          frame -1074396120 {
          }
          frame Default {
          }
        }
        n770 = Number To Decimal String(number=w2300) -> (decimal integer string=w2304:string)  [unwired: 1 in]
        n771 = Number To Decimal String(number=w2299) -> (decimal integer string=w2303:string)  [unwired: 1 in]
        n772 = Number To Decimal String(number=w2298) -> (decimal integer string=w2296:string)  [unwired: 1 in]
        n773 = Concatenate Strings(w2304, w2297, w2303, w2297, w2296) -> (→"Scan Image\nInformation":string)
      }
      event "ActImage": Mouse Down {
        n774 = event-data() -> ("Button"=w2317:u16)  [unwired: 1 in, 6 out]
        n775 = case shown="2" w2317 {
          tunnel: [TRUE _ TRUE] -> w2311
          frame 0, Default {
          }
          frame 1 {
            w2339 = TRUE ("ActImage Mouse Down?")
            n776 = local write "ActImage LMouse Down?"(w2339) -> ()
            n777 = local write "ActImage LSelectionOn?"(w2339) -> ()
          }
          frame 2 {
            w2341 = TRUE ("ActImage Mouse Down?")
            n778 = local write "ActImage RMouse Down?"(w2341) -> ()
            n779 = local write "ActImage RSelectionOn?"(w2341) -> ()
          }
        }
        n780 = local read "ROI2notROI1Boolen"() -> (w2309:bool)
        n781 = And(x=w2309, y=w2311) -> (x .and. y?=w2310:bool)
        n782 = case shown="False" w2310 {
          tunnel: w2320 -> [w2328 w2336]
          tunnel: [w2327 w2336] -> w2319
          tunnel: w2317 -> [w2326 _]
          tunnel: [w2324 w2337] -> w2316
          tunnel: [w2323 w2335] -> w2315
          tunnel: w2314 -> [w2322 w2337]
          tunnel: w2313 -> [w2321 w2335]
          frame False {
            n783 = property on="ActImage"(error in=w2328) -> (error out=w2327:errorcluster, "Last Mouse Position"=w2325)  [unwired: 1 in, 1 out]
            n784 = case shown="2" w2326 {
              tunnel: w2325 -> [_ w2332 w2334]
              tunnel: [w2330 w2332 w2333] -> w2324
              tunnel: [w2329 w2331 w2334] -> w2323
              tunnel: w2322 -> [w2330 _ w2333]
              tunnel: w2321 -> [w2329 w2331 _]
              frame 0, Default {
              }
              frame 1 {
              }
              frame 2 {
              }
            }
          }
          frame True {
          }
        }
      }
      event "ActImage": Mouse Leave {
        w2344 = FALSE ("ActImage Mouse Down?")
        n785 = event-data() -> ()  [unwired: 1 in, 3 out]
        n786 = local write "ActImage RMouse Down?"(w2344) -> ()
        n787 = local write "ActImage LMouse Down?"(w2344) -> ()
      }
      event "ActImage": Mouse Up {
        n788 = event-data() -> ("Button"=w2353:u16)  [unwired: 1 in, 6 out]
        n789 = case shown="1" w2353 {
          frame 0, Default {
          }
          frame 1 {
            n790 = local write "ActImage LMouse Down?"(FALSE ("ActImage Mouse Down?")) -> ()
          }
          frame 2 {
            n791 = local write "ActImage RMouse Down?"(FALSE ("ActImage Mouse Down?")) -> ()
          }
        }
      }
      event "ActImage": Mouse Move {
        n792 = event-data() -> ()  [unwired: 1 in, 4 out]
        n793 = local read "ActImage LMouse Down?"() -> (w2372:bool)
        n794 = local read "ActImage RMouse Down?"() -> (w2367:bool)
        n795 = local read "ActImage LSelectionOn?"() -> (w2371:bool)
        n796 = local read "ActImage RSelectionOn?"() -> (w2366:bool)
        n797 = local read "ROI2notROI1Boolen"() -> (w2357:bool)
        n798 = Not(x=w2357) -> (.not. x?=w2356:bool)
        n799 = And(x=w2372, y=w2371) -> (x .and. y?=w2370:bool)
        n800 = Compound Arithmetic op=AND(w2367, w2366, w2356) -> (w2368:bool)
        n801 = Or(x=w2370, y=w2368) -> (x .or. y?=w2369:bool)
        n802 = stacked-sequence {
          seq-local: [w2387 _] -> [_ w2489]
          tunnel: w2378 -> [w2393 _]
          tunnel: [_ w2490] -> w2377
          tunnel: w2376 -> [w2392 _]
          tunnel: w2375 -> [w2391 _]
          tunnel: w2374 -> [w2390 _]
          tunnel: [w2389 _] -> w2373
          tunnel: w2369 -> [w2388 _]
          tunnel: w2363 -> [w2386 _]
          tunnel: w2365 -> [w2385 _]
          tunnel: [w2384 _] -> w2364
          tunnel: w2358 -> [w2383 _]
          tunnel: [w2382 _] -> w2362
          tunnel: [w2381 _] -> w2361
          tunnel: w2360 -> [w2380 _]
          tunnel: w2359 -> [w2379 _]
          frame #0 {
            n803 = case shown="True" w2388 {
              tunnel: w2393 -> [w2397 w2419]
              tunnel: [w2397 w2426] -> w2387
              tunnel: w2392 -> [w2395 w2416]
              tunnel: w2391 -> [_ w2406]
              tunnel: w2390 -> [w2398 w2433]
              tunnel: [w2398 w2415] -> w2389
              tunnel: w2386 -> [w2394 w2414]
              tunnel: w2385 -> [w2396 w2428]
              tunnel: [w2396 w2413] -> w2384
              tunnel: w2383 -> [_ w2425]
              tunnel: [w2395 w2416] -> w2382
              tunnel: [w2394 w2414] -> w2381
              tunnel: w2380 -> [_ w2417]
              tunnel: w2379 -> [_ w2405]
              frame False {
              }
              frame True {
                w2400 = T10 {"Data"=[], "Height"=0, "Width"=0, "Save path out Scan"=path "", "Save path out Horizontal"=path "", "Save path out Vertical"=path "", "Scan?"=TRUE, "Scan running?"=TRUE, "ROI Calculation?"=TRUE, "Starting Mouse Position 1"={"X"=0, "Y"=0}, "End Mouse Position 1"={"X"=0, "Y"=0}, "Starting Mouse Position 2"={"X"=0, "Y"=0}, "End Mouse Position 2"={"X"=0, "Y"=0}, "do analysis?"=TRUE, "ScanValuesArray"=[], "ActDimensions"=0, "ScanNamesArray"=[], "Av repeat?"=FALSE}  # Analysis Step 2
                w2408 = 0 ("Height")
                w2409 = FALSE ("Scan?")
                w2410 = path "" ("Save path out Scan")
                w2438 = sgl 255.0 ("Pixel Color")
                w2442 = 0 ("element")
                w2441 = u16 0 items=["Line", "Rectangle", "Oval"] ("Shape to draw")
                n804 = call "IMAQController.get i attribute.vi"("i ref in"=w2417, "error in (no error)"=w2419) -> ("i attribute"=w2422:T17, "error out"=w2418:errorcluster)  [unwired: 15 in, 1 out]
                n805 = Unbundle By Name(w2422) -> ("activeCamera.Center Coordinates.Horizontal"=w2421:i32, "activeCamera.Center Coordinates.Vertical"=w2420:i32)
                n806 = local read "Image height"() -> (w2444:i32)
                n807 = local read "Image length"() -> (w2445:i32)
                n808 = Build Array(w2421, w2442, w2421, w2444) -> (w2439:i32[])
                n809 = call "IMAQ Draw"("Shape to draw"=w2441, "Pixel Color"=w2438, "error in (no error)"=w2418, "Coordinates"=w2439, "Image Dst"=w2405, "Image Src"=w2406) -> ("error out"=w2440:errorcluster, "Image Dst Out"=w2423:T3)  [unwired: 4 in]
                n810 = Build Array(w2442, w2420, w2445, w2420) -> (w2443:i32[])
                n811 = local read "ActImage LMouse Down?"() -> (w2434:bool)
                n812 = call "IMAQ Draw"("Shape to draw"=w2441, "Pixel Color"=w2438, "error in (no error)"=w2440, "Coordinates"=w2443, "Image Src"=w2423) -> ("error out"=w2437:errorcluster, "Image Dst Out"=w2435:T3)  [unwired: 5 in]
                n813 = local read "ActImage LSelectionOn?"() -> (w2436:bool)
                n814 = property on="ActImage"(error in=w2437) -> (error out=w2446:errorcluster, "Last Mouse Position"=w2430)  [unwired: 1 in, 1 out]
                n815 = case shown="True" w2436 {
                  tunnel: w2446 -> [w2469 w2486]
                  tunnel: w2416 -> [_ w2485]
                  tunnel: w2430 -> [_ w2481]
                  tunnel: [w2469 w2472] -> w2432
                  tunnel: w2435 -> [w2470 w2483]
                  tunnel: [w2470 w2471] -> w2431
                  tunnel: w2434 -> [_ w2482]
                  tunnel: w2433 -> [w2468 w2480]
                  tunnel: [w2468 w2477] -> w2415
                  frame False {
                  }
                  frame True {
                    w2478 = u16 1 items=["Line", "Rectangle", "Oval"] ("Shape to draw")
                    n816 = Unbundle By Name(w2485) -> ("X"=w2476:i32, "Y"=w2475:i32)
                    n817 = case shown="True" w2482 {
                      tunnel: w2481 -> [_ w2488]
                      tunnel: w2480 -> [w2487 _]
                      tunnel: [w2487 w2488] -> w2477
                      frame False {
                      }
                      frame True {
                      }
                    }
                    n818 = Unbundle By Name(w2477) -> ("X"=w2474:i32, "Y"=w2473:i32)
                    n819 = Build Array(w2476, w2475, w2474, w2473) -> (w2484:i32[])
                    n820 = call "IMAQ Draw"("Shape to draw"=w2478, "Pixel Color"=sgl 255.0, "error in (no error)"=w2486, "Coordinates"=w2484, "Image Src"=w2483) -> ("error out"=w2472:errorcluster, "Image Dst Out"=w2471:T3)  [unwired: 5 in]
                  }
                }
                n821 = local read "ActImage RMouse Down?"() -> (w2429:bool)
                n822 = local read "ActImage RSelectionOn?"() -> (w2401:bool)
                n823 = case shown="True" w2401 {
                  tunnel: w2432 -> [w2449 w2465]
                  tunnel: w2414 -> [_ w2464]
                  tunnel: w2430 -> [_ w2460]
                  tunnel: [w2449 w2450] -> w2427
                  tunnel: w2431 -> [w2447 w2462]
                  tunnel: w2429 -> [_ w2461]
                  tunnel: w2428 -> [w2448 w2459]
                  tunnel: [w2448 w2456] -> w2413
                  tunnel: [w2447 w2451] -> w2424
                  frame False {
                  }
                  frame True {
                    w2457 = u16 1 items=["Line", "Rectangle", "Oval"] ("Shape to draw")
                    n824 = Unbundle By Name(w2464) -> ("X"=w2455:i32, "Y"=w2454:i32)
                    n825 = case shown="True" w2461 {
                      tunnel: w2460 -> [_ w2467]
                      tunnel: w2459 -> [w2466 _]
                      tunnel: [w2466 w2467] -> w2456
                      frame False {
                      }
                      frame True {
                      }
                    }
                    n826 = Unbundle By Name(w2456) -> ("X"=w2453:i32, "Y"=w2452:i32)
                    n827 = Build Array(w2455, w2454, w2453, w2452) -> (w2463:i32[])
                    n828 = call "IMAQ Draw"("Shape to draw"=w2457, "Pixel Color"=sgl 255.0, "error in (no error)"=w2465, "Coordinates"=w2463, "Image Src"=w2462) -> ("error out"=w2450:errorcluster, "Image Dst Out"=w2451:T3)  [unwired: 5 in]
                  }
                }
                n829 = local write "ActImage"(w2424) -> ()
                n830 = Bundle(cluster=w2400, "Data"=u8[][] [], "Height"=w2408, "Width"=w2408, "Save path out Scan"=w2410, "Save path out Horizontal"=w2410, "Save path out Vertical"=w2410, "Scan?"=w2409, "Scan running?"=w2409, "ROI Calculation?"=w2409, "Starting Mouse Position 1"=w2416, "End Mouse Position 1"=w2415, "Starting Mouse Position 2"=w2414, "End Mouse Position 2"=w2413, "do analysis?"=FALSE, "ScanValuesArray"=dbl[] [], "ActDimensions"=i16 0, "ScanNamesArray"=string[] [], "Av repeat?"=FALSE) -> (w2411:T10)
                n831 = Generate User Event(user event=w2425, event data cluster=w2411, error in=w2427) -> (error out=w2426:errorcluster)  [unwired: 1 in, 1 out]
              }
            }
          }
          frame #1 {
            w2496 = " , " ("string")
            # "At the beginning no image is\navailable, which would result\nin an error here"
            n832 = property on="ActImage"(error in=w2489) -> (error out=w2500:errorcluster, "Last Mouse Position"=w2503)  [unwired: 1 in, 1 out]
            n833 = local read "ActImage"() -> (w2491:T3)
            n834 = Unbundle(w2503) -> (w2499, w2498)
            n835 = call "IMAQ GetPixelValue"("Image"=w2491, "X Coordinate"=w2499, "Y Coordinate"=w2498, "error in (no error)"=w2500) -> ("Pixel Value (U8)"=w2497:u8, "error out"=w2493:errorcluster)  [unwired: 2 in, 3 out]
            n836 = Unbundle(w2493) -> ("code"=w2494:i32)  [unwired: 2 out]
            n837 = case shown="-1074396120, -1074395317" w2494 {
              tunnel: w2493 -> [_ w2505]
              tunnel: [errorcluster {"status"=FALSE, "code"=0, "source"=""} ("error out") w2505] -> w2490
              frame -1074396120, -1074395317 {
              }
              frame Default {
              }
            }
            n838 = Number To Decimal String(number=w2499) -> (decimal integer string=w2502:string)  [unwired: 1 in]
            n839 = Number To Decimal String(number=w2498) -> (decimal integer string=w2501:string)  [unwired: 1 in]
            n840 = Number To Decimal String(number=w2497) -> (decimal integer string=w2495:string)  [unwired: 1 in]
            n841 = Concatenate Strings(w2502, w2496, w2501, w2496, w2495) -> (→"Act Image\nInformation":string)
          }
        }
      }
      event "TL1x", "TL1y", "BR1x", "BR1y", "TL2x", "TL2y", "BR2x", "BR2y": Value Change {
        w2507 = T10 {"Data"=[], "Height"=0, "Width"=0, "Save path out Scan"=path "", "Save path out Horizontal"=path "", "Save path out Vertical"=path "", "Scan?"=TRUE, "Scan running?"=TRUE, "ROI Calculation?"=TRUE, "Starting Mouse Position 1"={"X"=0, "Y"=0}, "End Mouse Position 1"={"X"=0, "Y"=0}, "Starting Mouse Position 2"={"X"=0, "Y"=0}, "End Mouse Position 2"={"X"=0, "Y"=0}, "do analysis?"=TRUE, "ScanValuesArray"=[], "ActDimensions"=0, "ScanNamesArray"=[], "Av repeat?"=FALSE}  # Analysis Step 2
        w2524 = 0 ("Height")
        w2526 = FALSE ("Scan?")
        w2525 = path "" ("Save path out Scan")
        w2544 = 0
        n842 = event-data() -> ("CtlRef"=w2554:refnum<vi>, "NewVal"=w2555:i32)  [unwired: 1 in]
        n843 = control-ref of="TL1x"() -> (w2552:refnum<vi>)
        n844 = control-ref of="TL1y"() -> (w2551:refnum<vi>)
        n845 = control-ref of="BR1x"() -> (w2550:refnum<vi>)
        n846 = control-ref of="BR1y"() -> (w2549:refnum<vi>)
        n847 = control-ref of="TL2x"() -> (w2548:refnum<vi>)
        n848 = control-ref of="TL2y"() -> (w2547:refnum<vi>)
        n849 = control-ref of="BR2y"() -> (w2546:refnum<vi>)
        n850 = control-ref of="BR2x"() -> (w2545:refnum<vi>)
        n851 = Build Array(w2570, w2569, w2568, w2567) -> (w2563:cluster{"X":i32, "Y":i32}[])
        n852 = Type Cast(type=w2544, x=w2552) -> (*(type *) &x=w2543:i32)
        n853 = Type Cast(type=w2544, x=w2551) -> (*(type *) &x=w2542:i32)
        n854 = Type Cast(type=w2544, x=w2550) -> (*(type *) &x=w2541:i32)
        n855 = Type Cast(type=w2544, x=w2549) -> (*(type *) &x=w2540:i32)
        n856 = Type Cast(type=w2544, x=w2548) -> (*(type *) &x=w2539:i32)
        n857 = Type Cast(type=w2544, x=w2547) -> (*(type *) &x=w2538:i32)
        n858 = Type Cast(type=w2544, x=w2546) -> (*(type *) &x=w2537:i32)
        n859 = Type Cast(type=w2544, x=w2545) -> (*(type *) &x=w2536:i32)
        n860 = Type Cast(type=w2544, x=w2554) -> (*(type *) &x=w2553:i32)
        n861 = Build Array(w2543, w2542, w2541, w2540, w2539, w2538, w2537, w2536) -> (w2571:i32[])
        n862 = Search 1D Array(1D array=w2571, element=w2553) -> (index of element=w2561:i32)  [unwired: 1 in]
        n863 = Quotient & Remainder(x=w2561, y=2) -> (x-y*floor(x/y)=w2559:i32)  [unwired: 1 out]
        n864 = Divide(x=w2561, y=2) -> (x/y=w2565:dbl)
        n865 = Round Toward -Infinity(1:w2565) -> (0:w2562:dbl)
        n866 = Equal To 0?(x=w2559) -> (x = 0?=w2558:bool)
        n867 = Index Array(array=w2563, index=w2562) -> (element=w2557:cluster{"X":i32, "Y":i32})
        n868 = case shown="True" w2558 {
          tunnel: w2557 -> [w2605 w2609]
          tunnel: [w2604 w2608] -> w2556
          tunnel: w2555 -> [w2602 w2607]
          frame True {
            n869 = Unbundle(w2605) -> ("Y"=w2603:i32)  [unwired: 1 out]
            n870 = Bundle(cluster=w2605, "X"=w2602, "Y"=w2603) -> (w2604:cluster{"X":i32, "Y":i32})
          }
          frame False {
            n871 = Unbundle(w2609) -> ("X"=w2606:i32)  [unwired: 1 out]
            n872 = Bundle(cluster=w2609, "X"=w2606, "Y"=w2607) -> (w2608:cluster{"X":i32, "Y":i32})
          }
        }
        n873 = local read "ActImage LSelectionOn?"() -> (w2531:bool)
        n874 = Replace Array Subset(array=w2563, new element=w2556, index=w2562) -> (w2564:cluster{"X":i32, "Y":i32}[])
        n875 = call "IMAQ Copy"("Image Dst"=w2530, "Image Src"=w2529) -> ("error out"=w2532:errorcluster, "Image Dst Out"=w2533:T3)  [unwired: 4 in]
        n876 = Index Array(array=w2564) -> (element #1=w2519:cluster{"X":i32, "Y":i32}, element #2=w2518:cluster{"X":i32, "Y":i32}, element #3=w2517:cluster{"X":i32, "Y":i32}, element #4=w2516:cluster{"X":i32, "Y":i32})  [unwired: 4 in]
        n877 = case shown="True" w2531 {
          tunnel: w2532 -> [w2588 w2601]
          tunnel: [w2588 w2590] -> w2535
          tunnel: w2533 -> [w2587 w2589]
          tunnel: w2519 -> [_ w2599]
          tunnel: w2518 -> [_ w2598]
          tunnel: [w2587 w2591] -> w2534
          frame False {
          }
          frame True {
            w2596 = u16 1 items=["Line", "Rectangle", "Oval"] ("Shape to draw")
            n878 = Unbundle By Name(w2599) -> ("X"=w2595:i32, "Y"=w2594:i32)
            n879 = Unbundle By Name(w2598) -> ("X"=w2593:i32, "Y"=w2592:i32)
            n880 = Build Array(w2595, w2594, w2593, w2592) -> (w2600:i32[])
            n881 = call "IMAQ Draw"("Shape to draw"=w2596, "Pixel Color"=sgl 255.0, "error in (no error)"=w2601, "Coordinates"=w2600, "Image Src"=w2589) -> ("error out"=w2590:errorcluster, "Image Dst Out"=w2591:T3)  [unwired: 5 in]
          }
        }
        n882 = local read "ActImage RSelectionOn?"() -> (w2509:bool)
        n883 = local read "ROI2notROI1Boolen"() -> (w2511:bool)
        n884 = Not(x=w2511) -> (.not. x?=w2508:bool)
        n885 = And(x=w2509, y=w2508) -> (x .and. y?=w2510:bool)
        n886 = case shown="True" w2510 {
          tunnel: w2535 -> [w2573 w2586]
          tunnel: [w2573 w2574] -> w2521
          tunnel: w2534 -> [w2572 w2582]
          tunnel: w2517 -> [_ w2584]
          tunnel: w2516 -> [_ w2583]
          tunnel: [w2572 w2575] -> w2528
          frame False {
          }
          frame True {
            w2580 = u16 1 items=["Line", "Rectangle", "Oval"] ("Shape to draw")
            n887 = Unbundle By Name(w2584) -> ("X"=w2579:i32, "Y"=w2578:i32)
            n888 = Unbundle By Name(w2583) -> ("X"=w2577:i32, "Y"=w2576:i32)
            n889 = Build Array(w2579, w2578, w2577, w2576) -> (w2585:i32[])
            n890 = call "IMAQ Draw"("Shape to draw"=w2580, "Pixel Color"=sgl 255.0, "error in (no error)"=w2586, "Coordinates"=w2585, "Image Src"=w2582) -> ("error out"=w2574:errorcluster, "Image Dst Out"=w2575:T3)  [unwired: 5 in]
          }
        }
        n891 = local write "ActImage"(w2528) -> ()
        n892 = Bundle(cluster=w2507, "Data"=u8[][] [], "Height"=w2524, "Width"=w2524, "Save path out Scan"=w2525, "Save path out Horizontal"=w2525, "Save path out Vertical"=w2525, "Scan?"=w2526, "Scan running?"=w2526, "ROI Calculation?"=w2526, "Starting Mouse Position 1"=w2519, "End Mouse Position 1"=w2518, "Starting Mouse Position 2"=w2517, "End Mouse Position 2"=w2516, "do analysis?"=FALSE, "ScanValuesArray"=dbl[] [], "ActDimensions"=i16 0, "ScanNamesArray"=string[] [], "Av repeat?"=FALSE) -> (w2522:T10)
        n893 = Generate User Event(user event=w2520, event data cluster=w2522, error in=w2521) -> (error out=w2515:errorcluster)  [unwired: 1 in, 1 out]
      }
      event User Event {
        n894 = event-data() -> ("Data"=w2624:u8[][], "Height"=w2611:i32, "Width"=w2623:i32, "Save path out Scan"=w2621:path, "Save path out Horizontal"=w2622:path, "Save path out Vertical"=w2612:path, "Scan?"=w2620:bool, "Scan running?"=w2619:bool, "ScanValuesArray"=w2617:dbl[], "ActDimensions"=w2616:i16, "ScanNamesArray"=w2615:string[], "Av repeat?"=w2610:bool)  [unwired: 1 in]
        n895 = case shown="False" w2610 {
          selector: w2610 -> [_ w2711]
          tunnel: [w2670 w2728] -> w2631
          tunnel: w2630 -> [w2665 w2727]
          tunnel: w2629 -> [w2663 _]
          tunnel: w2628 -> [w2662 w2726]
          tunnel: w2627 -> [w2661 w2717]
          tunnel: w2626 -> [w2660 w2716]
          tunnel: w2625 -> [w2659 w2715]
          tunnel: w2624 -> [w2655 _]
          tunnel: w2611 -> [w2654 _]
          tunnel: w2623 -> [w2653 _]
          tunnel: w2622 -> [w2652 _]
          tunnel: w2621 -> [w2651 _]
          tunnel: w2620 -> [w2650 w2713]
          tunnel: w2619 -> [w2649 _]
          tunnel: w2618 -> [w2646 _]
          tunnel: w2617 -> [w2645 _]
          tunnel: w2616 -> [w2644 _]
          tunnel: w2615 -> [w2643 _]
          tunnel: w2614 -> [w2642 w2718]
          tunnel: [w2641 w2718] -> w2613
          tunnel: w2612 -> [w2640 _]
          frame False {
            w2634 = T10 {"Data"=[], "Height"=0, "Width"=0, "Save path out Scan"=path "", "Save path out Horizontal"=path "", "Save path out Vertical"=path "", "Scan?"=TRUE, "Scan running?"=TRUE, "ROI Calculation?"=TRUE, "Starting Mouse Position 1"={"X"=0, "Y"=0}, "End Mouse Position 1"={"X"=0, "Y"=0}, "Starting Mouse Position 2"={"X"=0, "Y"=0}, "End Mouse Position 2"={"X"=0, "Y"=0}, "do analysis?"=TRUE, "ScanValuesArray"=[], "ActDimensions"=0, "ScanNamesArray"=[], "Av repeat?"=FALSE}  # Analysis Step 2
            n896 = local read "ActImage LSelectionOn?"() -> (w2656:bool)
            n897 = call "IMAQ Copy"("error in (no error)"=w2665, "Image Dst"=w2646, "Image Src"=w2663) -> ("error out"=w2664:errorcluster, "Image Dst Out"=w2647:T3)  [unwired: 3 in]
            n898 = case shown="True" w2656 {
              tunnel: w2664 -> [w2696 w2709]
              tunnel: [w2696 w2698] -> w2669
              tunnel: w2647 -> [w2695 w2697]
              tunnel: w2642 -> [_ w2707]
              tunnel: w2661 -> [_ w2706]
              tunnel: [w2695 w2699] -> w2668
              frame False {
              }
              frame True {
                w2704 = u16 1 items=["Line", "Rectangle", "Oval"] ("Shape to draw")
                n899 = Unbundle By Name(w2707) -> ("X"=w2703:i32, "Y"=w2702:i32)
                n900 = Unbundle By Name(w2706) -> ("X"=w2701:i32, "Y"=w2700:i32)
                n901 = Build Array(w2703, w2702, w2701, w2700) -> (w2708:i32[])
                n902 = call "IMAQ Draw"("Shape to draw"=w2704, "Pixel Color"=sgl 255.0, "error in (no error)"=w2709, "Coordinates"=w2708, "Image Src"=w2697) -> ("error out"=w2698:errorcluster, "Image Dst Out"=w2699:T3)  [unwired: 5 in]
              }
            }
            n903 = local read "ROI2notROI1Boolen"() -> (w2638:bool)
            n904 = local read "ActImage RSelectionOn?"() -> (w2636:bool)
            n905 = Not(x=w2638) -> (.not. x?=w2637:bool)
            n906 = And(x=w2637, y=w2636) -> (x .and. y?=w2635:bool)
            n907 = case shown="True" w2635 {
              tunnel: w2669 -> [w2681 w2694]
              tunnel: [w2681 w2682] -> w2667
              tunnel: w2668 -> [w2680 w2690]
              tunnel: w2660 -> [_ w2692]
              tunnel: w2659 -> [_ w2691]
              tunnel: [w2680 w2683] -> w2632
              frame False {
              }
              frame True {
                w2688 = u16 1 items=["Line", "Rectangle", "Oval"] ("Shape to draw")
                n908 = Unbundle By Name(w2692) -> ("X"=w2687:i32, "Y"=w2686:i32)
                n909 = Unbundle By Name(w2691) -> ("X"=w2685:i32, "Y"=w2684:i32)
                n910 = Build Array(w2687, w2686, w2685, w2684) -> (w2693:i32[])
                n911 = call "IMAQ Draw"("Shape to draw"=w2688, "Pixel Color"=sgl 255.0, "error in (no error)"=w2694, "Coordinates"=w2693, "Image Src"=w2690) -> ("error out"=w2682:errorcluster, "Image Dst Out"=w2683:T3)  [unwired: 5 in]
              }
            }
            n912 = flat-sequence {
              tunnel: w2632 -> [w2672]
              tunnel: w2642 -> [w2671]
              tunnel: [w2671] -> w2641
              frame #0 {
                n913 = local write "ActImage"(w2672) -> ()
              }
            }
            n914 = And(x=w2635, y=w2656) -> (x .and. y?=w2657:bool)
            n915 = Or(x=w2656, y=w2657) -> (x .or. y?=w2658:bool)
            n916 = Bundle(cluster=w2634, "Data"=w2655, "Height"=w2654, "Width"=w2653, "Save path out Scan"=w2651, "Save path out Horizontal"=w2652, "Save path out Vertical"=w2640, "Scan?"=w2650, "Scan running?"=w2649, "ROI Calculation?"=w2658, "Starting Mouse Position 1"=w2641, "End Mouse Position 1"=w2661, "Starting Mouse Position 2"=w2660, "End Mouse Position 2"=w2659, "do analysis?"=TRUE, "ScanValuesArray"=w2645, "ActDimensions"=w2644, "ScanNamesArray"=w2643, "Av repeat?"=FALSE) -> (w2666:T10)
            n917 = Strip Path(path=w2640) -> (name=→"AnaStep1":string)  [unwired: 1 out]
            n918 = case shown="True" w2650 {
              frame False {
              }
              frame True {
                n919 = local read "SNofSteps"() -> (w2677:i32)
                n920 = local read "SActStep"() -> (w2678:i32)
                n921 = Increment(x=w2678) -> (x+1=w2676:i32)
                n922 = Divide(x=w2676, y=w2677) -> (x/y=w2679:dbl)
                n923 = Multiply(x=w2679, y=100.0) -> (x*y=w2674:u8)
                n924 = local write "Progress bar"(w2674) -> ()
                n925 = Number To Decimal String(number=w2674) -> (decimal integer string=w2673:string)  [unwired: 1 in]
                n926 = property on="Progress bar" class="Slide (strict)"("TipStrip"=w2673) -> ()  [unwired: 2 in, 2 out]
              }
            }
            n927 = Generate User Event(user event=w2662, event data cluster=w2666, error in=w2667) -> (error out=w2670:errorcluster)  [unwired: 1 in, 1 out]
          }
          frame True {
            w2712 = T10 {"Data"=[], "Height"=0, "Width"=0, "Save path out Scan"=path "", "Save path out Horizontal"=path "", "Save path out Vertical"=path "", "Scan?"=TRUE, "Scan running?"=TRUE, "ROI Calculation?"=TRUE, "Starting Mouse Position 1"={"X"=0, "Y"=0}, "End Mouse Position 1"={"X"=0, "Y"=0}, "Starting Mouse Position 2"={"X"=0, "Y"=0}, "End Mouse Position 2"={"X"=0, "Y"=0}, "do analysis?"=TRUE, "ScanValuesArray"=[], "ActDimensions"=0, "ScanNamesArray"=[], "Av repeat?"=FALSE}  # Analysis Step 2
            w2714 = FALSE ("Scan?")
            w2722 = path "" ("Save path out Scan")
            w2723 = 0 ("Height")
            n928 = Bundle(cluster=w2712, "Data"=u8[][] [], "Height"=w2723, "Width"=w2723, "Save path out Scan"=w2722, "Save path out Horizontal"=w2722, "Save path out Vertical"=w2722, "Scan?"=w2713, "Scan running?"=w2714, "ROI Calculation?"=w2714, "Starting Mouse Position 1"=w2718, "End Mouse Position 1"=w2717, "Starting Mouse Position 2"=w2716, "End Mouse Position 2"=w2715, "do analysis?"=TRUE, "ScanValuesArray"=dbl[] [], "ActDimensions"=i16 0, "ScanNamesArray"=string[] [], "Av repeat?"=w2711) -> (w2725:T10)
            n929 = Generate User Event(user event=w2726, event data cluster=w2725, error in=w2727) -> (error out=w2728:errorcluster)  [unwired: 1 in, 1 out]
          }
        }
      }
      event "Clear ROIs button": Value Change {
        w2729 = FALSE ("ActImage RSelectionOn?")
        w2742 = sgl 255.0 ("Pixel Color")
        w2744 = 0 ("element")
        w2746 = u16 0 items=["Line", "Rectangle", "Oval"] ("Shape to draw")
        w2749 = 0.0 ("TL1x")
        w2750 = cluster{"X":i32, "Y":i32} {"X"=0, "Y"=0}
        n930 = event-data() -> ()  [unwired: 1 in, 5 out]
        n931 = call "IMAQController.get i attribute.vi"("i ref in"=w2734, "error in (no error)"=w2733) -> ("i attribute"=w2735:T17, "error out"=w2732:errorcluster)  [unwired: 15 in, 1 out]
        n932 = Unbundle By Name(w2735) -> ("activeCamera.Center Coordinates.Horizontal"=w2731:i32, "activeCamera.Center Coordinates.Vertical"=w2730:i32)
        n933 = local read "Image height"() -> (w2738:i32)
        n934 = local read "Image length"() -> (w2737:i32)
        n935 = local read "ActImage"() -> (w2739:T3)
        n936 = Build Array(w2731, w2744, w2731, w2738) -> (w2748:i32[])
        n937 = call "IMAQ Draw"("Shape to draw"=w2746, "Pixel Color"=w2742, "error in (no error)"=w2732, "Coordinates"=w2748, "Image Dst"=w2739, "Image Src"=w2736) -> ("error out"=w2747:errorcluster, "Image Dst Out"=w2743:T3)  [unwired: 4 in]
        n938 = Build Array(w2744, w2730, w2737, w2730) -> (w2745:i32[])
        n939 = call "IMAQ Draw"("Shape to draw"=w2746, "Pixel Color"=w2742, "error in (no error)"=w2747, "Coordinates"=w2745, "Image Src"=w2743) -> ("error out"=w2741:errorcluster, "Image Dst Out"=w2740:T3)  [unwired: 5 in]
        n940 = local write "ActImage"(w2740) -> ()
        n941 = invoke on="Clear ROIs button" class="Bool" method="Reinit To Default"(error in=w2741) -> (error out=w2751:errorcluster)  [unwired: 2 in, 2 out]
        n942 = local write "ActImage RSelectionOn?"(w2729) -> ()
        n943 = local write "ActImage LSelectionOn?"(w2729) -> ()
        n944 = local write "TL1x"(w2749) -> ()
        n945 = local write "TL1y"(w2749) -> ()
        n946 = local write "BR1y"(w2749) -> ()
        n947 = local write "BR1x"(w2749) -> ()
        n948 = local write "TL2x"(w2749) -> ()
        n949 = local write "TL2y"(w2749) -> ()
        n950 = local write "BR2y"(w2749) -> ()
        n951 = local write "BR2x"(w2749) -> ()
        n952 = local write "ROI 1"(w2749) -> ()
        n953 = local write "ROI 2"(w2749) -> ()
        n954 = local write "ROI 1 / ROI 2"(w2749) -> ()
      }
      event "Horizontal chart XY": Mouse Move {
        n955 = event-data() -> ("Coords"=w2776:T18)  [unwired: 1 in, 3 out]
        n956 = call "IMAQController.get i attribute.vi"("i ref in"=w2754, "error in (no error)"=w2753) -> ("i attribute"=w2756:T17, "error out"=w2752:errorcluster)  [unwired: 15 in, 1 out]
        n957 = property on="Horizontal chart XY" class="XYGraph (strict)"(error in=w2752) -> (error out=w2775:errorcluster, "ActXScl"=w2761:i32, "ActYScl"=w2762:i32, "XScale.Minimum"=w2766:dbl, "XScale.Maximum"=w2767:dbl, "YScale.Minimum"=w2764:dbl, "YScale.Maximum"=w2765:dbl)  [unwired: 1 in, 1 out]
        n958 = Unbundle By Name(w2756) -> ("activeCamera.PixelPermm.Horizontal"=w2755:dbl)
        n959 = invoke on="Horizontal chart XY" class="XYGraph (strict)" method="Map Coords To XY"(error in=w2775, "Coords"=w2776, "X Scale"=w2761, "Y Scale"=w2762) -> (error out=w2774:errorcluster, "XY"=w2768:cluster{"X":dbl, "Y":dbl})  [unwired: 3 in, 5 out]
        n960 = Unbundle(w2768) -> ("X"=w2773:dbl, "Y"=w2769:dbl)
        n961 = In Range and Coerce(upper limit=w2767, x=w2773, lower limit=w2766) -> (In Range?=w2771:bool)  [unwired: 1 out]
        n962 = In Range and Coerce(upper limit=w2765, x=w2769, lower limit=w2764) -> (In Range?=w2770:bool)  [unwired: 1 out]
        n963 = And(x=w2771, y=w2770) -> (x .and. y?=w2772:bool)
        n964 = case shown="True" w2772 {
          tunnel: [w2780 w2814] -> w2777
          tunnel: w2769 -> [_ w2804]
          tunnel: w2773 -> [_ w2801]
          tunnel: w2774 -> [w2781 w2800]
          tunnel: w2768 -> [_ w2799]
          tunnel: w2767 -> [_ w2798]
          tunnel: w2766 -> [_ w2797]
          tunnel: w2765 -> [_ w2796]
          tunnel: w2764 -> [_ w2795]
          tunnel: T24 {"Name"="", "Color"=0, "Style"=0, "Point Style"=0, "Name Visible"=FALSE, "Allow Drag"=FALSE, "Annotation Mode"=0, "Plot"=0, "Index"=0, "Position"={"X"=0.0, "Y"=0.0}, "X Scale"=0, "Y Scale"=0, "Show Arrow"=FALSE, "Lock Name"=FALSE, "Plot Area"=0, "Label Offset"={"X"=0.0, "Y"=0.0}} -> [w2778 w2794]
          tunnel: w2755 -> [_ w2786]
          frame False {
            n965 = Build Array(w2778) -> (w2779:T25)
            n966 = property on="Horizontal chart XY" class="XYGraph (strict)"(error in=w2781, "AnntList"=w2779) -> (error out=w2780:errorcluster)  [unwired: 1 in, 1 out]
          }
          frame True {
            w2782 = i16 7 ("width (-)")
            w2785 = 15.0 ("y")
            w2792 = i16 2 ("width (-)")
            n967 = Subtract(x=w2798, y=w2797) -> (x-y=w2788:dbl)
            n968 = Subtract(x=w2796, y=w2795) -> (x-y=w2784:dbl)
            n969 = Number To Fractional String(number=w2801, width (-)=w2782, precision (6)=w2792) -> (F-format string=w2802:string)  [unwired: 1 in]
            n970 = Number To Fractional String(number=w2804, width (-)=w2782, precision (6)=w2792) -> (F-format string=w2803:string)  [unwired: 1 in]
            n971 = Multiply(x=w2788, y=w2786) -> (x*y=w2787:dbl)
            n972 = Divide(x=w2787, y=w2785) -> (x/y=w2790:dbl)
            n973 = Divide(x=w2784, y=w2785) -> (x/y=w2789:dbl)
            n974 = Concatenate Strings(w2802, "\r", w2803) -> (w2783:string)
            n975 = Bundle(w2790, w2789) -> (w2791:cluster{dbl, dbl})  [unwired: 1 in]
            n976 = Bundle By Name(cluster=w2794, "Name"=w2783, "Color"=u32 16711680, "Style"=u8 0, "Point Style"=u8 0, "Name Visible"=TRUE, "Allow Drag"=FALSE, "Annotation Mode"=u32 0, "Position"=w2799, "Show Arrow"=FALSE, "Label Offset"=w2791) -> (w2813:T24)
            n977 = Build Array(w2813) -> (w2812:T25)
            n978 = property on="Horizontal chart XY" class="XYGraph (strict)"(error in=w2800, "AnntList"=w2812) -> (error out=w2814:errorcluster)  [unwired: 1 in, 1 out]
          }
        }
      }
      event "Vertical chart XY": Mouse Move {
        n979 = event-data() -> ("Coords"=w2839:T18)  [unwired: 1 in, 3 out]
        n980 = call "IMAQController.get i attribute.vi"("i ref in"=w2817, "error in (no error)"=w2816) -> ("i attribute"=w2819:T17, "error out"=w2815:errorcluster)  [unwired: 15 in, 1 out]
        n981 = Unbundle By Name(w2819) -> ("activeCamera.PixelPermm.Vertical"=w2818:dbl)
        n982 = property on="Vertical chart XY" class="XYGraph (strict)"(error in=w2815) -> (error out=w2838:errorcluster, "ActXScl"=w2824:i32, "ActYScl"=w2825:i32, "XScale.Minimum"=w2829:dbl, "XScale.Maximum"=w2830:dbl, "YScale.Minimum"=w2827:dbl, "YScale.Maximum"=w2828:dbl)  [unwired: 1 in, 1 out]
        n983 = invoke on="Vertical chart XY" class="XYGraph (strict)" method="Map Coords To XY"(error in=w2838, "Coords"=w2839, "X Scale"=w2824, "Y Scale"=w2825) -> (error out=w2837:errorcluster, "XY"=w2831:cluster{"X":dbl, "Y":dbl})  [unwired: 3 in, 5 out]
        n984 = Unbundle(w2831) -> ("X"=w2836:dbl, "Y"=w2832:dbl)
        n985 = In Range and Coerce(upper limit=w2830, x=w2836, lower limit=w2829) -> (In Range?=w2834:bool)  [unwired: 1 out]
        n986 = In Range and Coerce(upper limit=w2828, x=w2832, lower limit=w2827) -> (In Range?=w2833:bool)  [unwired: 1 out]
        n987 = And(x=w2834, y=w2833) -> (x .and. y?=w2835:bool)
        n988 = case shown="True" w2835 {
          tunnel: [w2843 w2877] -> w2840
          tunnel: w2832 -> [_ w2867]
          tunnel: w2836 -> [_ w2864]
          tunnel: w2837 -> [w2844 w2863]
          tunnel: w2831 -> [_ w2862]
          tunnel: w2830 -> [_ w2861]
          tunnel: w2829 -> [_ w2860]
          tunnel: w2828 -> [_ w2859]
          tunnel: w2827 -> [_ w2858]
          tunnel: T24 {"Name"="", "Color"=0, "Style"=0, "Point Style"=0, "Name Visible"=FALSE, "Allow Drag"=FALSE, "Annotation Mode"=0, "Plot"=0, "Index"=0, "Position"={"X"=0.0, "Y"=0.0}, "X Scale"=0, "Y Scale"=0, "Show Arrow"=FALSE, "Lock Name"=FALSE, "Plot Area"=0, "Label Offset"={"X"=0.0, "Y"=0.0}} -> [w2841 w2857]
          tunnel: w2818 -> [_ w2849]
          frame False {
            n989 = Build Array(w2841) -> (w2842:T25)
            n990 = property on="Vertical chart XY" class="XYGraph (strict)"(error in=w2844, "AnntList"=w2842) -> (error out=w2843:errorcluster)  [unwired: 1 in, 1 out]
          }
          frame True {
            w2845 = i16 6 ("width (-)")
            w2848 = 15.0 ("y")
            w2855 = i16 2 ("width (-)")
            n991 = Subtract(x=w2861, y=w2860) -> (x-y=w2851:dbl)
            n992 = Subtract(x=w2859, y=w2858) -> (x-y=w2847:dbl)
            n993 = Number To Fractional String(number=w2864, width (-)=w2845, precision (6)=w2855) -> (F-format string=w2865:string)  [unwired: 1 in]
            n994 = Number To Fractional String(number=w2867, width (-)=w2845, precision (6)=w2855) -> (F-format string=w2866:string)  [unwired: 1 in]
            n995 = Multiply(x=w2851, y=w2849) -> (x*y=w2850:dbl)
            n996 = Divide(x=w2850, y=w2848) -> (x/y=w2853:dbl)
            n997 = Divide(x=w2847, y=w2848) -> (x/y=w2852:dbl)
            n998 = Concatenate Strings(w2865, "\r", w2866) -> (w2846:string)
            n999 = Bundle(w2853, w2852) -> (w2854:cluster{dbl, dbl})  [unwired: 1 in]
            n1000 = Bundle By Name(cluster=w2857, "Name"=w2846, "Color"=u32 16711680, "Style"=u8 0, "Point Style"=u8 0, "Name Visible"=TRUE, "Allow Drag"=FALSE, "Annotation Mode"=u32 0, "Position"=w2862, "Show Arrow"=FALSE, "Label Offset"=w2854) -> (w2876:T24)
            n1001 = Build Array(w2876) -> (w2875:T25)
            n1002 = property on="Vertical chart XY" class="XYGraph (strict)"(error in=w2863, "AnntList"=w2875) -> (error out=w2877:errorcluster)  [unwired: 1 in, 1 out]
          }
        }
      }
      event "TestButton": Value Change {
        n1003 = event-data() -> ("NewVal"=w2879:bool)  [unwired: 1 in, 4 out]
        n1004 = case shown="True" w2879 {
          tunnel: w2881 -> [w2886 w2899]
          tunnel: [w2886 w2905] -> w2880
          tunnel: w2878 -> [_ w2903]
          frame False {
          }
          frame True {
            n1005 = call-poly "CoreLib.data 2 byte array.vi"("i32"=1) -> ("byteArray out"=w2898:T26)  [unwired: 18 in]
            n1006 = call-poly "CoreLib.data 2 byte array.vi"("byteArray"=w2898, "string"="testNomen") -> ("byteArray out"=w2897:T26)  [unwired: 17 in]
            n1007 = call-poly "CoreLib.data 2 byte array.vi"("byteArray"=w2897, "string"="testProperty") -> ("byteArray out"=w2896:T26)  [unwired: 17 in]
            n1008 = call-poly "CoreLib.data 2 byte array.vi"("byteArray"=w2896, "i32"=1) -> ("byteArray out"=w2895:T26)  [unwired: 17 in]
            n1009 = call-poly "CoreLib.data 2 byte array.vi"("byteArray"=w2895, "string"="string") -> ("byteArray out"=w2894:T26)  [unwired: 17 in]
            n1010 = call-poly "CoreLib.data 2 byte array.vi"("byteArray"=w2894, "i16"=1.0 ("f32")) -> ("byteArray out"=w2893:T26)  [unwired: 17 in]
            n1011 = call "BaseProcess.call process 2.vi"("i ref in"=w2903, "Object"="myAccInterface", "Selector"="Write1Value", "Data Descriptor"="L:1;C:N;C:N;L:1;C:N;S:1", "Data"=w2893, "error in (no error)"=w2899) -> ("error out"=w2904:errorcluster)  [unwired: 12 in, 1 out]
            n1012 = invoke on="TestButton" class="Bool (strict)" method="Reinit To Default"(error in=w2904) -> (error out=w2905:errorcluster)  [unwired: 2 in, 2 out]
          }
        }
      }
      event "Horizontal chart XY", "Vertical chart XY": Mouse Leave {
        n1013 = event-data() -> ()  [unwired: 1 in, 3 out]
        n1014 = Build Array(T24 {"Name"="", "Color"=0, "Style"=0, "Point Style"=0, "Name Visible"=FALSE, "Allow Drag"=FALSE, "Annotation Mode"=0, "Plot"=0, "Index"=0, "Position"={"X"=0.0, "Y"=0.0}, "X Scale"=0, "Y Scale"=0, "Show Arrow"=FALSE, "Lock Name"=FALSE, "Plot Area"=0, "Label Offset"={"X"=0.0, "Y"=0.0}}) -> (w2907:T25)
        n1015 = property on="Horizontal chart XY" class="XYGraph (strict)"("AnntList"=w2907) -> ()  [unwired: 2 in, 2 out]
        n1016 = property on="Vertical chart XY" class="XYGraph (strict)"("AnntList"=w2907) -> ()  [unwired: 2 in, 2 out]
      }
      event User Event {
        n1017 = event-data() -> ()  [unwired: 1 in, 4 out]
      }
    }
    n1018 = local write "Scan Image Pixel Value Loop error out"(w2277) -> ()
    "Scan Pixel Value Loop" <- w2282
  }
  n1019 = call "IMAQ Dispose"("Image"=w93) -> ()  [unwired: 5 in, 1 out]
  n1020 = while "Horiz/Vert Chart Loop" {
    shift-right: [w2932] -> w137
    shift-left: w141 -> [w2934]
    tunnel: w140 -> [w2935]
    shift-right: [w2929] -> _
    shift-left: w138 -> [w2931]
    shift-right: [w2928] -> _
    shift-left: w138 -> [w2930]
    shift-right: [w2925] -> _
    shift-left: w131 -> [w2926]
    shift-right: [w2924] -> _
    shift-left: w131 -> [w2927]
    shift-right: [w2921] -> _
    shift-left: w129 -> [w2923]
    shift-right: [w2920] -> _
    shift-left: w128 -> [w2922]
    tunnel: w79 -> [w2919]
    i -> [w2937]
    stop <- w2933 stop-if-true
    n1021 = event shown="[2] <Analysis Step 3>: User Event" {
      selector: w2935 -> [_ _ _ _]
      dyn-events: _ -> [_ _ _ _]
      timeout: -1 -> [_ _ _ _]
      tunnel: w2934 -> [w2944 w2952 _ w3129]
      tunnel: [w2944 w2952 w2972 w3129] -> w2932
      tunnel: [_ TRUE _ _] -> w2933
      tunnel: w2931 -> [w2943 w2950 w3019 _]
      tunnel: w2930 -> [w2942 w2949 w3012 _]
      tunnel: [w2943 w2950 w3021 _] -> w2929
      tunnel: [w2942 w2949 w3013 _] -> w2928
      tunnel: w2927 -> [w2940 w2948 w3011 _]
      tunnel: w2926 -> [w2941 w2947 w3020 _]
      tunnel: [w2941 w2947 w3019 _] -> w2925
      tunnel: [w2940 w2948 w3012 _] -> w2924
      tunnel: w2923 -> [w2939 w2946 w2995 _]
      tunnel: w2922 -> [w2938 w2945 w2978 _]
      tunnel: [w2939 w2946 w2981 _] -> w2921
      tunnel: [w2938 w2945 w2976 _] -> w2920
      tunnel: w2919 -> [_ _ w2959 _]
      event Timeout {
        n1022 = event-data() -> ()  [unwired: 1 in, 2 out]
      }
      event User Event {
        n1023 = event-data() -> ()  [unwired: 1 in, 4 out]
      }
      event User Event {
        w2982 = 1.01 ("y")
        w2997 = u32 0 ("Active Cursor")
        w2994 = u32 0 ("Active Cursor")
        # "Needed because camera\nchange triggers an error here"
        # "A rotation around\n90 degree can be\nadjusted relatively\neasy"
        # "manual scale of y-axes:\nMax Range schould be 1% \nmore than max value"
        n1024 = event-data() -> ("Data"=w2993:u8[][], "Height"=w2969:i32, "Width"=w2967:i32, "Save path out Horizontal"=w2956:path, "Save path out Vertical"=w2955:path)  [unwired: 1 in]
        n1025 = call "IMAQController.get i attribute.vi"("i ref in"=w2959, "error in (no error)"=errorcluster {"status"=FALSE, "code"=0, "source"=""} ("error out")) -> ("i ref out"=w2958:refnum<vi>, "i attribute"=w2966:T17, "error out"=w2960:errorcluster)  [unwired: 15 in]
        n1026 = disable-structure shown="Disabled" {
          frame Disabled {
            n1027 = call "IMAQ LinearAverages"() -> ()  [unwired: 7 in, 5 out]
          }
          frame Enabled {
          }
        }
        n1028 = Unbundle By Name(w2966) -> ("activeCamera.Center Coordinates.Horizontal"=w2965:i32, "activeCamera.Center Coordinates.Vertical"=w2964:i32, "activeCamera.PixelPermm.Horizontal"=w2963:dbl, "activeCamera.PixelPermm.Vertical"=w2962:dbl, "activeCamera.Rotation"=w2954:dbl)
        n1029 = Absolute Value(x=w2954) -> ()  [unwired: 1 out]
        n1030 = case shown="90, 270" 0 {
          tunnel: w2969 -> [w3030 w3032]
          tunnel: [w3029 w3032] -> w2968
          tunnel: w2967 -> [w3029 w3031]
          tunnel: [w3030 w3031] -> w2957
          frame 90, 270 {
          }
          frame Default {
          }
        }
        n1031 = Reciprocal(x=w2963) -> (1/x=w2971:dbl)
        n1032 = Reciprocal(x=w2962) -> (1/x=w2970:dbl)
        n1033 = Subtract(x=w2957, y=w2965) -> (x-y=w3007:i32)
        n1034 = Negate(x=w2965) -> (-x=w3010:i32)
        n1035 = Multiply(x=w3007, y=w2971) -> (x*y=w3006:dbl)
        n1036 = Array Size(array=w2993) -> (size(s)=w3028:i32[])
        n1037 = Multiply(x=w2965, y=w2971) -> (x*y=w3009:dbl)
        n1038 = Multiply(x=w2971, y=w3010) -> (x*y=w2998:dbl)
        n1039 = Negate(x=w3009) -> (-x=w3008:dbl)
        n1040 = Index Array(array=w3028, index #1=0 ("index")) -> (element #1=w3026:i32, element #2=w3025:i32)  [unwired: 1 in]
        n1041 = for {
          N: w3025 -> [_]
          tunnel: w2993 -> [w3121]
          tunnel: [w3119] -> w3021 mode=indexing
          tunnel: w3026 -> [w3118]
          tunnel: [w3117] -> w3018 mode=indexing
          i -> [w3117]
          n1042 = for {
            N: w3118 -> [_]
            tunnel: w3121 -> [w3127]
            tunnel: w3117 -> [w3122]
            shift-right: [w3124] -> w3119
            shift-left: 0 -> [w3125]
            i -> [w3123]
            n1043 = Index Array(array=w3127, index (row)=w3123, index (col)=w3122) -> (element=w3126:u8)
            n1044 = Add(x=w3125, y=w3126) -> (x+y=w3124:i32)
          }
        }
        n1045 = for {
          N: w3026 -> [_]
          tunnel: w2993 -> [w3110]
          tunnel: [w3108] -> w3013 mode=indexing
          tunnel: w3025 -> [w3107]
          tunnel: [w3106] -> w3014 mode=indexing
          i -> [w3106]
          n1046 = for {
            N: w3107 -> [_]
            tunnel: w3110 -> [w3116]
            tunnel: w3106 -> [w3111]
            shift-right: [w3113] -> w3108
            shift-left: 0 -> [w3114]
            i -> [w3112]
            n1047 = Index Array(array=w3116, index (row)=w3111, index (col)=w3112) -> (element=w3115:u8)
            n1048 = Add(x=w3114, y=w3115) -> (x+y=w3113:i32)
          }
        }
        n1049 = Subtract(x=w2968, y=w2964) -> (x-y=w3004:i32)
        n1050 = Negate(x=w2964) -> (-x=w2999:i32)
        n1051 = Multiply(x=w3004, y=w2970) -> (x*y=w3003:dbl)
        n1052 = Multiply(x=w2964, y=w2970) -> (x*y=w3001:dbl)
        n1053 = Multiply(x=w2970, y=w2999) -> (x*y=w3000:dbl)
        n1054 = Negate(x=w3001) -> (-x=w3002:dbl)
        n1055 = Divide(x=w3021, y=w2968) -> (x/y=w2992:dbl[])
        n1056 = Divide(x=w3019, y=w2968) -> (x/y=w2991:dbl[])
        n1057 = Divide(x=w3020, y=w2968) -> (x/y=w2990:dbl[])
        n1058 = Divide(x=w3013, y=w2957) -> (x/y=w2989:dbl[])
        n1059 = Divide(x=w3012, y=w2957) -> (x/y=w2988:dbl[])
        n1060 = Divide(x=w3011, y=w2957) -> (x/y=w2987:dbl[])
        n1061 = Bundle(w3018, w2992) -> (w3022:cluster{i32[], dbl[]})  [unwired: 1 in]
        n1062 = Bundle(w3018, w2991) -> (w3023:cluster{i32[], dbl[]})  [unwired: 1 in]
        n1063 = Bundle(w3018, w2990) -> (w3024:cluster{i32[], dbl[]})  [unwired: 1 in]
        n1064 = Bundle(w3014, w2989) -> (w3017:cluster{i32[], dbl[]})  [unwired: 1 in]
        n1065 = Bundle(w3014, w2988) -> (w3016:cluster{i32[], dbl[]})  [unwired: 1 in]
        n1066 = Bundle(w3014, w2987) -> (w3015:cluster{i32[], dbl[]})  [unwired: 1 in]
        n1067 = Build Array(w2992, w2991, w2990) -> (w2986:dbl[][])
        n1068 = Build Array(w3022, w3023, w3024) -> (w2975:cluster{i32[], dbl[]}[])
        n1069 = Build Array(w2989, w2988, w2987) -> (w2985:dbl[][])
        n1070 = Build Array(w3017, w3016, w3015) -> (w2974:cluster{i32[], dbl[]}[])
        n1071 = Array Max & Min(array=w2986) -> (max value=w2984:dbl)  [unwired: 3 out]
        n1072 = Array Max & Min(array=w2985) -> (max value=w2983:dbl)  [unwired: 3 out]
        n1073 = Multiply(x=w2984, y=w2982) -> (x*y=w2981:dbl)
        n1074 = property on="Horizontal chart XY" class="XYGraph (strict)"(error in=w2960, "XScale.Multiplier"=w2971, "XScale.Offset"=w3008, "XScale.Maximum"=w3006, "XScale.Minimum"=w2998, "Active Cursor"=w2994, "Cursor.Cursor X"=w2994, "YScale.Maximum"=w2981) -> (error out=w3005:errorcluster)  [unwired: 1 in, 1 out]
        n1075 = Not Equal?(x=w2981, y=w2995) -> (x != y?=w2996:bool)
        n1076 = Multiply(x=w2983, y=w2982) -> (x*y=w2976:dbl)
        n1077 = property on="Vertical chart XY" class="XYGraph (strict)"(error in=w3005, "XScale.Multiplier"=w2970, "XScale.Offset"=w3002, "XScale.Maximum"=w3003, "XScale.Minimum"=w3000, "Active Cursor"=w2997, "Cursor.Cursor X"=w2997, "YScale.Maximum"=w2976) -> (error out=w2980:errorcluster)  [unwired: 1 in, 1 out]
        n1078 = Not Equal?(x=w2976, y=w2978) -> (x != y?=w2979:bool)
        n1079 = case shown="True" w2979 {
          tunnel: w2980 -> [w3078 w3091]
          tunnel: [w3078 w3089] -> w2977
          tunnel: w2976 -> [_ w3083]
          tunnel: w2978 -> [_ w3082]
          frame False {
          }
          frame True {
            n1080 = Divide(x=w3083, y=w3082) -> (x/y=w3080:dbl)
            n1081 = property on="Vertical chart XY" class="XYGraph (strict)"(error in=w3091) -> (error out=w3090:errorcluster, "AnntList"=w3088:T27)  [unwired: 1 in, 1 out]
            n1082 = Index Array(array=w3088, index=0) -> (element=w3086:T24)
            n1083 = Unbundle By Name(w3086) -> ("Position.Y"=w3081:dbl)
            n1084 = Multiply(x=w3081, y=w3080) -> (x*y=w3079:dbl)
            n1085 = Bundle By Name(cluster=w3086, "Position.Y"=w3079) -> (w3084:T24)
            n1086 = Build Array(w3084) -> (w3085:T25)
            n1087 = property on="Vertical chart XY" class="XYGraph (strict)"(error in=w3090, "AnntList"=w3085) -> (error out=w3089:errorcluster)  [unwired: 1 in, 1 out]
          }
        }
        n1088 = case shown="True" w2996 {
          tunnel: w2977 -> [w3092 w3105]
          tunnel: [w3092 w3103] -> w2973
          tunnel: w2981 -> [_ w3097]
          tunnel: w2995 -> [_ w3096]
          frame False {
          }
          frame True {
            n1089 = Divide(x=w3097, y=w3096) -> (x/y=w3094:dbl)
            n1090 = property on="Horizontal chart XY" class="XYGraph (strict)"(error in=w3105) -> (error out=w3104:errorcluster, "AnntList"=w3102:T27)  [unwired: 1 in, 1 out]
            n1091 = Index Array(array=w3102, index=0) -> (element=w3100:T24)
            n1092 = Unbundle By Name(w3100) -> ("Position.Y"=w3095:dbl)
            n1093 = Multiply(x=w3095, y=w3094) -> (x*y=w3093:dbl)
            n1094 = Bundle By Name(cluster=w3100, "Position.Y"=w3093) -> (w3098:T24)
            n1095 = Build Array(w3098) -> (w3099:T25)
            n1096 = property on="Horizontal chart XY" class="XYGraph (strict)"(error in=w3104, "AnntList"=w3099) -> (error out=w3103:errorcluster)  [unwired: 1 in, 1 out]
          }
        }
        n1097 = stacked-sequence {
          seq-local: [w3034 _] -> [_ w3075]
          seq-local: [w3033 _] -> [_ w3074]
          tunnel: w2975 -> [w3059 w3077]
          tunnel: w2974 -> [w3058 w3076]
          tunnel: w2973 -> [w3038 _]
          tunnel: [w3060 _] -> w2972
          tunnel: w2965 -> [w3045 _]
          tunnel: w2964 -> [w3046 _]
          tunnel: w2971 -> [w3040 _]
          tunnel: w2970 -> [w3039 _]
          tunnel: w2958 -> [w3037 _]
          tunnel: w2956 -> [w3036 _]
          tunnel: w2955 -> [w3035 w3071]
          frame #0 {
            w3057 = 0 ("index")
            n1098 = Index Array(array=w3059, index=w3057) -> (element=w3056:cluster{i32[], dbl[]})
            n1099 = Index Array(array=w3058, index=w3057) -> (element=w3055:cluster{i32[], dbl[]})
            n1100 = local read "auto save"() -> (w3061:bool)
            n1101 = Unbundle(w3056) -> (w3048:i32[], w3054:dbl[])
            n1102 = Unbundle(w3055) -> (w3047:i32[], w3053:dbl[])
            n1103 = Subtract(x=w3048, y=w3045) -> (x-y=w3042:i32[])
            n1104 = Subtract(x=w3047, y=w3046) -> (x-y=w3044:i32[])
            n1105 = Multiply(x=w3042, y=w3040) -> (x*y=w3041:dbl[])
            n1106 = Multiply(x=w3044, y=w3039) -> (x*y=w3043:dbl[])
            n1107 = Build Array(w3041, w3054) -> (w3052:dbl[][])
            n1108 = Build Array(w3043, w3053) -> (w3050:dbl[][])
            n1109 = Transpose 2D Array(2D array=w3052) -> (transposed array=w3051:dbl[][])
            n1110 = Transpose 2D Array(2D array=w3050) -> (transposed array=w3049:dbl[][])
            n1111 = case shown="True" w3061 {
              tunnel: [w3064 w3069] -> w3060
              tunnel: w3049 -> [w3062 w3065]
              tunnel: w3051 -> [w3063 w3066]
              tunnel: w3038 -> [w3064 w3069]
              tunnel: w3037 -> [_ _]
              tunnel: w3036 -> [_ w3068]
              tunnel: w3035 -> [_ w3067]
              tunnel: [w3063 w3066] -> w3034
              tunnel: [w3062 w3065] -> w3033
              frame False {
              }
              frame True {
                n1112 = call-poly <vilib>:"Write To Spreadsheet File.vi"("2D data"=w3066, "file path (dialog if empty)"=w3068) -> ()  [unwired: 6 in, 1 out]
                n1113 = call-poly <vilib>:"Write To Spreadsheet File.vi"("2D data"=w3065, "file path (dialog if empty)"=w3067) -> ()  [unwired: 6 in, 1 out]
              }
            }
          }
          frame #1 {
            n1114 = local read "Proj Up"() -> (w3073:i32)
            n1115 = Strip Path(path=w3071) -> (name=→"AnaStep3":string)  [unwired: 1 out]
            n1116 = Increment(x=w3073) -> (x+1=→"Proj Up":i32)
            "Horizontal chart XY" <- w3077
            "Vertical chart XY" <- w3076
            "ActHorizontalProj" <- w3075
            "ActVerticalProj" <- w3074
          }
        }
      }
      event User Event {
        w3128 = cluster{i32[], dbl[]}[] [] ("Horizontal chart XY")
        n1117 = event-data() -> ()  [unwired: 1 in, 1 out]
        n1118 = local write "Horizontal chart XY"(w3128) -> ()
        n1119 = local write "Vertical chart XY"(w3128) -> ()
      }
    }
    n1120 = local write "Horiz/Vert Chart error out"(w2932) -> ()
    "Horiz/Vert Chart Loop" <- w2937
  }
  n1121 = while "Logger Loop" {
    tunnel: w36 -> [w3137]
    tunnel: w30 -> [w3135]
    tunnel: [w3134] -> w29
    shift-right: [w3132] -> _
    shift-left: w27 -> [w3133]
    shift-right: [w3131] -> _
    shift-left: 1 -> [w3130]
    stop <- w3136 stop-if-true
    n1122 = event shown="[2] <Logger Update>: User Event" {
      selector: w3137 -> [_ _ _ _]
      dyn-events: _ -> [_ _ _ _]
      timeout: -1 -> [_ _ _ _]
      tunnel: [_ TRUE _ _] -> w3136
      tunnel: w3135 -> [w3141 w3144 w3168 w3203]
      tunnel: [w3141 w3144 w3160 w3202] -> w3134
      tunnel: w3133 -> [w3140 w3143 w3150 w3201]
      tunnel: [w3140 w3143 w3149 w3201] -> w3132
      tunnel: [w3139 w3142 w3147 w3199] -> w3131
      tunnel: w3130 -> [w3139 w3142 w3146 w3200]
      event Timeout {
        n1123 = event-data() -> ()  [unwired: 1 in, 2 out]
      }
      event User Event {
        n1124 = event-data() -> ()  [unwired: 1 in, 4 out]
      }
      event User Event {
        n1125 = event-data() -> ("Message"=w3161:string, "Error?"=w3162:bool, "current time"=w3163:timestamp)  [unwired: 1 in]
        n1126 = Bundle("Message"=w3161, "Error?"=w3162, "current time"=w3163, "Msg#"=w3150) -> (w3167:T28)  [unwired: 1 in]
        n1127 = Lossy Enqueue Element(queue=w3168, element=w3167) -> (queue out=w3166:refnum<queue>)  [unwired: 1 in, 3 out]
        n1128 = property on="Logger String" class="Str"("Text.Selection Start"=u32 0 ("Text.Selection:Start"), "Text.Selection End"=w3146, "Text.FontColor"=u32 0) -> (error out=w3151:errorcluster)  [unwired: 2 in, 1 out]
        n1129 = Get Queue Status(queue=w3166, return elements? (F)=TRUE) -> (queue out=w3160:refnum<queue>, elements=w3164:T29)  [unwired: 1 in, 6 out]
        n1130 = for {
          N -> [w3179]
          tunnel: w3164 -> [w3198] mode=indexing
          tunnel: [w3183] -> w3159 mode=indexing
          tunnel: [w3178] -> w3157 mode=indexing if=w3184
          tunnel: [w3182] -> w3155 mode=indexing
          tunnel: w3151 -> [_]
          i -> [w3181]
          w3190 = ": "
          n1131 = Unbundle By Name(w3198) -> ("current time"=w3197:timestamp, "Message"=w3189:string, "Error?"=w3184:bool, "MsgNo"=w3177:i32)
          n1132 = Increment(x=w3181) -> (x+1=w3180:i32)
          n1133 = Equal?(x=w3179, y=w3180) -> (x = y?=w3188:bool)
          n1134 = Number To Decimal String(number=w3177) -> (decimal integer string=w3191:string)  [unwired: 1 in]
          n1135 = Select(t="", s=w3188, f="\r") -> (s? t:f=w3185:string)
          n1136 = Subtract(x=w3179, y=w3181) -> (x-y=w3178:i32)
          n1137 = Get Date/Time String(seconds (now)=w3197, want seconds? (F)=TRUE) -> (date string=w3195:string, time string=w3193:string)  [unwired: 1 in]
          n1138 = call <vilib>:"Space Constant.vi"() -> ("String"=w3194:string)
          n1139 = Concatenate Strings(w3185, w3195, w3194, w3193, w3190, "Msg " ("string"), w3191, w3190, w3189) -> (w3183:string)
          n1140 = String Length(string=w3183) -> (length=w3182:i32)
        }
        n1141 = Reverse 1D Array(array=w3159) -> (reversed array=w3158:string[])
        n1142 = Reverse 1D Array(array=w3155) -> (reversed array=w3154:i32[])
        n1143 = Reverse 1D Array(array=w3157) -> (reversed array=w3156:i32[])
        n1144 = Concatenate Strings(w3158) -> (w3148:string)
        "Logger String" <- w3148
        n1145 = for {
          tunnel: w3156 -> [w3174] mode=indexing
          tunnel: w3154 -> [w3175]
          n1146 = Decrement(x=w3174) -> (x-1=w3170:i32)
          n1147 = Index Array(array=w3175, index=w3170) -> (element=w3173:i32)
          n1148 = Array Subset(array=w3175, length=w3170) -> (w3176:i32[])  [unwired: 1 in]
          n1149 = Add Array Elements(numeric array=w3176) -> (sum=w3172:i32)
          n1150 = Add(x=w3173, y=w3172) -> (x+y=w3169:i32)
          n1151 = property on="Logger String" class="Str"("Text.Selection Start"=w3172, "Text.Selection End"=w3169, "Text.FontColor"=u32 16711680) -> ()  [unwired: 2 in, 2 out]
        }
        n1152 = String Length(string=w3148) -> (length=w3147:i32)
        n1153 = Increment(x=w3150) -> (x+1=w3149:i32)
      }
      event "Clear Log button": Value Change {
        n1154 = event-data() -> ("OldVal"=w3205:bool, "NewVal"=w3204:bool)  [unwired: 1 in]
        n1155 = local write "Clear Log button"(w3205) -> ()
        n1156 = case shown="True" w3204 {
          tunnel: w3203 -> [w3207 w3210]
          tunnel: [w3207 w3209] -> w3202
          tunnel: w3200 -> [w3206 _]
          tunnel: [w3206 _] -> w3199
          frame False {
          }
          frame True {
            n1157 = Flush Queue(queue=w3210) -> (queue out=w3209:refnum<queue>)  [unwired: 1 in, 2 out]
            n1158 = local write "Logger String"("") -> ()
          }
        }
      }
    }
  }
  n1159 = while "User Event Loop" {
    shift-right: [w3221] -> w155
    shift-left: w153 -> [w3219]
    tunnel: w152 -> [w3227]
    tunnel: w35 -> [w3225]
    shift-right: [w3224] -> w142
    shift-left: w105 -> [w3223]
    tunnel: w79 -> [w3222]
    shift-right: [w3218] -> _
    shift-left: w135 -> [w3220]
    tunnel: w132 -> [w3217]
    tunnel: w112 -> [w3216]
    tunnel: w3 -> [w3215]
    shift-right: [w3213] -> _
    shift-left: w70 -> [w3214]
    tunnel: w64 -> [w3212]
    tunnel: w1 -> [w3211]
    i -> [w3228]
    stop <- w3226 stop-if-true
    n1160 = case shown="False" w3220 {
      selector: w3220 -> [w3238 w4210]
      tunnel: w3227 -> [w3245 w4209]
      tunnel: [w3244 w4206] -> w3226
      tunnel: w3225 -> [w3243 _]
      tunnel: [w3242 w4211] -> w3224
      tunnel: w3223 -> [w3241 w4211]
      tunnel: w3222 -> [w3240 _]
      tunnel: [w3234 w4207] -> w3221
      tunnel: w3219 -> [w3239 w4205]
      tunnel: [w3237 w4204] -> w3218
      tunnel: w3217 -> [w3236 w4203]
      tunnel: w3216 -> [w3235 _]
      tunnel: w3215 -> [w3233 _]
      tunnel: w3214 -> [w3232 _]
      tunnel: [w3231 _] -> w3213
      tunnel: w3212 -> [w3230 _]
      tunnel: w3211 -> [w3229 _]
      frame False {
        n1161 = event shown="[10] \"Save this button\": Value Change" {
          selector: w3245 -> [_ _ _ _ _ _ _ _ _ _ _ _ _ _ _ _ _ _ _ _ _ _ _ _]
          dyn-events: _ -> [_ _ _ _ _ _ _ _ _ _ _ _ _ _ _ _ _ _ _ _ _ _ _ _]
          timeout: -1 -> [_ _ _ _ _ _ _ _ _ _ _ _ _ _ _ _ _ _ _ _ _ _ _ _]
          tunnel: w3239 -> [w3250 w3257 w3262 w3268 w3277 w3289 w3315 w3427 w3432 w3443 w3662 w3707 w3730 w3764 w3821 w3833 w3915 w3963 w3988 w4012 w4018 w4168 w4181 w4194]
          tunnel: [w3250 w3256 w3262 w3266 w3275 w3288 w3318 w3427 w3432 w3439 w3662 w3706 w3721 w3760 w3821 w3834 w3914 w3962 w3987 w4008 w4017 w4168 w4183 w4196] -> w3234
          tunnel: [_ _ TRUE _ _ _ _ _ _ _ _ _ _ _ _ _ _ _ _ _ _ _ _ _] -> w3244
          tunnel: w3243 -> [_ w3255 _ _ _ w3286 _ _ _ _ _ _ _ _ _ _ _ _ _ _ _ _ _ _]
          tunnel: w3241 -> [w3249 w3253 w3260 w3265 w3274 w3285 w3320 w3428 w3433 w3444 w3663 w3704 w3723 w3762 w3822 w3835 w3912 w3960 w3985 w4006 w4019 w4167 w4180 w4193]
          tunnel: [w3249 w3253 w3260 w3265 w3274 w3285 w3319 w3428 w3433 w3444 w3663 w3704 w3723 w3761 w3822 w3835 w3911 w3959 w3984 w4006 w4019 w4167 w4180 w4193] -> w3242
          tunnel: w3240 -> [_ _ _ _ _ w3284 w3314 _ _ w3440 w3660 w3702 _ w3759 _ w3832 w3913 w3961 w3986 _ _ _ _ _]
          tunnel: w3238 -> [w3248 w3252 w3259 w3264 w3273 w3283 w3316 _ _ _ _ w3703 w3722 w3758 _ w3830 w3910 w3958 w3983 _ _ _ w4179 w4192]
          tunnel: [w3248 w3252 w3259 w3264 w3273 w3283 w3316 _ _ _ _ w3703 w3722 w3758 _ w3830 w3910 w3958 w3983 _ _ _ w4179 w4192] -> w3237
          tunnel: w3236 -> [_ _ _ _ _ _ _ _ _ _ _ _ _ _ _ _ _ _ _ _ _ _ w4182 w4195]
          tunnel: w3235 -> [_ _ _ _ _ _ _ _ _ _ _ _ _ _ _ _ w3909 _ _ _ _ _ _ _]
          tunnel: w3233 -> [_ _ _ _ _ _ w3313 _ _ _ _ _ _ _ _ _ _ _ _ _ _ _ _ _]
          tunnel: w3232 -> [w3247 w3251 w3258 w3263 w3272 w3282 _ w3429 w3434 w3437 w3664 w3701 w3718 w3757 w3816 _ w3908 w3957 w3982 w4005 w4020 w4166 w4177 w4190]
          tunnel: [w3247 w3251 w3258 w3263 w3272 w3281 _ w3429 w3434 w3437 w3664 w3700 w3718 w3757 w3816 _ w3907 w3956 w3981 w4005 w4020 w4166 w4177 w4190] -> w3231
          tunnel: w3230 -> [_ _ _ _ _ _ _ _ _ _ w3661 _ _ _ _ _ _ _ _ _ _ _ _ _]
          tunnel: w3229 -> [_ _ _ _ _ _ _ _ _ _ w3659 _ _ _ _ _ w3906 _ _ _ _ _ _ _]
          event Timeout {
            n1162 = event-data() -> ()  [unwired: 1 in, 2 out]
          }
          event "stop button": Value Change; Panel Close {
            n1163 = event-data() -> ()  [unwired: 1 in, 2 out]
            n1164 = Generate User Event(user event=w3255, event data cluster=TRUE ("event data"), error in=w3257) -> (error out=w3256:errorcluster)  [unwired: 1 in, 1 out]
          }
          event User Event {
            n1165 = event-data() -> ()  [unwired: 1 in, 4 out]
          }
          event "Image Settings": Value Change {
            w3269 = u32 5 items=["Grayscale", "Binary", "Gradient", "Rainbow", "Temperature", "User Defined"] ("Palette:Palette Type")
            n1166 = event-data() -> ("NewVal"=w3267:cluster{u8, u8})  [unwired: 1 in, 4 out]
            n1167 = property on="ActImage"(error in=w3268, "Palette Type"=w3269) -> (error out=w3271:errorcluster)  [unwired: 1 in, 1 out]
            n1168 = call "ColorMap_Rainbow_LH.vi"("Limits (L:0,H:255)"=w3267) -> ("Rainbow_LH"=w3270:cluster{"Red":u8, "Green":u8, "Blue":u8}[])
            n1169 = property on="ActImage"(error in=w3271, "User Palette"=w3270) -> (error out=w3266:errorcluster)  [unwired: 1 in, 1 out]
          }
          event "Analysis Image Settings": Value Change {
            w3278 = u32 5 items=["Grayscale", "Binary", "Gradient", "Rainbow", "Temperature", "User Defined"] ("Palette:Palette Type")
            n1170 = event-data() -> ("NewVal"=w3276:cluster{u8, u8})  [unwired: 1 in, 4 out]
            n1171 = property on="ScanImage"(error in=w3277, "Palette Type"=w3278) -> (error out=w3280:errorcluster)  [unwired: 1 in, 1 out]
            n1172 = call "ColorMap_Rainbow_LH.vi"("Limits (L:0,H:255)"=w3276) -> ("Rainbow_LH"=w3279:cluster{"Red":u8, "Green":u8, "Blue":u8}[])
            n1173 = property on="ScanImage"(error in=w3280, "User Palette"=w3279) -> (error out=w3275:errorcluster)  [unwired: 1 in, 1 out]
          }
          event Menu Selection (User) {
            n1174 = event-data() -> ("ItemTag"=w3287:string)  [unwired: 1 in, 5 out]
            n1175 = case shown="\"QUIT\"" w3287 {
              tunnel: w3289 -> [w3291 w3295 w3301 w3309]
              tunnel: [w3291 w3294 w3301 w3309] -> w3288
              tunnel: w3286 -> [_ w3293 _ _]
              tunnel: w3284 -> [_ _ w3302 w3310]
              tunnel: w3282 -> [w3290 w3292 w3297 w3305]
              tunnel: [w3290 w3292 w3297 w3305] -> w3281
              frame Default {
              }
              frame "QUIT" {
                n1176 = Generate User Event(user event=w3293, event data cluster=TRUE ("event data"), error in=w3295) -> (error out=w3294:errorcluster)  [unwired: 1 in, 1 out]
              }
              frame "CONF_SEQUENCER" {
                n1177 = call "IMAQController.get i attribute.vi"("i ref in"=w3302, "error in (no error)"=w3301) -> ("i attribute"=w3300:T17, "error out"=w3298:errorcluster)  [unwired: 15 in, 1 out]
                n1178 = Unbundle By Name(w3300) -> ("actSequencer"=w3299:string)
                n1179 = call "CSSystemLib.name2ref.vi"("name"=w3299) -> ("obj refnum"=w3304:refnum<vi>)
                n1180 = call "CSObj.open front panel.vi"("i ref in"=w3304, "frontPanelOpen"=TRUE ("front panel open"), "error in (no error)"=w3298) -> ()  [unwired: 15 in, 2 out]
              }
              frame "CONF_SCAN" {
                n1181 = call "IMAQController.get i attribute.vi"("i ref in"=w3310, "error in (no error)"=w3309) -> ("i attribute"=w3308:T17, "error out"=w3306:errorcluster)  [unwired: 15 in, 1 out]
                n1182 = Unbundle By Name(w3308) -> ("actScanner"=w3307:string)
                n1183 = call "CSSystemLib.name2ref.vi"("name"=w3307) -> ("obj refnum"=w3312:refnum<vi>)
                n1184 = call "CSObj.open front panel.vi"("i ref in"=w3312, "frontPanelOpen"=TRUE ("front panel open"), "error in (no error)"=w3306) -> ()  [unwired: 15 in, 2 out]
              }
            }
          }
          event "Select Camera": Value Change {
            n1185 = event-data() -> ("NewVal"=w3317:u16)  [unwired: 1 in]
            n1186 = stacked-sequence {
              seq-local: [w3321 _ _] -> [_ w3341 _]
              seq-local: [_ w3336 _] -> [_ _ w3388]
              seq-local: [_ w3338 _] -> [_ _ w3382]
              tunnel: w3320 -> [w3329 _ _]
              tunnel: [_ w3351 _] -> w3319
              tunnel: [_ _ w3393] -> w3318
              tunnel: w3317 -> [_ w3342 _]
              tunnel: w3315 -> [w3326 _ _]
              tunnel: w3314 -> [_ _ w3387]
              tunnel: w3313 -> [_ _ w3385]
              frame #0 {
                # "Disconnect DIM Services for old camera"
                n1187 = stacked-sequence {
                  tunnel: w3326 -> [w3331 _]
                  tunnel: [w3330 _] -> w3324
                  frame #0 {
                    n1188 = call <vilib>:"Set Busy.vi"("error in (no error)"=w3331) -> ("error out"=w3330:errorcluster)  [unwired: 9 in, 1 out]
                  }
                  frame #1 {
                    n1189 = local write "Camera\nConnected?"(FALSE ("Camera\nConnected?")) -> ()
                  }
                }
                n1190 = property on="Connection status" class="Bool (strict)"(error in=w3324, "Blinking"=TRUE) -> (error out=w3322:errorcluster)  [unwired: 1 in, 1 out]
                n1191 = for {
                  tunnel: w3329 -> [w3333] mode=indexing
                  shift-right: [w3334] -> w3327
                  shift-left: w3322 -> [w3335]
                  n1192 = call "LVDimInterface.dic_release_service.vi"("callBackID"=w3333, "error in (no error)"=w3335) -> ("error out"=w3334:errorcluster)  [unwired: 17 in]
                }
                n1193 = control-ref of="ActualImageLink(Compression Mode)"() -> (w3328:refnum<vi>)
                n1194 = call "DimIndicators.dic_release_service.vi"("controlRef"=w3328, "error in (no error)"=w3327) -> ("error out"=w3321:errorcluster)  [unwired: 17 in]
                n1195 = local write "Overlay configured?"(FALSE ("OverlayAlreadyConfigured?")) -> ()
              }
              frame #1 {
                # "Connect DIM Services for new camera"
                n1196 = property on="Select Camera" class="Ring (strict)"(error in=w3341) -> (error out=w3337:errorcluster, "Strings []"=w3343:string[])  [unwired: 1 in, 1 out]
                n1197 = Index Array(array=w3343, index=w3342) -> (element=w3340:string)
                n1198 = Match Pattern(string=w3340, regular expression="HITRAP ") -> (after substring=w3338:string)  [unwired: 1 in, 3 out]
                n1199 = local read "DIM Array"() -> (w3346:refnum<queue>[])
                n1200 = Concatenate Strings(w3338, "_NumberOfImages" ("string")) -> (w3359:string)
                n1201 = call "LVDimInterface.dic_info_service_once.vi"("serviceName"=w3359, "error in (no error)"=w3337) -> ("data"=w3358:i8[], "error out"=w3348:errorcluster)  [unwired: 14 in, 2 out]
                n1202 = Type Cast(type=u16 0 ("data"), x=w3358) -> (*(type *) &x=w3345:u16)
                n1203 = for {
                  shift-right: [w3363] -> w3347
                  shift-left: w3348 -> [w3364]
                  tunnel: w3346 -> [w3361] mode=indexing
                  n1204 = Release Queue(queue=w3361, force destroy? (F)=TRUE, error in (no error)=w3364) -> (error out=w3363:errorcluster)  [unwired: 2 out]
                }
                n1205 = Concatenate Strings(w3338, "_Image" ("string")) -> (w3354:string)
                n1206 = for {
                  N: w3345 -> [_]
                  shift-right: [w3379] -> w3355
                  shift-left: w3347 -> [w3368]
                  tunnel: [w3378] -> w3351 mode=indexing
                  tunnel: w3354 -> [w3369]
                  tunnel: i8[] [] -> [w3366]
                  tunnel: [w3365] -> w3344 mode=indexing
                  i -> [w3371]
                  w3377 = T22 4 items=["ONCE_ONLY"=1, "TIMED"=2, "MONITORED"=4] ("serviceType")
                  n1207 = Increment(x=w3371) -> (x+1=w3373:i32)
                  n1208 = Number To Decimal String(number=w3373) -> (decimal integer string=w3372:string)  [unwired: 1 in]
                  n1209 = Obtain Queue(element data type=w3366, error in (no error)=w3368) -> (queue out=w3365:refnum<queue>, error out=w3367:errorcluster)  [unwired: 3 in, 1 out]
                  n1210 = Concatenate Strings(w3369, "_", w3372) -> (w3370:string)
                  n1211 = call-poly "LVDimInterface.dic_info_service.vi"("serviceName"=w3370, "queueRef"=w3365, "timeout [s]"=0, "serviceType"=w3377, "error in (no error)"=w3367, "stamped"=FALSE) -> ("callBackID"=w3378:i32, "error out"=w3379:errorcluster)  [unwired: 12 in]
                }
                n1212 = control-ref of="ActualImageLink(Compression Mode)"() -> (w3352:refnum<vi>)
                n1213 = local write "DIM Array"(w3344) -> ()
                n1214 = Concatenate Strings(w3338, "_Image_JPEG" ("string")) -> (w3356:string)
                n1215 = call "DimIndicators.dic_info_service.vi"("controlRef"=w3352, "serviceName"=w3356, "error in (no error)"=w3355) -> ("error out"=w3336:errorcluster)  [unwired: 15 in, 1 out]
              }
              frame #2 {
                # "beim camera change alle plots löschen!!"
                n1216 = Generate User Event(user event=w3385, event data cluster=TRUE ("event data")) -> ()  [unwired: 2 in, 2 out]
                n1217 = call "IMAQController.get data to modify.vi"("i ref in"=w3387, "error in (no error)"=w3388) -> ("i ref out"=w3386:refnum<vi>, "i attribute"=w3392:T17, "timed out"=w3391:bool, "error out"=w3390:errorcluster)  [unwired: 14 in]
                n1218 = case shown="False" w3391 {
                  tunnel: w3392 -> [w3405 _]
                  tunnel: w3390 -> [w3401 w3412]
                  tunnel: [w3400 w3412] -> w3389
                  tunnel: w3386 -> [w3399 w3411]
                  tunnel: w3382 -> [w3397 _]
                  tunnel: [w3396 w3411] -> w3383
                  frame False {
                    n1219 = Unbundle By Name(w3405) -> ("activatedCameras"=w3403:T19)
                    n1220 = while {
                      tunnel: w3403 -> [w3409] mode=indexing
                      tunnel: w3397 -> [w3410]
                      tunnel: [w3406] -> w3402
                      i -> [w3406]
                      stop <- w3407 stop-if-true
                      n1221 = Unbundle By Name(w3409) -> ("Name"=w3408:string)
                      n1222 = Equal?(x=w3408, y=w3410) -> (x = y?=w3407:bool)
                    }
                    n1223 = Index Array(array=w3403, index=w3402) -> (element=w3398:T32)
                    n1224 = Bundle By Name(cluster=w3405, "activeCamera"=w3398, "actCamera"=w3397) -> (w3404:T17)
                    n1225 = call "IMAQController.set modified data.vi"("i ref in"=w3399, "i attribute"=w3404, "error in (no error)"=w3401) -> ("i ref out"=w3396:refnum<vi>, "error out"=w3400:errorcluster)  [unwired: 15 in]
                  }
                  frame True {
                  }
                }
                n1226 = local read "Acquisition mode (Buffer)"() -> (w3381:T2)
                n1227 = case shown="\"Scan\", \"External Trigger\"" w3381 {
                  tunnel: [0 1] -> w3380
                  frame Default {
                  }
                  frame "Scan", "External Trigger" {
                  }
                }
                n1228 = stacked-sequence {
                  tunnel: w3389 -> [w3417 _ w3422]
                  tunnel: [_ _ w3422] -> w3393
                  tunnel: w3383 -> [w3416 _ _]
                  tunnel: w3382 -> [w3414 _ _]
                  tunnel: w3380 -> [w3413 _ _]
                  frame #0 {
                    # "To be sure"
                    n1229 = call-poly "CoreLib.data 2 byte array.vi"("i32"=w3413) -> ("byteArray out"=w3415:T26)  [unwired: 18 in]
                    n1230 = call "BaseProcess.call process 2.vi"("i ref in"=w3416, "Object"=w3414, "Selector"="SetTriggerMode", "Data"=w3415, "error in (no error)"=w3417) -> ()  [unwired: 13 in, 2 out]
                  }
                  frame #1 {
                    n1231 = local write "Camera\nConnected?"(TRUE ("Camera\nConnected?")) -> ()
                    n1232 = local write "Overlay configured?"(FALSE ("Overlay configured?")) -> ()
                  }
                  frame #2 {
                    n1233 = Unbundle By Name(w3422) -> ("status"=w3423:bool, "source"=w3421:string)
                    n1234 = property on="Connection status" class="Bool (strict)"("Blinking"=FALSE) -> ()  [unwired: 2 in, 2 out]
                    n1235 = property on="Connection status" class="Bool (strict)"("TipStrip"=w3421) -> ()  [unwired: 2 in, 2 out]
                    n1236 = call <vilib>:"Unset Busy.vi"() -> ()  [unwired: 11 in, 1 out]
                    n1237 = local write "Connection status"(w3423) -> ()
                  }
                }
              }
            }
          }
          event Key Down {
            n1238 = event-data() -> ("VKey"=w3426:T30)  [unwired: 1 in, 3 out]
            n1239 = Equal?(x=eventvkey."F1" ("VKey"), y=w3426) -> ()  [unwired: 1 out]
          }
          event "Show all data": Value Change {
            n1240 = event-data() -> ("NewVal"=w3430:bool)  [unwired: 1 in]
            n1241 = case shown="False" w3430 {
              tunnel: [T21."Enabled" ("Disabled") T21."Disabled and Grayed Out" ("Disabled")] -> w3431
              frame False {
              }
              frame True {
              }
            }
            n1242 = property on="# shown Plots:" class="DigNum (strict)"("DisabledEnum"=w3431) -> ()  [unwired: 2 in, 2 out]
          }
          event "Camera Choice": Value Change {
            n1243 = event-data() -> ("NewVal"=w3442:i32[], "OldVal"=w3441:i32[])  [unwired: 1 in]
            n1244 = call <vilib>:"Set Busy.vi"("error in (no error)"=w3443) -> ("error out"=w3438:errorcluster)  [unwired: 9 in, 1 out]
            n1245 = stacked-sequence {
              seq-local: [_ w3478 _ _] -> [_ _ w3601 _]
              seq-local: [w3451 _ _ _] -> [_ w3477 w3606 _]
              seq-local: [w3456 _ _ _] -> [_ w3470 w3605 _]
              seq-local: [w3452 _ _ _] -> [_ w3474 w3609 _]
              seq-local: [w3450 _ _ _] -> [_ w3473 w3604 _]
              seq-local: [w3445 _ _ _] -> [_ w3472 _ _]
              seq-local: [_ w3471 _ _] -> [_ _ _ w3657]
              tunnel: w3442 -> [w3457 _ _ _]
              tunnel: w3441 -> [w3456 _ _ _]
              tunnel: w3438 -> [w3455 w3480 _ _]
              tunnel: w3440 -> [_ w3479 _ _]
              tunnel: [_ _ w3616 _] -> w3439
              frame #0 {
                # "The loop here is overkill, because NewVal\nshould only have exactly 1 element in"
                # "The reason for this is that I would like that the user\ncan add and substract a camera by just click with the left mouse button"
                n1246 = property on="Camera Choice" class="MCListbox (strict)"(error in=w3455) -> (error out=w3454:errorcluster, "ItemNames"=w3452:string[][])  [unwired: 1 in, 1 out]
                n1247 = for {
                  shift-right: [w3460] -> w3451
                  shift-left: w3456 -> [w3461]
                  tunnel: w3457 -> [w3458] mode=indexing
                  tunnel: [w3458] -> w3450
                  n1248 = Search 1D Array(1D array=w3461, element=w3458) -> (index of element=w3459:i32)  [unwired: 1 in]
                  n1249 = Greater?(x=w3459, y=-1) -> (0:w3463:bool)
                  n1250 = case shown="True" w3463 {
                    tunnel: w3461 -> [w3465 w3469]
                    tunnel: [w3466 w3468] -> w3460
                    tunnel: w3459 -> [_ w3467]
                    tunnel: w3458 -> [w3464 _]
                    frame False {
                      n1251 = Build Array (concatenate)(w3465, w3464) -> (w3466:i32[])
                    }
                    frame True {
                      n1252 = Delete From Array(array=w3469, index=w3467) -> (array with subset deleted=w3468:i32[])  [unwired: 1 in, 1 out]
                    }
                  }
                }
                "NewVal" <- w3451
                n1253 = property on="Connection status" class="Bool (strict)"(error in=w3454, "Blinking"=TRUE) -> (error out=w3449:errorcluster)  [unwired: 1 in, 1 out]
                n1254 = property on="Select Camera" class="Ring (strict)"(error in=w3449) -> (error out=w3448:errorcluster, "Strings []"=w3447:string[])  [unwired: 1 in, 1 out]
                n1255 = local write "Camera Choice"(w3451) -> ()
                n1256 = property on="Select Camera" class="Ring (strict)"(error in=w3448) -> ("Value"=w3446:u16)  [unwired: 1 in, 2 out]
                n1257 = Index Array(array=w3447, index=w3446) -> (element=w3445:string)
              }
              frame #1 {
                n1258 = Array Size(array=w3477) -> (size(s)=w3475:i32)
                n1259 = Array Size(array=w3470) -> (size(s)=w3476:i32)
                n1260 = Greater?(x=w3475, y=w3476) -> (0:w3481:bool)
                n1261 = case "Camera added?" shown="True" w3481 {
                  tunnel: w3480 -> [w3512 w3556]
                  tunnel: w3479 -> [w3513 w3557]
                  tunnel: [w3488 w3539] -> w3478
                  tunnel: w3474 -> [w3502 w3543]
                  tunnel: w3473 -> [w3498 w3535]
                  tunnel: w3472 -> [w3486 w3538]
                  tunnel: [w3482 _] -> w3471
                  tunnel: w3470 -> [_ w3536]
                  frame False {
                    # "Unload has to\nbe tested again"
                    n1262 = call "IMAQController.ReadConfigFile.vi"("object ref in"=w3513, "error in"=w3512) -> ("object ref out"=w3505:refnum<vi>, "Camera-System Configuration"=w3510:T33, "error out"=w3503:errorcluster)  [unwired: 15 in]
                    n1263 = Index Array(array=w3502, index (row)=w3498, index (col)=0 ("index (row)")) -> (element=w3499:string)
                    n1264 = Concatenate Strings("Camera_" ("string"), w3499) -> (w3490:string)
                    n1265 = while {
                      tunnel: w3510 -> [w3527] mode=indexing
                      tunnel: [w3525] -> w3504
                      tunnel: w3490 -> [w3523]
                      i -> [w3518]
                      stop <- w3522 stop-if-true
                      # "Max\n30 Systems"
                      n1266 = Unbundle By Name(w3527) -> ("SystemName"=w3525:string, "Camera-Name"=w3526:string[])
                      n1267 = for {
                        tunnel: w3526 -> [w3532] mode=indexing
                        tunnel: w3523 -> [w3531]
                        shift-right: [w3528] -> w3521
                        shift-left: FALSE -> [w3529]
                        n1268 = Equal?(x=w3532, y=w3531) -> (x = y?=w3530:bool)
                        n1269 = case shown="False" w3530 {
                          tunnel: w3529 -> [w3533 _]
                          tunnel: [w3533 TRUE] -> w3528
                          frame False {
                          }
                          frame True {
                          }
                        }
                      }
                      n1270 = Greater?(x=w3518, y=30.0) -> (0:w3520:bool)
                      n1271 = Or(x=w3520, y=w3521) -> (x .or. y?=w3522:bool)
                    }
                    n1272 = call-poly "CoreLib.data 2 byte array.vi"("string"=w3490) -> ("byteArray out"=w3500:T26)  [unwired: 18 in]
                    n1273 = Concatenate Strings(w3504, "\\Super" ("string")) -> (w3509:string)
                    n1274 = call "BaseProcess.call process 1.vi"("i ref in"=w3505, "Object"=w3509, "Selector"="KillObject", "CallType"=enum16{"simple", "synchronous", "asynchronous"}."synchronous", "Data"=w3500, "error in (no error)"=w3503) -> ("i ref out"=w3493:refnum<vi>, "error out"=w3494:errorcluster)  [unwired: 11 in, 1 out]
                    n1275 = call "IMAQController.SubCameraFromCameraList.vi"("i ref in"=w3493, "CS Camera Name"=w3490, "error in (no error)"=w3494) -> ("i ref out"=w3492:refnum<vi>, "error out"=w3491:errorcluster)  [unwired: 13 in, 2 out]
                    n1276 = call "IMAQController.get i attribute.vi"("i ref in"=w3492, "error in (no error)"=w3491) -> ("i attribute"=w3496:T17, "error out"=w3497:errorcluster)  [unwired: 15 in, 1 out]
                    n1277 = Unbundle By Name(w3496) -> ("activatedCameras"=w3495:T19)
                    n1278 = for {
                      tunnel: [w3516] -> w3487 mode=indexing
                      tunnel: w3495 -> [w3515] mode=indexing
                      n1279 = Unbundle By Name(w3515) -> ("Name"=w3514:string)
                      n1280 = Concatenate Strings("HITRAP " ("string"), w3514) -> (w3516:string)
                    }
                    n1281 = property on="Select Camera" class="Ring (strict)"(error in=w3497, "Strings []"=w3487) -> (error out=w3489:errorcluster)  [unwired: 1 in, 1 out]
                    n1282 = Search 1D Array(1D array=w3487, element=w3486) -> (index of element=w3485:i32)  [unwired: 1 in]
                    n1283 = Less Than 0?(x=w3485) -> (x < 0?=w3482:bool)
                    n1284 = Select(t=0, s=w3482, f=w3485) -> (s? t:f=w3484:i32)
                    n1285 = property on="Select Camera" class="Ring (strict)"(error in=w3489, "Value"=w3484) -> (error out=w3488:errorcluster)  [unwired: 1 in, 1 out]
                  }
                  frame True {
                    n1286 = call "IMAQController.ReadConfigFile.vi"("object ref in"=w3557, "error in"=w3556) -> ("object ref out"=w3558:refnum<vi>, "Camera-System Configuration"=w3555:T33, "error out"=w3542:errorcluster)  [unwired: 15 in]
                    n1287 = Index Array(array=w3543, index (row)=w3535, index (col)=0 ("index (row)")) -> (element=w3546:string)
                    n1288 = Concatenate Strings("Camera_" ("string"), w3546) -> (w3541:string)
                    n1289 = while {
                      tunnel: w3555 -> [w3592] mode=indexing
                      tunnel: [w3590] -> w3551
                      tunnel: w3541 -> [w3588]
                      i -> [w3583]
                      stop <- w3586 stop-if-true
                      # "Max\n30 Systems"
                      n1290 = Unbundle By Name(w3592) -> ("SystemName"=w3590:string, "Camera-Name"=w3591:string[])
                      n1291 = for {
                        tunnel: w3591 -> [w3597] mode=indexing
                        tunnel: w3588 -> [w3596]
                        shift-right: [w3593] -> w3587
                        shift-left: FALSE -> [w3594]
                        n1292 = Equal?(x=w3597, y=w3596) -> (x = y?=w3595:bool)
                        n1293 = case shown="False" w3595 {
                          tunnel: w3594 -> [w3598 _]
                          tunnel: [w3598 TRUE] -> w3593
                          frame False {
                          }
                          frame True {
                          }
                        }
                      }
                      n1294 = Greater?(x=w3583, y=30.0) -> (0:w3585:bool)
                      n1295 = Or(x=w3585, y=w3587) -> (x .or. y?=w3586:bool)
                    }
                    n1296 = call-poly "CoreLib.data 2 byte array.vi"("string"=w3541) -> ("byteArray out"=w3549:T26)  [unwired: 18 in]
                    n1297 = call-poly "CoreLib.data 2 byte array.vi"("byteArray"=w3549, "string"="IMAQDevice") -> ("byteArray out"=w3548:T26)  [unwired: 17 in]
                    n1298 = Concatenate Strings(w3551, "\\Super" ("string")) -> (w3554:string)
                    n1299 = call "BaseProcess.call process 1.vi"("i ref in"=w3558, "Object"=w3554, "Selector"="CreateObject", "CallType"=enum16{"simple", "synchronous", "asynchronous"}."synchronous", "Data"=w3548, "error in (no error)"=w3542) -> ("i ref out"=w3544:refnum<vi>, "error out"=w3537:errorcluster)  [unwired: 11 in, 1 out]
                    n1300 = case shown="No Error" w3537 {
                      selector: w3537 -> [w3559 w3582]
                      tunnel: w3544 -> [w3571 _]
                      tunnel: w3541 -> [w3570 _]
                      tunnel: [w3563 w3582] -> w3539
                      tunnel: w3538 -> [w3561 _]
                      tunnel: w3536 -> [_ w3581]
                      tunnel: w3535 -> [_ w3578]
                      frame No Error {
                        n1301 = call "IMAQController.AddCameraToCameraList.vi"("i ref in"=w3571, "CS Camera Name"=w3570, "error in (no error)"=w3559) -> ("i ref out"=w3566:refnum<vi>, "error out"=w3565:errorcluster)  [unwired: 13 in, 2 out]
                        n1302 = call "IMAQController.get i attribute.vi"("i ref in"=w3566, "error in (no error)"=w3565) -> ("i attribute"=w3568:T17, "error out"=w3569:errorcluster)  [unwired: 15 in, 1 out]
                        n1303 = Unbundle By Name(w3568) -> ("activatedCameras"=w3567:T19)
                        n1304 = for {
                          tunnel: [w3574] -> w3562 mode=indexing
                          tunnel: w3567 -> [w3573] mode=indexing
                          n1305 = Unbundle By Name(w3573) -> ("Name"=w3572:string)
                          n1306 = Concatenate Strings("HITRAP " ("string"), w3572) -> (w3574:string)
                        }
                        n1307 = property on="Select Camera" class="Ring (strict)"(error in=w3569, "Strings []"=w3562) -> (error out=w3564:errorcluster)  [unwired: 1 in, 1 out]
                        n1308 = Search 1D Array(1D array=w3562, element=w3561) -> (index of element=w3560:i32)  [unwired: 1 in]
                        n1309 = property on="Select Camera" class="Ring (strict)"(error in=w3564, "Value"=w3560) -> (error out=w3563:errorcluster)  [unwired: 1 in, 1 out]
                      }
                      frame Error {
                        # "Restore old values in case of error"
                        n1310 = property on="Camera Choice" class="MCListbox (strict)"("Value"=w3581) -> ()  [unwired: 2 in, 2 out]
                        n1311 = property on="Camera Choice" class="MCListbox (strict)"() -> ("ItemNames"=w3580:string[][])  [unwired: 2 in, 2 out]
                        n1312 = Replace Array Subset(array=w3580, new element="", index (row)=w3578, index (col)=3 ("disabled index (col)")) -> (w3579:string[][])
                        n1313 = property on="Camera Choice" class="MCListbox (strict)"("ItemNames"=w3579) -> ()  [unwired: 2 in, 2 out]
                      }
                    }
                  }
                }
              }
              frame #2 {
                n1314 = Array Size(array=w3609) -> (size(s)=w3618:i32[])
                n1315 = Array Size(array=w3606) -> (size(s)=w3607:i32)
                n1316 = Array Size(array=w3605) -> (size(s)=w3608:i32)
                n1317 = Index Array(array=w3618, index=0) -> (element=w3611:i32)
                n1318 = Greater?(x=w3607, y=w3608) -> (0:w3603:bool)
                n1319 = Initialize Array("not loaded" ("element"), w3611) -> (w3612:string[])
                n1320 = case shown="True" w3603 {
                  tunnel: [_ "0: 0: 0"] -> w3602
                  frame False {
                  }
                  frame True {
                  }
                }
                n1321 = Replace Array Subset(array=w3609, new element=w3612, index (col)=1 ("disabled index (col)")) -> (w3614:string[][])  [unwired: 1 in]
                n1322 = case shown="No Error" w3601 {
                  selector: w3601 -> [_ w3651]
                  tunnel: w3614 -> [w3626 _]
                  tunnel: w3606 -> [w3625 _]
                  tunnel: w3604 -> [w3622 _]
                  tunnel: w3602 -> [w3620 _]
                  tunnel: [_ w3651] -> w3600
                  frame No Error {
                    n1323 = for {
                      tunnel: w3625 -> [w3631] mode=indexing
                      tunnel: w3626 -> [w3646]
                      shift-right: [w3643] -> w3627
                      shift-left: dbl[] [] ("CameraTimeStamps") -> [w3644]
                      shift-right: [w3635] -> w3623
                      shift-left: w3626 -> [w3633]
                      w3641 = "Camera_" ("string")
                      n1324 = Index Array(array=w3646, index (row)=w3631, index (col)=0 ("disabled index (col)")) -> (element=w3640:string)
                      n1325 = Concatenate Strings(w3641, w3640, "_CameraType" ("string")) -> (w3638:string)
                      n1326 = Concatenate Strings(w3641, w3640, "_birthday" ("string")) -> (w3647:string)
                      n1327 = call "LVDimInterface.dic_info_service_once.vi"("serviceName"=w3638) -> ("data"=w3637:i8[])  [unwired: 15 in, 3 out]
                      n1328 = call "LVDimInterface.dic_info_service_once.vi"("serviceName"=w3647) -> ("data"=w3650:i8[])  [unwired: 15 in, 3 out]
                      n1329 = Type Cast(x=w3637) -> (*(type *) &x=w3636:string)  [unwired: 1 in]
                      n1330 = Type Cast(type=0.0, x=w3650) -> (*(type *) &x=w3642:dbl)
                      n1331 = Replace Array Subset(array=w3633, new element="loaded" ("new element/subarray"), index (row)=w3631, index (col)=1 ("disabled index (col)")) -> (w3632:string[][])
                      n1332 = Build Array (concatenate)(w3644, w3642) -> (w3643:dbl[])
                      n1333 = Replace Array Subset(array=w3632, new element=w3636, index (row)=w3631, index (col)=2 ("disabled index (col)")) -> (w3635:string[][])
                    }
                    n1334 = Replace Array Subset(array=w3623, new element=w3620, index (row)=w3622, index (col)=3) -> (w3621:string[][])
                    n1335 = property on="Camera Choice" class="MCListbox (strict)"("ItemNames"=w3621) -> ()  [unwired: 2 in, 2 out]
                    n1336 = local write "CameraTimeStamps"(w3627) -> ()
                  }
                  frame Error {
                  }
                }
                "Camera Choice error out" <- w3600
                n1337 = Unbundle By Name(w3600) -> ("status"=→"Connection status":bool)
                n1338 = case shown="Error" w3600 {
                  selector: w3600 -> [_ w3654]
                  tunnel: [_ w3653] -> w3615
                  frame No Error {
                  }
                  frame Error {
                    n1339 = Unbundle By Name(w3654) -> ("source"=w3653:string)
                  }
                }
                n1340 = flat-sequence {
                  tunnel: [w3656] -> w3616
                  tunnel: w3600 -> [_]
                  frame #0 {
                    n1341 = property on="Connection status" class="Bool (strict)"("Blinking"=FALSE) -> ()  [unwired: 2 in, 2 out]
                    n1342 = call <vilib>:"Unset Busy.vi"() -> ("error out"=w3656:errorcluster)  [unwired: 11 in]
                  }
                }
                n1343 = property on="Connection status" class="Bool (strict)"("TipStrip"=w3615) -> ()  [unwired: 2 in, 2 out]
              }
              frame #3 {
                # "If the active camera is destroyed als a \"Select Camera\" Event has to be triggered!!"
                n1344 = case shown="True" w3657 {
                  frame False {
                  }
                  frame True {
                    n1345 = property on="Select Camera" class="Ring (strict)"() -> ("Value"=w3658:u16)  [unwired: 2 in, 2 out]
                    n1346 = property on="Select Camera" class="Ring (strict)"("Val(Sgnl)"=w3658) -> ()  [unwired: 2 in, 2 out]
                  }
                }
              }
            }
          }
          event "Save this button": Value Change {
            n1347 = event-data() -> ("NewVal"=w3666:bool)  [unwired: 1 in]
            n1348 = case shown="True" w3666 {
              tunnel: w3661 -> [_ w3682]
              tunnel: w3660 -> [_ w3695]
              tunnel: w3659 -> [_ w3672]
              frame False {
              }
              frame True {
                w3675 = T12 {"Message"="", "Error?"=TRUE, "current time"=timestamp(0 s since 1904-01-01)}  # Logger String
                w3687 = refnum<vi> refnum  # ImageControl
                # "Problem ist momentan: Der Filename benutzt als Zeitstempel die Zeit, zu der auf den Butoon gedrückt wurde\nund nicht die Zeit, als das Bild entstand..."
                # "Diese Funktion ist nicht zur Anwendung während eines Scans vorgesehen!\nauch wenn die Vorbereitungen schon getroffen sind."
                # "Vielleicht andere Namenskonvention benutzen??"
                n1349 = call "IMAQController.get i attribute.vi"("i ref in"=w3695) -> ("i attribute"=w3694:T17)  [unwired: 16 in, 2 out]
                n1350 = control-ref of="ActImage"() -> (w3685:refnum<vi>)
                n1351 = Unbundle By Name(w3694) -> ("actScanner"=w3693:string)
                n1352 = local read "Save Path"() -> (w3678:path)
                n1353 = To More Specific Class(target class=w3687, reference=w3685) -> (specific class reference=w3689:refnum<vi>, error out=w3688:errorcluster)  [unwired: 1 in]
                n1354 = property on="Property Node" class="ImageControl"(reference=w3689, error in=w3688) -> ("User Palette"=w3686)  [unwired: 2 out]
                n1355 = call <vilib>:"Check if File or Folder Exists.vi"("path"=w3678) -> ("file or folder exists?"=w3677:bool)  [unwired: 8 in, 2 out]
                n1356 = case shown="False" w3677 {
                  tunnel: w3678 -> [_ w3699]
                  tunnel: [w3698 w3699] -> w3676
                  frame False {
                    n1357 = call <vilib>:"Dflt Data Dir.vi"() -> ("App:Default Data Directory"=w3698:path)
                  }
                  frame True {
                  }
                }
                n1358 = local read "Acquisition mode (Buffer)"() -> (w3697:T2)
                n1359 = Concatenate Strings(w3693, "_curStep" ("string")) -> (w3692:string)
                n1360 = call "IMAQ GetPalette"("Palette Number (gray)"=T31."Gray") -> ("Color Palette"=w3683:cluster{"Red":u8, "Green":u8, "Blue":u8}[])  [unwired: 4 in, 1 out]
                n1361 = call "IMAQController.SaveImage.vi"("Image"=w3682, "Save path in"=w3676, "Service name"=w3692, "Save?"=TRUE, "Save Overlay?"=FALSE, "Aqcuisation Mode"=w3697, "User Palette"=w3686, "Color Palette"=w3683) -> ("Save path out Horizontal"=w3670:path, "Save path out Verical"=w3681:path)  [unwired: 8 in, 2 out]
                n1362 = Strip Path(path=w3670) -> (name=w3667:string)  [unwired: 1 out]
                n1363 = Get Date/Time In Seconds() -> (seconds since 1Jan1904=w3674:timestamp)
                n1364 = Concatenate Strings("Image saved: " ("Message"), w3667) -> (w3669:string)
                n1365 = Bundle By Name(cluster=w3675, "Message"=w3669, "Error?"=FALSE, "current time"=w3674) -> (w3671:T12)
                n1366 = Generate User Event(user event=w3672, event data cluster=w3671) -> ()  [unwired: 2 in, 2 out]
                n1367 = local read "ActHorizontalProj"() -> (w3680:dbl[][])
                n1368 = local read "ActVerticalProj"() -> (w3679:dbl[][])
                n1369 = call-poly <vilib>:"Write To Spreadsheet File.vi"("2D data"=w3680, "file path (dialog if empty)"=w3670) -> ()  [unwired: 6 in, 1 out]
                n1370 = call-poly <vilib>:"Write To Spreadsheet File.vi"("2D data"=w3679, "file path (dialog if empty)"=w3681) -> ()  [unwired: 6 in, 1 out]
              }
            }
            n1371 = local write "Save this button"(FALSE ("Save this button")) -> ()
          }
          event "Configure Scan button": Value Change {
            n1372 = event-data() -> ("NewVal"=w3705:bool)  [unwired: 1 in]
            n1373 = case shown="True" w3705 {
              tunnel: w3707 -> [w3709 w3711]
              tunnel: [w3709 w3711] -> w3706
              tunnel: w3702 -> [_ w3712]
              tunnel: w3701 -> [w3708 w3710]
              tunnel: [w3708 w3710] -> w3700
              frame False {
              }
              frame True {
                n1374 = invoke on="Configure Scan button" class="Bool" method="Reinit To Default"() -> ()  [unwired: 3 in, 3 out]
                n1375 = call "IMAQController.get i attribute.vi"("i ref in"=w3712, "error in (no error)"=w3711) -> ("i attribute"=w3715:T17, "error out"=w3717:errorcluster)  [unwired: 15 in, 1 out]
                n1376 = Unbundle By Name(w3715) -> ("actScanner"=w3716:string)
                n1377 = call "CSSystemLib.name2ref.vi"("name"=w3716) -> ("obj refnum"=w3713:refnum<vi>)
                n1378 = call "CSObj.open front panel.vi"("i ref in"=w3713, "frontPanelOpen"=TRUE ("front panel open"), "error in (no error)"=w3717) -> ()  [unwired: 15 in, 2 out]
              }
            }
          }
          event "Save Analysis button": Value Change {
            w3732 = i16 2 ("width (-)")
            n1379 = event-data() -> ()  [unwired: 1 in, 5 out]
            n1380 = Get Date/Time In Seconds() -> (seconds since 1Jan1904=w3746:timestamp)
            n1381 = Seconds To Date/Time(time stamp (now)=w3746) -> (date time rec=w3745:T34)  [unwired: 1 in]
            n1382 = Unbundle By Name(w3745) -> ("year"=w3744:i32, "month"=w3743:i32, "day of month"=w3742:i32, "hour"=w3741:i32, "minute"=w3740:i32, "second"=w3739:i32)
            n1383 = Number To Decimal String(number=w3744) -> (decimal integer string=w3738:string)  [unwired: 1 in]
            n1384 = Number To Decimal String(number=w3743, width (-)=w3732) -> (decimal integer string=w3737:string)
            n1385 = Number To Decimal String(number=w3742, width (-)=w3732) -> (decimal integer string=w3736:string)
            n1386 = Number To Decimal String(number=w3741, width (-)=w3732) -> (decimal integer string=w3733:string)
            n1387 = Number To Decimal String(number=w3740, width (-)=w3732) -> (decimal integer string=w3734:string)
            n1388 = Number To Decimal String(number=w3739, width (-)=w3732) -> (decimal integer string=w3735:string)
            n1389 = Concatenate Strings(w3738, w3737, w3736, w3733, w3734, w3735) -> (w3731:string)
            n1390 = call <vilib>:"Space Constant.vi"() -> ("String"=w3727:string)
            n1391 = Search and Replace String(replace all?=TRUE ("replace all? (F)"), input string=w3731, search string=w3727, replace string="0" ("replace string (\"\")"), error in=w3730) -> (result string=w3725:string, error out=w3729:errorcluster)  [unwired: 3 in, 2 out]
            n1392 = local read "Save Path"() -> (w3752:path)
            n1393 = Path To String(path=w3752) -> (string=w3751:string)
            n1394 = Concatenate Strings(w3751, "\\" ("string"), "Analysis_", w3725, ".png" ("string")) -> (w3750:string)
            n1395 = property on="ScanImage"(error in=w3729) -> (error out=w3754:errorcluster, "User Palette"=w3753)  [unwired: 1 in, 1 out]
            n1396 = String To Path(string=w3750) -> (path=w3749:path)
            n1397 = local read "ScanImage"() -> (w3756:T3)
            n1398 = call-poly "IMAQ Write File 2"("Color Palette"=w3753, "error in (no error)"=w3754, "Image Quality"=u32 1000, "File Path"=w3749, "Image"=w3756) -> ("error out"=w3720:errorcluster)  [unwired: 5 in, 1 out]
            n1399 = invoke on="Save Analysis button" class="Bool" method="Reinit To Default"() -> (error out=w3719:errorcluster)  [unwired: 3 in, 2 out]
            n1400 = Merge Errors(w3720, w3719) -> (w3721:errorcluster)
          }
          event "Network Transport": Value Change {
            n1401 = event-data() -> ("NewVal"=w3763:enum32{"Radio Selection 1", "Radio Selection 2"})  [unwired: 1 in, 4 out]
            n1402 = disable-structure shown="Enabled" {
              disable-tunnel: w3764 -> [w3787 w3814]
              disable-tunnel: w3763 -> [w3783 _]
              disable-tunnel: w3762 -> [w3782 w3815]
              disable-tunnel: [w3781 w3815] -> w3761
              disable-tunnel: [w3780 w3814] -> w3760
              disable-tunnel: w3759 -> [w3779 _]
              frame Disabled {
                n1403 = case shown="\"Radio Selection 1\", Default" w3783 {
                  tunnel: [FALSE TRUE] -> w3765
                  tunnel: [T21."Enabled" ("Disabled") T21."Disabled and Grayed Out" ("Disabled")] -> w3771
                  frame "Radio Selection 1", Default {
                  }
                  frame "Radio Selection 2" {
                  }
                }
                n1404 = property on="Analysis Mode" class="Enum (strict)"(error in=w3787, "DisabledEnum"=w3771) -> (error out=w3786:errorcluster)  [unwired: 1 in, 1 out]
                n1405 = property on="Save Analysis button" class="Bool"(error in=w3786, "DisabledEnum"=w3771) -> (error out=w3785:errorcluster)  [unwired: 1 in, 1 out]
                n1406 = Concatenate Strings("_Image" ("string")) -> (w3773:string)  [unwired: 1 in]
                n1407 = case shown="\"Radio Selection 1\", Default" w3783 {
                  tunnel: [w3791 w3806] -> w3784
                  tunnel: w3782 -> [_ w3805]
                  tunnel: [w3790 w3804] -> w3772
                  tunnel: [w3789 _] -> w3781
                  tunnel: w3773 -> [w3788 _]
                  frame "Radio Selection 1", Default {
                    n1408 = for {
                      shift-right: [w3802] -> w3790
                      shift-left: w3791 -> [w3803]
                      tunnel: [w3801] -> w3789 mode=indexing
                      tunnel: w3788 -> [w3792]
                      i -> [w3794]
                      w3800 = T22 4 items=["ONCE_ONLY"=1, "TIMED"=2, "MONITORED"=4] ("serviceType")
                      n1409 = Increment(x=w3794) -> (x+1=w3796:i32)
                      n1410 = Number To Decimal String(number=w3796) -> (decimal integer string=w3795:string)  [unwired: 1 in]
                      n1411 = Concatenate Strings(w3792, "_", w3795) -> (w3793:string)
                      n1412 = call-poly "LVDimInterface.dic_info_service.vi"("serviceName"=w3793, "timeout [s]"=0, "serviceType"=w3800, "error in (no error)"=w3803, "stamped"=FALSE) -> ("callBackID"=w3801:i32, "error out"=w3802:errorcluster)  [unwired: 13 in]
                    }
                  }
                  frame "Radio Selection 2" {
                    n1413 = for {
                      tunnel: w3805 -> [w3807] mode=indexing
                      shift-right: [w3808] -> w3804
                      shift-left: w3806 -> [w3809]
                      n1414 = call "LVDimInterface.dic_release_service.vi"("callBackID"=w3807, "error in (no error)"=w3809) -> ("error out"=w3808:errorcluster)  [unwired: 17 in]
                    }
                  }
                }
                n1415 = local read "Select Camera"() -> (w3770:u16)
                n1416 = Boolean To (0,1)(Boolean=w3765) -> (0, 1=w3778:i16)
                n1417 = call-poly "CoreLib.data 2 byte array.vi"("i16"=w3778) -> ("byteArray out"=w3775:T26)  [unwired: 18 in]
                n1418 = Unbundle By Name() -> ("Cameras"=w3767:T35)  [unwired: 1 in]
                n1419 = call "BaseProcess.call process 2.vi"("i ref in"=w3779, "Selector"="SetJpgMode", "Data Descriptor"="S:1", "Data"=w3775, "error in (no error)"=w3772) -> ("error out"=w3780:errorcluster)  [unwired: 13 in, 1 out]
                n1420 = Index Array(array=w3767, index=w3770) -> (element=w3768:T36)
                n1421 = Bundle By Name(cluster=w3768, "JPEG Mode?"=w3765) -> (w3766:T36)
                n1422 = Replace Array Subset(array=w3767, new element=w3766, index=w3770) -> (w3769:T35)
                n1423 = Bundle By Name("Cameras"=w3769) -> ()  [unwired: 1 in, 1 out]
              }
              frame Enabled {
              }
            }
          }
          event "Delay (ms)": Value Change {
            n1424 = event-data() -> ("OldVal"=w3818:i32, "NewVal"=w3817:i32)  [unwired: 1 in, 3 out]
            n1425 = Greater?(x=w3817, y=1000) -> (0:w3819:bool)
            n1426 = case shown="False" w3819 {
              tunnel: w3818 -> [w3827 _]
              tunnel: w3817 -> [_ w3828]
              frame False {
                n1427 = local write "Delay (ms)"(w3827) -> ()
                n1428 = Concatenate Strings("Please enter a value" ("message"), "\r", "larger than 1000ms!" ("message")) -> (w3826:string)
                n1429 = One Button Dialog(message=w3826) -> ()  [unwired: 1 in, 1 out]
              }
              frame True {
                n1430 = local write "Delay (ms) Buffered"(w3828) -> ()
              }
            }
          }
          event "Acquisition mode": Value Change {
            n1431 = event-data() -> ("OldVal"=w3829:T2, "NewVal"=w3831:T2)  [unwired: 1 in, 3 out]
            n1432 = stacked-sequence {
              tunnel: [_ w3874] -> w3834
              tunnel: w3833 -> [w3837 w3873]
              tunnel: w3832 -> [w3838 w3872]
              tunnel: w3831 -> [w3840 w3856]
              tunnel: w3829 -> [w3839 _]
              frame #0 {
                # "Switch off sequencer when another acquisition mode is selected"
                n1433 = case shown="\"Scan\"" w3840 {
                  tunnel: w3839 -> [w3845 _]
                  tunnel: w3838 -> [w3843 _]
                  tunnel: w3837 -> [w3842 _]
                  tunnel: [T21."Disabled and Grayed Out" ("Disabled") T21."Enabled" ("Disabled")] -> w3836
                  frame "Internal Trigger", "free Running", "External Trigger", Default {
                    n1434 = case shown="\"Scan\"" w3845 {
                      tunnel: w3843 -> [_ w3847]
                      tunnel: w3842 -> [_ w3846]
                      frame "Internal Trigger", "free Running", "External Trigger", Default {
                      }
                      frame "Scan" {
                        n1435 = call "IMAQController.get i attribute.vi"("i ref in"=w3847, "error in (no error)"=w3846) -> ("i ref out"=w3849:refnum<vi>, "i attribute"=w3851:T17, "error out"=w3850:errorcluster)  [unwired: 15 in]
                        n1436 = Unbundle By Name(w3851) -> ("actSequencer"=w3848:string)
                        n1437 = call "BaseProcess.call process 2.vi"("i ref in"=w3849, "Object"=w3848, "Selector"="Abort", "error in (no error)"=w3850) -> ()  [unwired: 14 in, 2 out]
                      }
                    }
                    n1438 = local write "ScanRunning?"(FALSE ("ScanRunning?")) -> ()
                  }
                  frame "Scan" {
                  }
                }
                n1439 = property on="auto repeat scan step" class="Bool (strict)"("DisabledEnum"=w3836) -> ()  [unwired: 2 in, 2 out]
                n1440 = property on="lower limit" class="DigNum (strict)"("DisabledEnum"=w3836) -> ()  [unwired: 2 in, 2 out]
                n1441 = property on="Progress bar" class="Slide (strict)"("DisabledEnum"=w3836) -> ()  [unwired: 2 in, 2 out]
                n1442 = property on="ScanRunning?" class="Bool (strict)"("DisabledEnum"=w3836) -> ()  [unwired: 2 in, 2 out]
              }
              frame #1 {
                # "Camera Trigger Mode"
                n1443 = call "IMAQController.get i attribute.vi"("i ref in"=w3872, "error in (no error)"=w3873) -> ("i ref out"=w3871:refnum<vi>, "i attribute"=w3870:T17, "error out"=w3865:errorcluster)  [unwired: 15 in]
                n1444 = Unbundle By Name(w3870) -> ("actCamera"=w3855:string, "CameraTriggerID"=w3869:i32)
                n1445 = case shown="\"Scan\"" w3856 {
                  tunnel: [0 1 1] -> w3867
                  tunnel: [T21."Enabled" ("Disabled") T21."Disabled and Grayed Out" ("Disabled") T21."Disabled and Grayed Out" ("Disabled")] -> w3863
                  frame Default {
                  }
                  frame "Scan" {
                  }
                  frame "External Trigger" {
                  }
                }
                n1446 = property on="Delay (ms)" class="DigNum (strict)"(error in=w3865, "DisabledEnum"=w3863) -> (error out=w3864:errorcluster)  [unwired: 1 in, 1 out]
                n1447 = case shown="Default" w3856 {
                  tunnel: w3864 -> [w3892 w3899]
                  tunnel: [w3888 w3895] -> w3875
                  frame Default {
                    w3887 = T21."Disabled and Grayed Out" ("Disabled")
                    n1448 = property on="Configure Scan button" class="Bool"(error in=w3892, "DisabledEnum"=w3887) -> (error out=w3891:errorcluster)  [unwired: 1 in, 1 out]
                    n1449 = property on="Start Scan button" class="Bool"(error in=w3891, "DisabledEnum"=w3887) -> (error out=w3890:errorcluster)  [unwired: 1 in, 1 out]
                    n1450 = property on="Pause Scan button" class="Bool"(error in=w3890, "DisabledEnum"=w3887) -> (error out=w3889:errorcluster)  [unwired: 1 in, 1 out]
                    n1451 = property on="Stop Scan button" class="Bool"(error in=w3889, "DisabledEnum"=w3887) -> (error out=w3888:errorcluster)  [unwired: 1 in, 1 out]
                  }
                  frame "Scan" {
                    w3894 = T21."Enabled" ("Disabled")
                    n1452 = property on="Configure Scan button" class="Bool"(error in=w3899, "DisabledEnum"=w3894) -> (error out=w3898:errorcluster)  [unwired: 1 in, 1 out]
                    n1453 = property on="Start Scan button" class="Bool"(error in=w3898, "DisabledEnum"=w3894) -> (error out=w3897:errorcluster)  [unwired: 1 in, 1 out]
                    n1454 = property on="Pause Scan button" class="Bool"(error in=w3897, "DisabledEnum"=T21."Disabled and Grayed Out" ("Disabled")) -> (error out=w3896:errorcluster)  [unwired: 1 in, 1 out]
                    n1455 = property on="Stop Scan button" class="Bool"(error in=w3896, "DisabledEnum"=w3894) -> (error out=w3895:errorcluster)  [unwired: 1 in, 1 out]
                  }
                }
                n1456 = call-poly "CoreLib.data 2 byte array.vi"("i32"=w3867) -> ("byteArray out"=w3876:T26)  [unwired: 18 in]
                n1457 = To Word Integer(number=w3867) -> (16bit integer=w3868:i16)
                n1458 = Type Cast(x=w3868) -> (*(type *) &x=w3866:string)  [unwired: 1 in]
                n1459 = call "BaseProcess.call process 2.vi"("i ref in"=w3871, "Object"=w3855, "Selector"="SetTriggerMode", "Data"=w3876, "error in (no error)"=w3875) -> ("i ref out"=w3854:refnum<vi>)  [unwired: 13 in, 1 out]
                n1460 = call "LVDimInterface.dis_update_service.vi"("my_serviceID"=w3869, "data"=w3866) -> ("error out"=w3862:errorcluster)  [unwired: 15 in, 2 out]
                n1461 = call "IMAQController.get data to modify.vi"("i ref in"=w3854, "error in (no error)"=w3862) -> ("i ref out"=w3861:refnum<vi>, "i attribute"=w3857:T17, "timed out"=w3858:bool, "error out"=w3860:errorcluster)  [unwired: 14 in]
                n1462 = case shown="False" w3858 {
                  tunnel: w3861 -> [w3883 _]
                  tunnel: w3860 -> [w3882 w3884]
                  tunnel: [w3881 w3884] -> w3859
                  tunnel: w3857 -> [w3880 _]
                  tunnel: w3856 -> [w3878 _]
                  frame False {
                    n1463 = Bundle By Name(cluster=w3880, "activeCamera.Aqcuisation Mode"=w3878) -> (w3879:T17)
                    n1464 = call "IMAQController.set modified data.vi"("i ref in"=w3883, "i attribute"=w3879, "error in (no error)"=w3882) -> ("error out"=w3881:errorcluster)  [unwired: 15 in, 1 out]
                  }
                  frame True {
                  }
                }
                n1465 = flat-sequence {
                  tunnel: w3859 -> [w3886]
                  tunnel: [w3886] -> w3874
                  tunnel: w3856 -> [w3885]
                  frame #0 {
                    n1466 = local write "Acquisition mode (Buffer)"(w3885) -> ()
                  }
                }
              }
            }
          }
          event "Start Scan button": Value Change {
            n1467 = event-data() -> ("NewVal"=w3916:bool)  [unwired: 1 in]
            n1468 = case shown="True" w3916 {
              tunnel: w3915 -> [w3919 w3949]
              tunnel: [w3919 w3951] -> w3914
              tunnel: w3913 -> [_ w3947]
              tunnel: [w3918 w3955] -> w3911
              tunnel: w3912 -> [w3918 w3955]
              tunnel: w3909 -> [_ w3954]
              tunnel: w3908 -> [w3917 w3940]
              tunnel: [w3917 _] -> w3907
              tunnel: w3906 -> [_ w3920]
              frame False {
              }
              frame True {
                w3925 = T12 {"Message"="", "Error?"=TRUE, "current time"=timestamp(0 s since 1904-01-01)}  # Logger String
                w3936 = i16 2 ("width (-)")
                w3943 = T21."Enabled" ("Disabled")
                w3944 = T21."Disabled and Grayed Out" ("Disabled")
                n1469 = invoke on="Start Scan button" class="Bool" method="Reinit To Default"() -> ()  [unwired: 3 in, 3 out]
                n1470 = Get Date/Time In Seconds() -> (seconds since 1Jan1904=w3923:timestamp)
                n1471 = Bundle By Name(cluster=w3925, "Message"="Scan started", "Error?"=FALSE, "current time"=w3923) -> (w3921:T12)
                n1472 = Generate User Event(user event=w3920, event data cluster=w3921) -> ()  [unwired: 2 in, 2 out]
                n1473 = property on="Start Scan button" class="Bool"("DisabledEnum"=w3944) -> ()  [unwired: 2 in, 2 out]
                n1474 = property on="Configure Scan button" class="Bool"("DisabledEnum"=w3944) -> ()  [unwired: 2 in, 2 out]
                n1475 = call "IMAQController.get i attribute.vi"("i ref in"=w3947, "error in (no error)"=w3949) -> ("i ref out"=w3946:refnum<vi>, "i attribute"=w3950:T17, "error out"=w3948:errorcluster)  [unwired: 15 in]
                n1476 = Unbundle By Name(w3950) -> ("actSequencer"=w3945:string)
                n1477 = property on="Pause Scan button" class="Bool"("DisabledEnum"=w3943) -> ()  [unwired: 2 in, 2 out]
                n1478 = property on="Stop Scan button" class="Bool"("DisabledEnum"=w3943) -> ()  [unwired: 2 in, 2 out]
                n1479 = call "BaseProcess.call process 2.vi"("i ref in"=w3946, "Object"=w3945, "Selector"="Start", "error in (no error)"=w3948) -> ("error out"=w3952:errorcluster)  [unwired: 14 in, 1 out]
                n1480 = Not(x=w3940) -> (.not. x?=w3941:bool)
                n1481 = Generate User Event(user event=w3954, event data cluster=w3941, error in=w3952) -> (error out=w3951:errorcluster)  [unwired: 1 in, 1 out]
                n1482 = Get Date/Time In Seconds() -> (seconds since 1Jan1904=w3931:timestamp)
                n1483 = local write "ScanRunning?"(TRUE ("ScanRunning?")) -> ()
                n1484 = Seconds To Date/Time(time stamp (now)=w3931) -> (date time rec=w3932:T34)  [unwired: 1 in]
                n1485 = Unbundle By Name(w3932) -> ("hour"=w3933:i32, "minute"=w3934:i32, "second"=w3935:i32)
                n1486 = Number To Decimal String(number=w3933, width (-)=w3936) -> (decimal integer string=w3937:string)
                n1487 = Number To Decimal String(number=w3934, width (-)=w3936) -> (decimal integer string=w3938:string)
                n1488 = Number To Decimal String(number=w3935, width (-)=w3936) -> (decimal integer string=w3939:string)
                n1489 = Concatenate Strings(w3937, w3938, w3939) -> (w3927:string)
                n1490 = call <vilib>:"Space Constant.vi"() -> ("String"=w3930:string)
                n1491 = Search and Replace String(replace all?=TRUE ("replace all? (F)"), input string=w3927, search string=w3930, replace string="0" ("replace string (\"\")")) -> (result string=→"Last scan started":string)  [unwired: 4 in, 3 out]
              }
            }
          }
          event "Pause Scan button": Value Change {
            n1492 = event-data() -> ("NewVal"=w3964:bool)  [unwired: 1 in, 4 out]
            n1493 = case shown="True" w3964 {
              tunnel: w3963 -> [w3967 w3976]
              tunnel: [w3967 w3978] -> w3962
              tunnel: w3961 -> [_ w3974]
              tunnel: [w3966 w3980] -> w3959
              tunnel: w3960 -> [w3966 w3980]
              tunnel: w3957 -> [w3965 _]
              tunnel: [w3965 TRUE ("Paused scan?")] -> w3956
              frame False {
              }
              frame True {
                w3970 = T21."Disabled and Grayed Out" ("Disabled")
                w3971 = T21."Enabled" ("Disabled")
                n1494 = invoke on="Pause Scan button" class="Bool" method="Reinit To Default"() -> ()  [unwired: 3 in, 3 out]
                n1495 = call "IMAQController.get i attribute.vi"("i ref in"=w3974, "error in (no error)"=w3976) -> ("i ref out"=w3973:refnum<vi>, "i attribute"=w3977:T17, "error out"=w3975:errorcluster)  [unwired: 15 in]
                n1496 = Unbundle By Name(w3977) -> ("actSequencer"=w3972:string)
                n1497 = property on="Start Scan button" class="Bool"("DisabledEnum"=w3971) -> ()  [unwired: 2 in, 2 out]
                n1498 = property on="Stop Scan button" class="Bool"("DisabledEnum"=w3971) -> ()  [unwired: 2 in, 2 out]
                n1499 = call "BaseProcess.call process 2.vi"("i ref in"=w3973, "Object"=w3972, "Selector"="Pause", "error in (no error)"=w3975) -> ("error out"=w3978:errorcluster)  [unwired: 14 in, 1 out]
                n1500 = property on="Pause Scan button" class="Bool"("DisabledEnum"=w3970) -> ()  [unwired: 2 in, 2 out]
                n1501 = property on="Configure Scan button" class="Bool"("DisabledEnum"=w3970) -> ()  [unwired: 2 in, 2 out]
                n1502 = local write "ScanRunning?"(FALSE ("ScanRunning?")) -> ()
              }
            }
          }
          event "Stop Scan button": Value Change {
            n1503 = event-data() -> ("NewVal"=w3989:bool)  [unwired: 1 in, 4 out]
            n1504 = case shown="True" w3989 {
              tunnel: w3988 -> [w3992 w4001]
              tunnel: [w3992 w3993] -> w3987
              tunnel: w3986 -> [_ w3999]
              tunnel: [w3991 w4004] -> w3984
              tunnel: w3985 -> [w3991 w4004]
              tunnel: w3982 -> [w3990 _]
              tunnel: [w3990 _] -> w3981
              frame False {
              }
              frame True {
                w3995 = T21."Disabled and Grayed Out" ("Disabled")
                w3996 = T21."Enabled" ("Disabled")
                n1505 = invoke on="Stop Scan button" class="Bool" method="Reinit To Default"() -> ()  [unwired: 3 in, 3 out]
                n1506 = call "IMAQController.get i attribute.vi"("i ref in"=w3999, "error in (no error)"=w4001) -> ("i ref out"=w3998:refnum<vi>, "i attribute"=w4002:T17, "error out"=w4000:errorcluster)  [unwired: 15 in]
                n1507 = Unbundle By Name(w4002) -> ("actSequencer"=w3997:string)
                n1508 = property on="Start Scan button" class="Bool"("DisabledEnum"=w3996) -> ()  [unwired: 2 in, 2 out]
                n1509 = property on="Configure Scan button" class="Bool"("DisabledEnum"=w3996) -> ()  [unwired: 2 in, 2 out]
                n1510 = call "BaseProcess.call process 2.vi"("i ref in"=w3998, "Object"=w3997, "Selector"="Abort", "error in (no error)"=w4000) -> ("error out"=w3993:errorcluster)  [unwired: 14 in, 1 out]
                n1511 = property on="Stop Scan button" class="Bool"("DisabledEnum"=w3995) -> ()  [unwired: 2 in, 2 out]
                n1512 = property on="Pause Scan button" class="Bool"("DisabledEnum"=w3995) -> ()  [unwired: 2 in, 2 out]
                n1513 = local write "ScanRunning?"(FALSE ("ScanRunning?")) -> ()
              }
            }
          }
          event "ROI2notROI1Boolen": Value Change {
            n1514 = event-data() -> ("NewVal"=w4013:bool)  [unwired: 1 in, 4 out]
            n1515 = case shown="False" w4013 {
              tunnel: [T21."Enabled" ("Disabled") T21."Disabled and Grayed Out" ("Disabled")] -> w4007
              frame False {
              }
              frame True {
              }
            }
            n1516 = property on="TL2x" class="DigNum (strict)"(error in=w4012, "DisabledEnum"=w4007) -> (error out=w4011:errorcluster)  [unwired: 1 in, 1 out]
            n1517 = property on="TL2y" class="DigNum (strict)"(error in=w4011, "DisabledEnum"=w4007) -> (error out=w4010:errorcluster)  [unwired: 1 in, 1 out]
            n1518 = property on="BR2x" class="DigNum (strict)"(error in=w4010, "DisabledEnum"=w4007) -> (error out=w4009:errorcluster)  [unwired: 1 in, 1 out]
            n1519 = property on="BR2y" class="DigNum (strict)"(error in=w4009, "DisabledEnum"=w4007) -> (error out=w4008:errorcluster)  [unwired: 1 in, 1 out]
          }
          event "Send Button": Value Change {
            n1520 = event-data() -> ("NewVal"=w4016:bool)  [unwired: 1 in]
            n1521 = case shown="True" w4016 {
              tunnel: w4018 -> [w4022 w4024]
              tunnel: [w4022 w4023] -> w4017
              frame False {
              }
              frame True {
                n1522 = stacked-sequence {
                  seq-local: [w4027 _] -> [_ w4135]
                  seq-local: [w4026 _] -> [_ w4134]
                  tunnel: w4024 -> [w4032 _]
                  tunnel: [w4028 _] -> w4023
                  frame #0 {
                    n1523 = local read "BugFilePath"() -> (w4031:path)
                    n1524 = call <vilib>:"Open Config Data.vi"("error in (no error)"=w4032, "configuration file path"=w4031) -> ("error out"=w4033:errorcluster, "refnum"=w4034:T20)  [unwired: 7 in, 1 out]
                    n1525 = call <vilib>:"Get Section Names.vi"("error in (no error)"=w4033, "refnum"=w4034) -> ("error out"=w4036:errorcluster, "section names"=w4035:string[], "refnum out"=w4025:T20)  [unwired: 7 in]
                    n1526 = for {
                      tunnel: w4035 -> [w4085] mode=indexing
                      tunnel: w4025 -> [w4099]
                      shift-right: [w4084] -> w4030
                      shift-left: w4036 -> [w4100]
                      tunnel: [w4075] -> w4026 mode=indexing
                      n1527 = call-poly <vilib>:"Read Key.vi"("section"=w4085, "error in (no error)"=w4100, "key"="B?", "refnum"=w4099) -> ("error out"=w4097:errorcluster, "value"=w4083:bool, "refnum out"=w4098:T20)  [unwired: 4 in, 1 out]
                      n1528 = Select(t="B", s=w4083, f="F") -> (s? t:f=w4080:string)
                      n1529 = call-poly <vilib>:"Read Key.vi"("section"=w4085, "error in (no error)"=w4097, "key"="Date", "refnum"=w4098) -> ("error out"=w4088:errorcluster, "value"=w4079:string, "refnum out"=w4090:T20)  [unwired: 4 in, 1 out]
                      n1530 = call-poly <vilib>:"Read Key.vi"("section"=w4085, "error in (no error)"=w4088, "key"="User", "refnum"=w4090) -> ("error out"=w4086:errorcluster, "value"=w4078:string, "refnum out"=w4087:T20)  [unwired: 4 in, 1 out]
                      n1531 = call-poly <vilib>:"Read Key.vi"("section"=w4085, "error in (no error)"=w4086, "key"="Topic", "refnum"=w4087) -> ("error out"=w4095:errorcluster, "value"=w4077:string, "refnum out"=w4096:T20)  [unwired: 4 in, 1 out]
                      n1532 = call-poly <vilib>:"Read Key.vi"("section"=w4085, "error in (no error)"=w4095, "key"="Desc", "refnum"=w4096) -> ("error out"=w4084:errorcluster, "value"=w4076:string)  [unwired: 4 in, 2 out]
                      n1533 = Build Array(w4080, w4079, w4078, w4077, w4076) -> (w4075:string[])
                    }
                    n1534 = property on="Bug Report/ Feature Request - List" class="MCListbox (strict)"() -> ("ItemNames"=w4027:string[][])  [unwired: 2 in, 2 out]
                    n1535 = for {
                      tunnel: w4027 -> [w4040] mode=indexing
                      tunnel: w4025 -> [w4045]
                      shift-right: [w4042] -> w4029
                      shift-left: w4030 -> [w4044]
                      tunnel: [w4043] -> _
                      i -> [w4041]
                      n1536 = Concatenate Strings(w4040) -> (w4039:string)
                      n1537 = Equal?(x=w4039, y="") -> (x = y?=w4038:bool)
                      n1538 = case shown="False" w4038 {
                        tunnel: w4040 -> [w4072 _]
                        tunnel: w4045 -> [w4071 w4074]
                        tunnel: w4044 -> [w4070 w4073]
                        tunnel: [w4069 w4074] -> w4043
                        tunnel: [w4068 w4073] -> w4042
                        tunnel: w4041 -> [w4067 _]
                        frame False {
                          n1539 = Index Array(array=w4072) -> (element #1=w4066:string, element #2=w4055:string, element #3=w4054:string, element #4=w4053:string, element #5=w4052:string)  [unwired: 5 in]
                          n1540 = Equal?(x="B", y=w4066) -> (x = y?=w4064:bool)
                          n1541 = Number To Decimal String(number=w4067) -> (decimal integer string=w4051:string)  [unwired: 1 in]
                          n1542 = call-poly <vilib>:"Write Key.vi"("section"=w4051, "error in (no error)"=w4070, "value"=w4064, "key"="B?", "refnum"=w4071) -> ("error out"=w4062:errorcluster, "refnum out"=w4063:T20)  [unwired: 4 in, 1 out]
                          n1543 = call-poly <vilib>:"Write Key.vi"("section"=w4051, "error in (no error)"=w4062, "value"=w4055, "key"="Date", "refnum"=w4063) -> ("error out"=w4060:errorcluster, "refnum out"=w4061:T20)  [unwired: 4 in, 1 out]
                          n1544 = call-poly <vilib>:"Write Key.vi"("section"=w4051, "error in (no error)"=w4060, "value"=w4054, "key"="User", "refnum"=w4061) -> ("error out"=w4058:errorcluster, "refnum out"=w4059:T20)  [unwired: 4 in, 1 out]
                          n1545 = call-poly <vilib>:"Write Key.vi"("section"=w4051, "error in (no error)"=w4058, "value"=w4053, "key"="Topic", "refnum"=w4059) -> ("error out"=w4056:errorcluster, "refnum out"=w4057:T20)  [unwired: 4 in, 1 out]
                          n1546 = call-poly <vilib>:"Write Key.vi"("section"=w4051, "error in (no error)"=w4056, "value"=w4052, "key"="Desc", "refnum"=w4057) -> ("error out"=w4068:errorcluster, "refnum out"=w4069:T20)  [unwired: 4 in, 1 out]
                        }
                        frame True {
                        }
                      }
                    }
                    n1547 = call <vilib>:"Close Config Data.vi"("error in (no error)"=w4029, "refnum"=w4025) -> ("error out"=w4028:errorcluster)  [unwired: 8 in, 1 out]
                  }
                  frame #1 {
                    # "alt"
                    # "neu"
                    n1548 = for {
                      tunnel: w4134 -> [w4153] mode=indexing
                      tunnel: [w4152] -> w4133 mode=indexing
                      n1549 = Concatenate Strings(w4153) -> (w4152:string)
                    }
                    n1550 = for {
                      tunnel: w4135 -> [w4155] mode=indexing
                      tunnel: w4133 -> [w4158]
                      tunnel: [w4155] -> w4109 mode=indexing if=w4154
                      n1551 = Concatenate Strings(w4155) -> (w4157:string)
                      n1552 = Search 1D Array(1D array=w4158, element=w4157) -> (index of element=w4156:i32)  [unwired: 1 in]
                      n1553 = Less Than 0?(x=w4156) -> (x < 0?=w4154:bool)
                    }
                    n1554 = for {
                      tunnel: w4109 -> [w4151] mode=indexing
                      tunnel: [w4144] -> w4111 mode=indexing
                      tunnel: [w4139] -> w4102 mode=indexing
                      w4140 = "\r\n"
                      n1555 = Index Array(array=w4151) -> (element #1=w4150:string, element #2=w4143:string, element #3=w4142:string, element #4=w4139:string, element #5=w4141:string)  [unwired: 5 in]
                      n1556 = Equal?(x="B", y=w4150) -> (x = y?=w4148:bool)
                      n1557 = Select(t="Bug report:" ("x"), s=w4148, f="Feature request:" ("x")) -> (s? t:f=w4145:string)
                      n1558 = Build Array(w4145, w4140, w4143, w4140, w4142, w4140, w4139, w4140, w4141, w4140, w4140) -> (w4144:string[])
                    }
                    n1559 = Array Size(array=w4109) -> (size(s)=w4108:i32[])
                    n1560 = Index Array(array=w4108) -> (element=w4107:i32)  [unwired: 1 in]
                    n1561 = Greater Than 0?(x=w4107) -> (x > 0?=w4104:bool)
                    n1562 = Index Array(array=w4102) -> (element=w4101:string)  [unwired: 1 in]
                    n1563 = Not Equal?(x=w4101, y="") -> (x != y?=w4105:bool)
                    n1564 = And(x=w4105, y=w4104) -> (x .and. y?=w4103:bool)
                    n1565 = Concatenate Strings(w4111) -> (w4117:string)
                    n1566 = constructor class="MailAddress"("address"="hitrap@gsi.de", "displayName"="Hitrap") -> (reference out=w4132:refnum<k24>)  [unwired: 3 in, 4 out]
                    n1567 = constructor class="MailAddress"("address"="d.neidherr@gsi.de", "displayName"="Neidherr, Dennis Dr.") -> (reference out=w4131:refnum<k24>)  [unwired: 3 in, 4 out]
                    n1568 = constructor class="MailMessage"("from"=w4132, "to"=w4131) -> (reference out=w4130:refnum<k24>)  [unwired: 3 in, 4 out]
                    n1569 = constructor class="SmtpClient"("host"="smtp.gsi.de") -> (reference out=w4128:refnum<k24>)  [unwired: 3 in, 3 out]
                    n1570 = constructor class="NetworkCredential"("userName"="hitrap", "password"="CK03032010") -> (reference out=w4120:refnum<k24>)  [unwired: 3 in, 4 out]
                    n1571 = property class="SmtpClient"(reference=w4128, "Port"=25) -> (reference out=w4119:refnum<k24>)  [unwired: 1 in, 1 out]
                    n1572 = property class="MailMessage"(reference=w4130, "Subject"="IMAQController: New Bug/Feature") -> (reference out=w4129:refnum<k24>)  [unwired: 1 in, 1 out]
                    n1573 = property class="SmtpClient"(reference=w4119, "Credentials"=w4120) -> (reference out=w4127:refnum<k24>)  [unwired: 1 in, 1 out]
                    n1574 = property class="MailMessage"(reference=w4129, "Body"=w4117) -> (reference out=w4121:refnum<k24>)  [unwired: 1 in, 1 out]
                    n1575 = property class="SmtpClient"(reference=w4127, "EnableSsl"=FALSE) -> (reference out=w4110:refnum<k24>)  [unwired: 1 in, 1 out]
                    n1576 = case shown="True" w4103 {
                      tunnel: w4121 -> [_ w4138]
                      tunnel: "Thank you for your good will to improve this software.\nYou have just sent an email to a poor guy who has now more work.\nThanks a lot again..." ("message") -> [_ w4137]
                      tunnel: w4110 -> [_ w4136]
                      frame False {
                      }
                      frame True {
                        n1577 = invoke class="SmtpClient" method="Send"(reference=w4136, "message"=w4138) -> ()  [unwired: 2 in, 4 out]
                        n1578 = One Button Dialog(message=w4137) -> ()  [unwired: 1 in, 1 out]
                      }
                    }
                  }
                }
              }
            }
            n1579 = local write "Send Button"(FALSE ("Send Button")) -> ()
          }
          event "Bug Report/ Feature Request - List": Value Change {
            n1580 = event-data() -> ()  [unwired: 1 in, 1 out]
            n1581 = property on="Bug Report/ Feature Request - List" class="MCListbox (strict)"() -> ("ItemNames"=w4159:string[][])  [unwired: 2 in, 2 out]
            n1582 = Array Size(array=w4159) -> (size(s)=w4165:i32[])
            n1583 = Index Array(array=w4165) -> (element=w4164:i32)  [unwired: 1 in]
            n1584 = Decrement(x=w4164) -> (x-1=w4163:i32)
            n1585 = Index Array(array=w4159, index (row)=w4163) -> (element=w4162:string[])  [unwired: 1 in]
            n1586 = for {
              tunnel: w4162 -> [w4171] mode=indexing
              tunnel: [w4169] -> w4161 mode=indexing
              n1587 = Equal?(x="", y=w4171) -> (x = y?=w4169:bool)
            }
            n1588 = And Array Elements(Boolean array=w4161) -> (logical AND=w4160:bool)
            n1589 = case shown="False" w4160 {
              tunnel: w4159 -> [w4172 _]
              frame False {
                n1590 = Initialize Array("", 5 ("dimension size")) -> (w4173:string[])
                n1591 = Build Array (concatenate)(w4172, w4173) -> (w4176:string[][])
                n1592 = property on="Bug Report/ Feature Request - List" class="MCListbox (strict)"("ItemNames"=w4176) -> ()  [unwired: 2 in, 2 out]
              }
              frame True {
              }
            }
          }
          event "Error UL": Mouse Down {
            n1593 = event-data() -> ()  [unwired: 1 in, 7 out]
            n1594 = local read "Error UL"() -> (w4178:bool)
            n1595 = case shown="True" w4178 {
              tunnel: [w4184 w4189] -> w4183
              tunnel: w4182 -> [_ w4188]
              tunnel: w4181 -> [w4184 w4185]
              frame False {
              }
              frame True {
                # "UL traegt die ID 0"
                n1596 = invoke on="Error UL" class="Bool (strict)" method="Reinit To Default"(error in=w4185) -> (error out=w4186:errorcluster)  [unwired: 2 in, 2 out]
                n1597 = Send Notification(notification=0, notifier=w4188, error in (no error)=w4186) -> (error out=w4189:errorcluster)  [unwired: 1 out]
              }
            }
          }
          event "Error UR": Mouse Down {
            n1598 = event-data() -> ()  [unwired: 1 in, 7 out]
            n1599 = local read "Error UR"() -> (w4191:bool)
            n1600 = case shown="True" w4191 {
              tunnel: [w4197 w4202] -> w4196
              tunnel: w4195 -> [_ w4201]
              tunnel: w4194 -> [w4197 w4198]
              frame False {
              }
              frame True {
                # "UR traegt die ID 1"
                n1601 = invoke on="Error UR" class="Bool (strict)" method="Reinit To Default"(error in=w4198) -> (error out=w4199:errorcluster)  [unwired: 2 in, 2 out]
                n1602 = Send Notification(notification=1, notifier=w4201, error in (no error)=w4199) -> (error out=w4202:errorcluster)  [unwired: 1 out]
              }
            }
          }
        }
        n1603 = local write "User Event error out"(w3234) -> ()
      }
      frame True {
        n1604 = event shown="[2] \"Error OL\": Mouse Down" {
          selector: w4209 -> [_ _ _ _]
          dyn-events: _ -> [_ _ _ _]
          timeout: -1 -> [_ _ _ _]
          tunnel: w4210 -> [w4213 w4214 _ _]
          tunnel: [w4212 w4215 w4220 w4227] -> w4207
          tunnel: [_ TRUE _ _] -> w4206
          tunnel: w4205 -> [w4212 w4215 w4219 w4228]
          tunnel: [w4213 w4214 FALSE FALSE] -> w4204
          tunnel: w4203 -> [_ _ _ w4226]
          event Timeout {
            n1605 = event-data() -> ()  [unwired: 1 in, 2 out]
          }
          event User Event {
            n1606 = event-data() -> ()  [unwired: 1 in, 4 out]
          }
          event "Error OL": Mouse Down {
            n1607 = event-data() -> ()  [unwired: 1 in, 7 out]
            n1608 = local read "Error OL"() -> (w4217:bool)
            n1609 = case shown="True" w4217 {
              tunnel: [w4221 w4223] -> w4220
              tunnel: w4219 -> [w4221 w4222]
              frame False {
              }
              frame True {
                n1610 = call <vilib>:"Clear Errors.vi"("error in (no error)"=w4222) -> ("error out"=w4224:errorcluster)  [unwired: 5 in, 1 out]
                n1611 = invoke on="Error OL" class="Bool (strict)" method="Reinit To Default"(error in=w4224) -> (error out=w4223:errorcluster)  [unwired: 2 in, 2 out]
              }
            }
          }
          event "Error UL": Mouse Down {
            n1612 = event-data() -> ()  [unwired: 1 in, 7 out]
            n1613 = local read "Error UL"() -> (w4225:bool)
            n1614 = case shown="True" w4225 {
              tunnel: w4228 -> [w4230 w4234]
              tunnel: [w4230 w4232] -> w4227
              tunnel: w4226 -> [_ w4231]
              frame False {
              }
              frame True {
                # "UL traegt die ID 0"
                n1615 = invoke on="Error UL" class="Bool (strict)" method="Reinit To Default"(error in=w4234) -> (error out=w4233:errorcluster)  [unwired: 2 in, 2 out]
                n1616 = Send Notification(notification=0, notifier=w4231, error in (no error)=w4233) -> (error out=w4232:errorcluster)  [unwired: 1 out]
              }
            }
          }
        }
      }
    }
    "User Event Loop" <- w3228
  }
  n1617 = Release Queue(queue=w29) -> ()  [unwired: 2 in, 3 out]
  n1618 = call "IMAQ Dispose"("Image"=w121, "error in (no error)"=w123) -> ("error out"=w122:errorcluster)  [unwired: 1 in, 3 out]
  n1619 = call "IMAQ Dispose"("Image"=w165, "error in (no error)"=w159) -> ("error out"=w149:errorcluster)  [unwired: 1 in, 3 out]
  n1620 = stacked-sequence {
    seq-local: [w4238 _] -> [_ w4266]
    tunnel: w179 -> [w4261 _]
    tunnel: w142 -> [w4260 _]
    tunnel: [_ w4269] -> w158
    tunnel: w157 -> [w4259 _]
    tunnel: w156 -> [w4257 _]
    tunnel: w35 -> [w4255 _]
    tunnel: w1 -> [w4253 _]
    tunnel: w41 -> [w4251 _]
    tunnel: w132 -> [w4249 _]
    tunnel: w42 -> [w4248 _]
    tunnel: w112 -> [w4246 _]
    tunnel: w3 -> [w4244 _]
    tunnel: w71 -> [w4242 _]
    tunnel: w64 -> [_ w4267]
    tunnel: w46 -> [w4240 _]
    tunnel: w39 -> [w4237 _]
    frame #0 {
      n1621 = call "IMAQ Dispose"("Image"=w4257, "error in (no error)"=w4259) -> ("error out"=w4258:errorcluster)  [unwired: 1 in, 3 out]
      n1622 = for {
        tunnel: w4261 -> [w4265] mode=indexing
        tunnel: w4260 -> [w4263] mode=indexing
        shift-right: [w4264] -> w4256
        shift-left: w4258 -> [w4262]
        n1623 = Release Queue(queue=w4265, error in (no error)=w4262) -> (error out=w4264:errorcluster)  [unwired: 1 in, 2 out]
        n1624 = call "LVDimInterface.dic_release_service.vi"("callBackID"=w4263) -> ()  [unwired: 18 in, 1 out]
      }
      n1625 = Destroy User Event(user event=w4255, error in=w4256) -> (error out=w4254:errorcluster)
      n1626 = Destroy User Event(user event=w4253, error in=w4254) -> (error out=w4252:errorcluster)
      n1627 = Destroy User Event(user event=w4251, error in=w4252) -> (error out=w4250:errorcluster)
      n1628 = Release Notifier(notifier=w4249, error in (no error)=w4250) -> (error out=w4236:errorcluster)  [unwired: 1 in, 2 out]
      n1629 = Destroy User Event(user event=w4248, error in=w4236) -> (error out=w4247:errorcluster)
      n1630 = Destroy User Event(user event=w4246, error in=w4247) -> (error out=w4245:errorcluster)
      n1631 = Destroy User Event(user event=w4244, error in=w4245) -> (error out=w4243:errorcluster)
      n1632 = Destroy User Event(user event=w4242, error in=w4243) -> (error out=w4241:errorcluster)
      n1633 = Destroy User Event(user event=w4240, error in=w4241) -> (error out=w4239:errorcluster)
      n1634 = Destroy User Event(user event=w4237, error in=w4239) -> (error out=w4238:errorcluster)
    }
    frame #1 {
      n1635 = call "IMAQ Dispose"("Image"=w4267) -> ()  [unwired: 2 in, 4 out]
      n1636 = control-ref of="ActualImageLink(Compression Mode)"() -> (w4268:refnum<vi>)
      n1637 = call "DimIndicators.dic_release_service.vi"("controlRef"=w4268, "error in (no error)"=w4266) -> ("error out"=w4269:errorcluster)  [unwired: 17 in]
    }
  }
  n1638 = stacked-sequence {
    tunnel: w149 -> [w4271]
    tunnel: [w4271] -> w148
    tunnel: w78 -> [w4270]
    frame #0 {
      n1639 = Set Occurrence(w4270) -> ()
    }
  }
  n1640 = stacked-sequence {
    tunnel: w158 -> [_ w4285 _]
    tunnel: w79 -> [w4275 _ w4286]
    tunnel: w148 -> [_ w4284 _]
    tunnel: w155 -> [_ w4283 _]
    tunnel: w143 -> [_ w4282 _]
    tunnel: w122 -> [_ w4281 _]
    tunnel: w137 -> [_ w4280 _]
    frame #0 {
      # "Close FP of scanner and sequencer"
      n1641 = call "IMAQController.get i attribute.vi"("i ref in"=w4275) -> ("i attribute"=w4278:T17)  [unwired: 16 in, 2 out]
      n1642 = Unbundle By Name(w4278) -> ("actSequencer"=w4272:string, "actScanner"=w4279:string)
      n1643 = call "CSSystemLib.name2ref.vi"("name"=w4272) -> ("obj refnum"=w4273:refnum<vi>)
      n1644 = call "CSSystemLib.name2ref.vi"("name"=w4279) -> ("obj refnum"=w4276:refnum<vi>)
      n1645 = call "CSObj.open front panel.vi"("i ref in"=w4273, "frontPanelOpen"=FALSE ("front panel open")) -> ()  [unwired: 16 in, 2 out]
      n1646 = call "CSObj.open front panel.vi"("i ref in"=w4276, "frontPanelOpen"=FALSE ("front panel open")) -> ()  [unwired: 16 in, 2 out]
    }
    frame #1 {
      "DIM client error out" <- w4285
      "Analysis Event error out" <- w4284
      "User Event error out" <- w4283
      "Send command error out" <- w4282
      "Scan Image Pixel Value Loop error out" <- w4281
      "Horiz/Vert Chart error out" <- w4280
    }
    frame #2 {
      n1647 = call "destroy this.vi"("i ref in"=w4286, "close FP first"=TRUE) -> ()  [unwired: 17 in, 1 out]
    }
  }
